vi "WVDIAL_2_OphirPM_v2.0.vi"() -> ()   [LabVIEW 2012]
uses:
  <vilib>/DAQmx/write.llb/DAQmx Write (Digital 1D Bool NChan 1Samp 1Line).vi
  <vilib>/DAQmx/miscellaneous.llb/DAQmx Fill In Error Info.vi
  under_development/AMCS_Data.vi
  <vilib>/Analysis/baseanly.llb/Mean (DBL).vi
  H2O_DIAL/LabVIEW-2012/Scalar_Data.vi
  H2O_DIAL/LabVIEW-2012/Bristol WM V2_31b/CLDevIFace.dll
  <vilib>/Analysis/NI_AALBase.lvlib
panel:
  out "AMCS_Profile":i32=68875
  out "FileHour":i32=2
  out "L_Count":i32=936
  out "sigma_off_total":dbl[](array[numeric])=[5.070497628289756e-25, 5.0334853455633925e-25, 4.99663547931583e-25, 4.959948279288469e-25, 4.923423990568222e-25, 4.887062852998473e-25, 4.850865100877033e-25, 4.814830962521382e-25, 4.778960659817837e-25, 4.743254407920139e-25, 4.707712414842624e-25, 4.672334881115004e-25, 4.637121999436925e-25, 4.602073954366994e-25, 4.56719092201873e-25, 4.532473069731469e-25, 4.497920555823106e-25, 4.463533529335168e-25, 4.429312129736619e-25, 4.395256486716884e-25, 4.361366720005691e-25, 4.327642939082048e-25, 4.2940852430644775e-25, 4.260693720490288e-25, 4.227468449179839e-25, 4.194409496090374e-25, 4.161516917187555e-25, 4.128790757307133e-25, 4.0962310500914247e-25, 4.063837817890729e-25, 4.0316110716857104e-25, 3.999550811045053e-25, 3.9676570240528366e-25, 3.935929687302844e-25, 3.9043687659042657e-25, 3.872974213418959e-25, 3.8417459719034525e-25, 3.8106839719420626e-25, 3.779788132663995e-25, 3.7490583617828527e-25, 3.7184945556449563e-25, 3.6880965993136353e-25, 3.6578643666610067e-25, 3.627797720389404e-25, 3.597896512186718e-25, 3.568160582829921e-25, 3.538589762243083e-25, 3.509183869681634e-25, 3.479942713816823e-25, 3.450866092902416e-25, 3.421953794902879e-25, 3.393205597627788e-25, 3.364621268922782e-25, 3.3362005668111493e-25, 3.3079432396620512e-25, 3.2798490263459325e-25, 3.2519176564454297e-25, 3.2241488504042248e-25, 3.196542319726317e-25, 3.1690977671553114e-25, 3.1418148868557824e-25, 3.1146933646267415e-25, 3.08773287808136e-25, 3.060933096826186e-25, 3.0342936826836184e-25, 3.007814289864978e-25, 2.9814945651963276e-25, 2.955334148264468e-25, 2.9293326716696813e-25, 2.9034897611789183e-25, 2.8778050359516556e-25, 2.8522781086960743e-25, 2.8269085858893675e-25, 2.801696067964473e-25, 2.77664014947359e-25, 2.751740419295918e-25, 2.7269964608086254e-25, 2.7024078520645357e-25, 2.677974165975873e-25, 2.6536949704675698e-25, 2.629569828657932e-25, 2.6055982990165753e-25, 2.5817799355364205e-25, 2.5581142878655634e-25, 2.534600901463837e-25, 2.5112393177860403e-25, 2.488029074350094e-25, 2.464969704946346e-25, 2.4420607397132765e-25, 2.4193017053199705e-25, 2.396692125036495e-25, 2.374231518868433e-25, 2.351919403683499e-25, 2.3297552932977987e-25, 2.3077386985828024e-25, 2.2858691275833926e-25, 2.264146085578557e-25, 2.242569075179679e-25, 2.2211375964275483e-25, 2.1998511468550746e-25, 2.1787092215687626e-25, 2.1577113133082336e-25, 2.136856912540202e-25, 2.116145507460489e-25, 2.095576584136337e-25, 2.0751496264925255e-25, 2.0548641163882025e-25, 2.0347195336705433e-25, 2.0147153562078706e-25, 1.9948510599408518e-25, 1.9751261189266903e-25, 1.9555400053748722e-25, 1.936092189678544e-25, 1.9167821404641924e-25, 1.8976093246186118e-25, 1.8785732073267435e-25, 1.8596732521063013e-25, 1.840908920841047e-25, 1.8222796738212876e-25, 1.8037849697802666e-25, 1.7854242659075025e-25, 1.7671970179325255e-25, 1.7491026801307859e-25, 1.7311407053680074e-25, 1.7133105451612698e-25, 1.6956116497139343e-25, 1.6780434679580535e-25, 1.6606054476291184e-25, 1.6432970353069002e-25, 1.6261176764671616e-25, 1.6090668155595419e-25, 1.5921438960726898e-25, 1.5753483606030133e-25, 1.558679650921211e-25, 1.542137208060544e-25, 1.5257204723895893e-25, 1.5094288837202545e-25, 1.4932618813705948e-25, 1.4772189042726048e-25, 1.4612993910873613e-25, 1.4455027802681816e-25, 1.4298285102037945e-25, 1.4142760193126855e-25, 1.39884474614635e-25, 1.383534129515875e-25, 1.3683436086077352e-25, 1.3532726230945627e-25, 1.3383206132699214e-25, 1.3234870201513542e-25, 1.3087712856189937e-25, 1.294172852522011e-25, 1.279691164815233e-25, 1.2653256676631938e-25, 1.251075807588225e-25, 1.236941032547358e-25, 1.2229207920724155e-25, 1.2090145373762662e-25, 1.1952217214575004e-25, 1.1815417992033117e-25, 1.1679742274812815e-25, 1.1545184652383437e-25, 1.1411739735782334e-25, 1.1279402158460732e-25, 1.1148166576893325e-25, 1.1018027671315384e-25, 1.0888980146189734e-25, 1.0761018730676202e-25, 1.0634138178949676e-25, 1.050833327058706e-25, 1.0383598810662664e-25, 1.0259929629764006e-25, 1.0137320584118708e-25, 1.0015766555315383e-25, 9.895262450187152e-26, 9.775803200441297e-26, 9.657383762269646e-26, 9.539999115734773e-26, 9.423644264312016e-26, 9.308314234034012e-26, 9.194004072774325e-26, 9.08070884940888e-26, 8.968423652704526e-26, 8.857143590515842e-26, 8.746863788487623e-26, 8.637579389020506e-26, 8.529285549996808e-26, 8.421977443551903e-26, 8.315650254725024e-26, 8.210299180224986e-26, 8.105919426962639e-26, 8.002506210665298e-26, 7.900054754557642e-26, 7.798560287932613e-26, 7.698018044712655e-26, 7.598423262105828e-26, 7.499771179237192e-26, 7.402057035772657e-26, 7.305276070650775e-26, 7.209423520744956e-26, 7.114494619701163e-26, 7.020484596631184e-26, 6.927388675157846e-26, 6.83520207218349e-26, 6.74391999695093e-26, 6.653537650085038e-26, 6.564050222691071e-26, 6.47545289560048e-26, 6.387740838606428e-26, 6.300909209843307e-26, 6.21495315514699e-26, 6.129867807642097e-26, 6.045648287278875e-26, 5.962289700535e-26, 5.879787140111133e-26, 5.798135684830717e-26, 5.717330399483455e-26, 5.637366334840297e-26, 5.558238527695597e-26, 5.479942001036147e-26, 5.402471764231797e-26, 5.325822813299969e-26, 5.249990131253825e-26, 5.174968688556138e-26, 5.100753443546731e-26, 5.0273393429923897e-26, 4.954721322724253e-26, 4.8828943082274503e-26, 4.8118532153859127e-26, 4.741592951231876e-26, 4.6721084147336384e-26, 4.6033944976566704e-26, 4.535446085450234e-26, 4.468258058186193e-26, 4.401825291523709e-26, 4.33614265769571e-26, 4.2712050266026124e-26, 4.207007266850279e-26, 4.1435442468571613e-26, 4.080810836010187e-26, 4.018801905846338e-26, 3.957512331230703e-26, 3.896936991600012e-26, 3.837070772243326e-26, 3.777908565561996e-26, 3.719445272431421e-26, 3.661675803546137e-26, 3.604595080840441e-26, 3.548198038889937e-26, 3.4924796264223826e-26, 3.4374348078418457e-26, 3.383058564773786e-26, 3.3293458977389997e-26, 3.2762918278031975e-26, 3.2238913983477067e-26, 3.172139676902159e-26, 3.121031757036547e-26, 3.070562760379313e-26, 3.0207278387203887e-26, 2.971522176188582e-26, 2.922940991630198e-26, 2.8749795410476525e-26, 2.827633120249765e-26, 2.7808970676362635e-26, 2.7347667671897224e-26, 2.689237651659654e-26, 2.644305206012318e-26, 2.599964971092499e-26, 2.556212547611665e-26, 2.5130436004126895e-26, 2.4704538631119164e-26, 2.428439143089101e-26, 2.3869953269207577e-26, 2.3461183862372208e-26, 2.3058043840965564e-26, 2.2660494818532045e-26, 2.2268499466380175e-26, 2.1882021593865282e-26]
  out "sigma_on_total":dbl[](array[numeric])=[3.516166046138097e-23, 3.5157907452847906e-23, 3.51513468971426e-23, 3.514196959161098e-23, 3.512976736015344e-23, 3.511473306185464e-23, 3.5096860601118775e-23, 3.507614493860602e-23, 3.5052582098874735e-23, 3.502616917541285e-23, 3.4996904342273037e-23, 3.4964786854780294e-23, 3.4929817057676835e-23, 3.4891996387279024e-23, 3.485132737348183e-23, 3.480781364691122e-23, 3.476145993029859e-23, 3.4712272049844286e-23, 3.466025692277867e-23, 3.460542256602056e-23, 3.454777808431937e-23, 3.4487333671672725e-23, 3.442410060646205e-23, 3.4358091240077325e-23, 3.428931899736903e-23, 3.421779836333299e-23, 3.414354487615683e-23, 3.4066575119381957e-23, 3.3986906707513384e-23, 3.3904558278202657e-23, 3.38195494740876e-23, 3.373190093797025e-23, 3.3641634290981605e-23, 3.3548772119364244e-23, 3.345333796241224e-23, 3.33553562899499e-23, 3.325485248768654e-23, 3.31518528399112e-23, 3.3046384509497314e-23, 3.2938475515200476e-23, 3.282815471712371e-23, 3.271545178971963e-23, 3.260039720401316e-23, 3.248302220230674e-23, 3.236335877827104e-23, 3.224143965253366e-23, 3.2117298246742885e-23, 3.199096865914817e-23, 3.18624856457891e-23, 3.1731884585195093e-23, 3.1599201461816614e-23, 3.14644728350361e-23, 3.1327735813913904e-23, 3.118902803167363e-23, 3.104838761691913e-23, 3.0905853167689533e-23, 3.0761463727388826e-23, 3.0615258751451924e-23, 3.0467278083049304e-23, 3.031756192772461e-23, 3.0166150822926897e-23, 3.001308561059991e-23, 2.985840741286183e-23, 2.9702157600649176e-23, 2.9544377769578504e-23, 2.938510971087036e-23, 2.922439538548865e-23, 2.9062276897463107e-23, 2.88987964664322e-23, 2.8733996404482916e-23, 2.856791908519729e-23, 2.840060692109546e-23, 2.823210233938355e-23, 2.8062447754046733e-23, 2.7891685544356736e-23, 2.771985802876922e-23, 2.754700743927475e-23, 2.7373175906154254e-23, 2.71984054232944e-23, 2.702273783786046e-23, 2.684621481765235e-23, 2.6668877840748917e-23, 2.649076816398387e-23, 2.6311926811665514e-23, 2.6132394550121815e-23, 2.595221187261574e-23, 2.5771418977050947e-23, 2.5590055752041554e-23, 2.5408161756800332e-23, 2.522577620551517e-23, 2.5042937953267503e-23, 2.4859685474964716e-23, 2.4676056859152064e-23, 2.449208978537404e-23, 2.4307821515438647e-23, 2.4123288880546024e-23, 2.3938528266275293e-23, 2.375357560379023e-23, 2.3568466357933387e-23, 2.338323551597007e-23, 2.3197917579690722e-23, 2.3012546551776264e-23, 2.2827155936328393e-23, 2.2641778719258197e-23, 2.2456447370872583e-23, 2.2271193832897603e-23, 2.2086049516775996e-23, 2.1901045294566413e-23, 2.1716211494842488e-23, 2.153157789996697e-23, 2.1347173738731588e-23, 2.1163027687270315e-23, 2.097916786360134e-23, 2.07956218227752e-23, 2.061241656256252e-23, 2.0429578512033775e-23, 2.0247133540629775e-23, 2.006510694942393e-23, 1.9883523476865673e-23, 1.970240729431415e-23, 1.9521782011719382e-23, 1.934167067561686e-23, 1.9162095771558377e-23, 1.8983079226880006e-23, 1.880464240994691e-23, 1.8626806138283133e-23, 1.8449590676178742e-23, 1.8273015741880447e-23, 1.8097100507455573e-23, 1.7921863607252917e-23, 1.7747323138362434e-23, 1.7573496666605283e-23, 1.740040123053841e-23, 1.722805334930093e-23, 1.7056469022044368e-23, 1.6885663739791132e-23, 1.671565248534023e-23, 1.6546449743297844e-23, 1.6378069503914255e-23, 1.6210525269221011e-23, 1.604383005998786e-23, 1.587799642145069e-23, 1.571303643051848e-23, 1.554896170175491e-23, 1.53857833954368e-23, 1.5223512221160605e-23, 1.506215844867706e-23, 1.490173191356572e-23, 1.4742242021808207e-23, 1.458369776070558e-23, 1.4426107704149258e-23, 1.4269480019244374e-23, 1.4113822474190837e-23, 1.3959142446739708e-23, 1.3805446929672297e-23, 1.3652742538129026e-23, 1.3501035518651393e-23, 1.335033175471664e-23, 1.3200636774045514e-23, 1.3051955758103955e-23, 1.290429354596179e-23, 1.2757654643750209e-23, 1.2612043231262256e-23, 1.2467463168547449e-23, 1.2323918004591888e-23, 1.2181410981178614e-23, 1.2039945043564175e-23, 1.1899522845279472e-23, 1.1760146755511953e-23, 1.1621818864405649e-23, 1.1484540993290901e-23, 1.1348314697827357e-23, 1.1213141275614906e-23, 1.1079021773658707e-23, 1.0945956993350662e-23, 1.0813947499162843e-23, 1.0682993621158443e-23, 1.0553095464443556e-23, 1.0424252914291965e-23, 1.0296465640364806e-23, 1.0169733106187996e-23, 1.0044054570976238e-23, 9.919429098867016e-24, 9.795855561937457e-24, 9.673332646628335e-24, 9.551858860010187e-24, 9.431432533872387e-24, 9.312051830803365e-24, 9.193714748143824e-24, 9.076419125045633e-24, 8.960162645828894e-24, 8.844942844499155e-24, 8.730757111818061e-24, 8.617602697299562e-24, 8.505476715326103e-24, 8.394376148894811e-24, 8.28429785474724e-24, 8.175238567297419e-24, 8.067194902841032e-24, 7.960163362989318e-24, 7.854140339751279e-24, 7.749122119445534e-24, 7.645104885867197e-24, 7.542084723743027e-24, 7.440057623402108e-24, 7.339019484335796e-24, 7.238966117429662e-24, 7.139893249972184e-24, 7.041796528033791e-24, 6.944671519436088e-24, 6.848513717840699e-24, 6.753318545523783e-24, 6.659081355525225e-24, 6.565797436329607e-24, 6.473462012991977e-24, 6.382070250797694e-24, 6.291617257696864e-24, 6.202098086956149e-24, 6.1135077405262306e-24, 6.0258411699439036e-24, 5.939093280105205e-24, 5.853258931100218e-24, 5.7683329402744104e-24, 5.684310085466258e-24, 5.601185105691751e-24, 5.518952704737261e-24, 5.437607551764278e-24, 5.3571442845088725e-24, 5.277557511186432e-24, 5.198841810779709e-24, 5.120991736926645e-24, 5.044001818760121e-24, 4.967866561988263e-24, 4.892580451868829e-24, 4.818137953743617e-24, 4.744533515043554e-24, 4.671761567206439e-24, 4.599816526130568e-24, 4.528692794421368e-24, 4.4583847623727855e-24, 4.388886810069044e-24, 4.320193307151974e-24, 4.252298615419794e-24, 4.185197089827738e-24, 4.118883078938342e-24, 4.053350926789436e-24, 3.988594973802574e-24, 3.9246095576720925e-24, 3.861389014400184e-24, 3.7989276796219265e-24, 3.737219888905301e-24, 3.6762599794970055e-24, 3.6160422905656756e-24, 3.55656116454113e-24, 3.497810947330621e-24, 3.439785989889431e-24, 3.382480648098059e-24, 3.325889284547815e-24, 3.270006268380975e-24, 3.214825976428064e-24, 3.1603427936015446e-24, 3.1065511140889573e-24, 3.053445341163424e-24, 3.001019888590546e-24, 2.9492691804210446e-24, 2.8981876524496178e-24, 2.847769751738098e-24, 2.79800993813206e-24, 2.7489026837790565e-24, 2.7004424745716544e-24, 2.652623809775478e-24, 2.6054412029477065e-24, 2.5588891822439123e-24, 2.5129622908274716e-24, 2.4676550873679846e-24, 2.4229621459967116e-24, 2.3788780572043868e-24]
  out "background start":u32=269
  in  "Tab Control 2":enum32{"WV ND far", "WV ND near"}(tab)
  out "Water Vapor Number Density":dbl[][](graph)=[[1.5992131155180653, 1.6082257408100515, 1.6172404192617005, 1.5682940115340778, 1.4382631922991003, 1.4566513161926358, 1.6624857596079967, 1.604530318531669, 1.3653234601107795, 1.2397847200272387, 1.2182284851114118, 1.2594618273623515, 1.2757220359952972, 1.231794919996768, 1.1984238773092097, 1.0511941569175325, 0.947177179813774, 1.3213587629249737, 1.4068153237738503, 0.9935374495138973, 0.7599198342010364, 0.6628288993150979, 0.6698286610956209, 0.8385968849843203, 0.9265576864824148, 0.7974532453710999, 0.7815643341063747, 0.7189784837938722, 0.5208097189885875, 0.2535027201514644, 0.4186197260233687, 0.8935310957648346, 0.4569807618660739, 0.25298622943586235, -0.3980630535463325, -2.133807038662934, -2.606639636741421, -3.9154695882450983, -8.219471908587723, -10.050453359526605, -3.4968101624851693, -3.2729400219950566, -3.163884070486512, -2.4309470851928605, -0.5833929948890328, 0.06247920983003045, -0.9129852004503765, -0.7315712531026931, -0.30164757420753013, -0.6177145499916912, 0.05774264779438736, 0.6842875121661679, 1.4740113495484077, 0.697544982479824, -1.049981924326516, -0.8196574068354904, 0.510148279490742, 0.21464861075793903, -0.31714560207329967, 0.006887828569203875, -0.30407504105215905, -0.20010859267721784, -1.221138706669891, -0.04661851813208892, 1.5284195002773824, 0.0260232816898901, -0.520857938764628, -0.08492917434350651, 0.604187732093999, 0.73543759309028, 0.6308713001702517, -0.18461931416174024, -0.641552498246701, -0.9215208222409633, -1.0892550092701596, 1.2442835676945807, 2.173314646621063, 0.9369534608442799, -0.792885950953008, -1.1531494944579526, -0.15905319487357858, 0.8176028380172045, 1.1612952959671206, 2.617387230232414, 2.015404900631263, -0.4303147992033666, -0.7796608509634929, -0.10067409378849432, -0.3694516626487272, 0.730107477279339, 0.37322824802492466, -1.6742234572486923, -1.036253896298939, -1.6680330853214775, -0.9716921094813229, 0.06454577965723993, -0.07817305102869904, -0.7332562405584276, 1.8159065003832369, 2.4971988578262545, -0.27693900780234415, 4.098424126129518, 1.9148579130151497, -1.8281665525227517, -2.3804143706043144, 0.3092823814280153, -0.49065459076649065, -0.34898078933322085, 1.2553996836583532, 0.11445370205265852, -1.5928775278553056, -3.6617633065604367, -1.7636166748987094, -0.2880075426855823, 1.7560526808900407, -0.2512189459596313, -0.3287850652593397, 0.8208825793059632, 1.044251631009513, -0.06848876471766958, 0.706626715240254, -1.3322554497053207, 2.1908219922192615, 9.331622435071264, 2.849767805860485, 3.513601642618711, 2.309109033176175, 5.100110065656176, -2.305506196889784, -1.0851253092088786, 2.1439019584318526, 3.111549499967813, -1.002045501523791, -6.733749565128037, 1.243909744708835, 2.064440733646956, -1.2701440070751369, -5.4628386135729325, 3.3917878618854673, 9.521303672264951, -0.5084767308845132, -0.05512797558414156, 12.922056854770483, 2.7383986133981355, -5.799654080917452, -13.877589166980687, -5.53890167405428, 3.110441098528859, -1.7133359853030656, -10.487457505690932, 5.222912870877752, -3.7373060146953523, -21.861987195132567, -5.308588265909625, 0.9116820151696693, 8.993600924878596, 4.185979422457073, 1.0845074378859085, -1.8910834021656124, -1.5746296913749636, 4.306022618247472, 3.997958103320701, 7.93554204893104, -3.684280000966452, -8.424392762667392, -5.77219986630512, -2.3453953126740634, -5.766772069385087, 4.17298472258335, 3.5826829653229293, -9.190201621067096, -1.0829815607679063, -1.682589248661155, 13.874443095893445, 4.3866530582639705, 16.11064454311473, 17.78879632267084, 12.011208447047938, -5.260899169337218, -7.4866580190818866, -14.699964054590536, 2.7256753738889627, -7.159808903092408, -40.059798644383065, 10.941886052200935, -26.89298479919689, -28.06184835098003, -20.43347977213505, -4.406709706394973, -1.8407735993912404, 8.810705572452946, 15.789352328361959, 2.554121964743826, 12.1962206668947, -15.099300151730803, 13.019777626127185, 26.143487506459437, 15.112075103913178, -4.566333162000295, 4.703673483038427, -1.9604286278257814, -22.477442176801777, 11.237707198763124, 25.90063719494314, 16.397524232625667, -1.637893029433272, -11.255055728055169, -28.732727310685455, -20.490465992738148, 9.615150980796496, 12.68857300996426, 18.16933227624077, 14.520051089280647, -5.646874057069329, 0.40197008760169967, 20.2177608324192, -31.760449757613948, 13.215305675945084, 23.298804318146267, -32.646100448424825, -3.1598248666074613, -8.40542451017114, -3.3560341338387953, 29.35382069433968, -25.04630218293011, -13.507505089357831, -13.922338316207165, 6.15334141001665, -10.360985562260492, 28.923205139605535, 8.694480650748346, -16.057475063525434, 36.919584558543015, -13.423711644791421, 39.996568023931324, -16.55455537984995, 6.809952333760757, -7.20484250819715, 23.06954136236042, 39.58479818950455, -17.99911903544103, 5.890677341163354, -60.034189646412095, -21.786588583324534, -51.914763721371045, 40.661987400676836, 26.225049000292202, -34.112626888694464, -39.797026603236304, -67.10976626173382, -5.113708731880433, -49.7213926330504, -18.062560466122466, 85.38084621901817, -23.691191412149227, -7.881934268930171, 63.29577386065949, 24.052597030707947, -20.43551776172326, 132.2828290748101, 39.4757334452027, 55.7151516560583, -23.806902559982316, -75.5252149839331, 70.36337238869856, 94.82852884165652, -82.81021633454347, 12.893729544398322, -26.84837020288986, -60.81708823090221, -39.17993688985304, -13.378858268915783, 37.953224707869225, -16.19763515356616, -29.108263916519956, -124.93982671437738, 0.0, 0.0, 0.0, 0.0]]
  out "Water Vapor Number Density 2":dbl[][](graph)=[[1.5364130113793415, 1.518337489157193, 1.520390998062569, 1.556767034818283, 1.561107486940302, 1.5564802719193571, 1.6381438265816557, 1.501563316682888, 1.2292446720753658, 1.18064949906327, 1.2072274468822595, 1.2275182502054294, 1.2727095492709266, 1.2129762431126005, 1.1245595858175887, 1.02161468124156, 0.9927211557756013, 1.4320153948984997, 1.5061236129201165, 1.040214125246526, 0.7745680406160396, 0.6534685372617243, 0.6999783116040139, 0.7861560859454928, 0.7809087050195085, 0.727799697364269, 0.746909724600615, 0.7971092161296583, 0.40553259283535176, 0.01613853483237202, 0.2058601557879657, 0.12053797086574508, -0.02020158762419371, 0.06527616385373658, -0.6347082947562561, -2.0643629823265455, -2.9845901222078335, -5.145604151721974, -6.748015683547248, -3.7685317770029907, -3.34533331126462, -2.9872900066566688, -2.6758227938189725, -1.7932635435202542, -0.8949735037482576, -0.8200012571692603, -0.13682264648337022, 0.2931977072594, -0.05698793384208824, -0.3224880867074141, -0.11524687828656995, -0.1788695014063217, -0.19025205177511265, 0.012926056004201238, -0.6277162703713939, -0.8922551089115862, -1.1334406535777133, -0.9461302928201699, -0.3168485004641039, 0.268767685858386, 0.28559527092386766, -0.13538304531121997, -0.04237770041577783, -0.023399515410177357, 1.1157410601639124, 1.2482750531968756, 0.7958671042399825, 0.34827129055460804, -0.5014270960529756, -0.7927073011228699, -0.511240289149088, -0.11791264053508158, 0.2420693689689032, 0.2137538761092436, -1.5931871111776896, -1.4220036751918483, 0.0235219114797506, 1.7421075643216557, 1.6432774713882652, 0.6321158852755421, 0.27215593630840884, 0.06807951216103945, -0.5456678171301241, -0.7815692803223797, 0.6275724518932578, 0.27517653867500025, -0.444506510114721, -1.2330716818477265, -0.13086648735003015, 0.3259486674374053, 0.04240287015581609, 1.1654964341416485, 0.7519854734562245, 0.7141108280831628, 0.8488902389421702, 0.8298293562028988, -0.30894789354783786, -1.12530687327123, -0.1478070819209756, 0.9858160437767299, 0.7750186672950592, 0.6108763122901893, -0.14121494435094706, -1.2642069595379943, -0.35713973453174835, -0.4031134561301113, -1.576138495989707, -1.038841182482667, -0.1928514921881704, -2.6034850828806184, -3.7154313945317927, -5.313334178231977, -0.8917503831211164, 2.223977767075163, 0.4871323439767443, -2.3274363575798107, 1.0704190904659991, 3.990521818638429, -0.8398164977279448, 2.7105795336840592, 4.601483331593351, 3.5149673225037716, 0.8990366427771173, 2.2125259583813297, 2.3166980827134824, 5.725774100618085, 2.8364971034247017, -2.5078911292129753, 0.2506085763683534, -1.3073165403302751, -1.4735434630012858, -1.3246230011748195, -3.3265875819766584, -6.081437709602098, -3.1713696664778235, -3.821424059913203, -2.4079480376962152, 2.7122997464347733, -0.4012787716328172, -1.6660387722422796, -2.8883298019759622, 1.583008030545662, 8.683114563228083, 10.230517516040909, -0.4958975601136249, 2.8813077819771102, 3.625276173741331, -2.840541261698016, -0.6053599352493296, 2.1441948493950482, 6.466736863936187, 0.2608467982783902, -3.8177527279633554, -5.6914259723937874, -1.4359348338625717, -3.004659151138894, -4.6914097216194754, 1.0083878383431153, 4.739440029394087, 0.06886551002808773, -2.485849280291415, 4.65498881925389, 7.801295615519863, 2.6547227868290895, 8.996315788153266, 1.929973280459837, -1.4172050913150493, 0.6156159950160424, 1.2936423902948462, 3.2285093129371596, 0.32204146956322977, -4.1108233226260245, -6.506413000854209, -4.911723091198433, -13.141929692253491, -6.3977876365384745, 8.616388465474579, 16.51371740907324, -7.1988931514972, -10.553923078163223, -12.307641308423447, -6.5697288376189835, -5.044623651384795, -13.808438208567816, -2.425144986156166, 5.400445627008468, 2.267531069243815, -17.257334276896696, -8.950527418563968, 5.703973433707766, 14.939577492212859, 21.595849939589044, -9.851732971822114, 17.17547031217899, 9.806979152667655, 20.20186441259229, 1.976249509706074, -4.552324226015481, 7.670997760036694, 22.717836142749398, 15.728369988698287, 13.297780916019025, 22.704048183168776, -11.77196022467062, -14.947622700887818, -9.058359300858323, -0.7082321311117581, 3.2172514486542094, 14.699799656085345, -28.32299461926606, -8.266322339282022, -11.902651622162375, -18.733040377231333, -11.409939624479723, 32.28757119464318, 3.42137124257041, -3.1268353184493938, 11.18700848144839, -3.3359401699727584, 5.0092913080631005, -6.365614099587739, -20.388474455127188, -0.6018044775915197, 19.729541678869182, 3.3391712612817845, -28.65533859839855, -22.47922904710733, -38.673044137935726, -28.471841305595238, -4.335580114906128, -24.63003692117338, -34.16022113076511, -19.05945088654873, 5.782474230064923, -29.66949474051266, -13.271540111384867, -6.570141734253886, 6.6246451035020195, 10.987346568975623, 43.59236203202549, 7.2310434492700235, 50.35355833882173, 3.2493293592923687, -29.827301167932877, -26.579368830155776, 13.378383332241294, 16.44736247852381, 43.942199391517484, 19.15753541202371, -76.54840433881071, 24.075567112876836, -24.501666960145464, 29.583695883450805, 51.633971547504146, 65.0169036784934, 28.137206072052717, 13.077137255123715, -4.3911378030089585, -13.286995683876434, 39.72390515889458, -58.46394305649631, -35.05269948224503, -35.501083671422364, -53.17327104429747, -5.753557970712993, -49.876470893489724, -18.47853213614708, -40.42031030978713, -9.338008653877434, -31.795543307360436, 55.7002918087253, 55.79470085384945, 39.48367009008215, 35.13953970858524, -15.931364372720266, 44.460085088302236, 0.0, 0.0, 0.0, 0.0]] caption="Water Vapor Number Density"
  out "RingBuffer offline near":dbl[][](array[numeric])
  out "RingBuffer aerosol near":dbl[][](array[numeric])=[[2382.6, 2697.6, 2843.6, 3137.6, 4025.6, 3802.6, 2176.6, 1092.6, 1987.6, 4591.6, 6038.6, 6777.6, 6483.6, 4982.6, 3675.6, 3236.6, 3392.6, 3540.6, 3398.6, 3986.6, 4735.6, 3674.6, 2084.6, 721.6, 292.6, 285.6, 230.6, 173.6, 221.6, 330.6, 441.6, 457.6, 447.6, 631.6, 1010.6, 1159.6, 685.6, 426.6, 321.6, 204.6, 70.6, 20.6, 8.6, 1.5999999999999996, -4.4, -2.4000000000000004, 5.6, -2.4000000000000004, 4.6, -7.4, -0.40000000000000036, -5.4, 3.5999999999999996, -5.4, -7.4, -0.40000000000000036, 0.5999999999999996, -1.4000000000000004, 1.5999999999999996, -1.4000000000000004, -4.4, -0.40000000000000036, -3.4000000000000004, -3.4000000000000004, -4.4, -3.4000000000000004, 4.6, 1.5999999999999996, -2.4000000000000004, 1.5999999999999996, 1.5999999999999996, 4.6, 1.5999999999999996, 1.5999999999999996, 2.5999999999999996, -3.4000000000000004, -0.40000000000000036, -0.40000000000000036, -7.4, -3.4000000000000004, -0.40000000000000036, 4.6, -4.4, 0.5999999999999996, -1.4000000000000004, -3.4000000000000004, 0.5999999999999996, -2.4000000000000004, 3.5999999999999996, 0.5999999999999996, 2.5999999999999996, -3.4000000000000004, 3.5999999999999996, -5.4, 2.5999999999999996, 1.5999999999999996, -4.4, -4.4, 2.5999999999999996, 1.5999999999999996, 2.5999999999999996, 1.5999999999999996, 1.5999999999999996, -7.4, 1.5999999999999996, -2.4000000000000004, 0.5999999999999996, -5.4, 0.5999999999999996, 3.5999999999999996, -2.4000000000000004, -7.4, -1.4000000000000004, -1.4000000000000004, -5.4, -1.4000000000000004, 0.5999999999999996, -1.4000000000000004, 0.5999999999999996, -5.4, -4.4, -0.40000000000000036, -5.4, 0.5999999999999996, -3.4000000000000004, -1.4000000000000004, 0.5999999999999996, -1.4000000000000004, -1.4000000000000004, 0.5999999999999996, 2.5999999999999996, -0.40000000000000036, -6.4, -0.40000000000000036, -6.4, -4.4, 2.5999999999999996, -3.4000000000000004, -0.40000000000000036, 0.5999999999999996, -5.4, -4.4, -2.4000000000000004, -3.4000000000000004, -7.4, -2.4000000000000004, 3.5999999999999996, -0.40000000000000036, 1.5999999999999996, -1.4000000000000004, -3.4000000000000004, -1.4000000000000004, -3.4000000000000004, 1.5999999999999996, 5.6, -1.4000000000000004, -1.4000000000000004, 5.6, -1.4000000000000004, -2.4000000000000004, -4.4, 0.5999999999999996, -1.4000000000000004, -2.4000000000000004, -5.4, -5.4, 1.5999999999999996, -5.4, -3.4000000000000004, -5.4, -2.4000000000000004, -5.4, -6.4, -4.4, -3.4000000000000004, -0.40000000000000036, -1.4000000000000004, -2.4000000000000004, -6.4, -1.4000000000000004, 2.5999999999999996, -1.4000000000000004, 2.5999999999999996, 5.6, 4.6, 0.5999999999999996, -4.4, -2.4000000000000004, 0.5999999999999996, -2.4000000000000004, -0.40000000000000036, -1.4000000000000004, -1.4000000000000004, 0.5999999999999996, 0.5999999999999996, 0.5999999999999996, 5.6, 1.5999999999999996, -2.4000000000000004, 2.5999999999999996, -5.4, -0.40000000000000036, 0.5999999999999996, -1.4000000000000004, -4.4, -3.4000000000000004, -1.4000000000000004, -2.4000000000000004, -2.4000000000000004, -0.40000000000000036, -3.4000000000000004, -3.4000000000000004, -2.4000000000000004, 2.5999999999999996, -1.4000000000000004, 5.6, -3.4000000000000004, -2.4000000000000004, 0.5999999999999996, -1.4000000000000004, 0.5999999999999996, -5.4, 0.5999999999999996, -6.4, -0.40000000000000036, -5.4, 0.5999999999999996, 0.5999999999999996, 8.6, 1.5999999999999996, -0.40000000000000036, -3.4000000000000004, -3.4000000000000004, 0.5999999999999996, -2.4000000000000004, -2.4000000000000004, -6.4, -3.4000000000000004, -3.4000000000000004, -1.4000000000000004, 2.5999999999999996, -3.4000000000000004, -1.4000000000000004, -3.4000000000000004, -3.4000000000000004, -2.4000000000000004, -2.4000000000000004, 1.5999999999999996, -7.4, -6.4, -4.4, -0.40000000000000036, -0.40000000000000036, -0.40000000000000036, -4.4, -5.4, -1.4000000000000004, -2.4000000000000004, -4.4, 6.6, -1.4000000000000004, 0.5999999999999996, 2.5999999999999996, -3.4000000000000004, -0.40000000000000036, 3.5999999999999996, -3.4000000000000004, 2.5999999999999996, -5.4, 1.5999999999999996, 0.5999999999999996, -2.4000000000000004, -1.4000000000000004, 1.5999999999999996, 1.5999999999999996, 0.5999999999999996, 0.5999999999999996, -0.40000000000000036, -2.4000000000000004]]
  in  "LOWER DISPLAY TAB":T1(tab)=enum."Raw Counts far"
  out "NRB":dbl[][](graph)=[[-3.739841376821264, -3.148111997969907, -2.8053201900405846, -2.4720283981738125, -2.2220361062039857, -2.1624941227636123, -2.2596934733921055, -2.1357303164235213, -1.6917041934233819, -1.3691989209887527, -1.1576363880704834, -1.0291107137638036, -1.0052600046420344, -1.0397129725062237, -1.0384028135023908, -0.9519858474845082, -0.8454239717927076, -0.7641788963246816, -0.6644779477624746, -0.5354162701784232, -0.4868695967293412, -0.5872496631273286, -0.848695128061842, -1.2608662111155369, -1.4732078684705003, -1.4690139900772856, -1.5446868005495193, -1.5048285927516476, -1.3465772854760274, -1.1700462347927176, -1.0570455424154432, -0.9928439277866905, -0.8831468540601666, -0.677792072205639, -0.5471488995830269, -0.5906765228582762, -0.7934541078663532, -0.9917126986266663, -1.0727561222562487, -1.303794944751113, -1.7988220766703165, -2.4430222256888485, -2.928555581752763, -3.29394444921866, -3.6424079877548867, -3.3600775241079655, -3.1786717810361544, -2.9495348706920352, -2.855238446439066, -2.914077336771172, -3.2704528352752407, -3.016215942676994, -3.1322980629894563, -4.262195139097215, -4.246257279754664, -3.6285450064507736, -3.437083303960591, -4.200126671617277, -3.2310329121095642, -3.2164344346265654, -3.5542613904416402, -3.100809808474606, -4.128301559835989, -2.835862681978818, -2.6387483057572134, -3.485833189379437, -4.074833053341498, -2.915831976778562, -3.0950387539193422, -4.036786578714638, -2.983076490032963, -2.8082025040450525, -3.222187295064662, -3.2103695758436217, -3.198710488522174, -2.819222617629452, -2.8078683518460705, -2.664033424565632, -2.4693208364620416, -2.9665569614099656, -3.910012620985852, -3.899354953975718, -3.8888264739910037, -3.276362488339411, -3.868144807314566, -3.0798361128184384, -3.8479441535059147, -2.7966278431707763, -2.786813174181288, -3.040347996426924, -3.0307502306633864, -2.3844416907520993, -2.233725509365601, -2.458514084558427, -3.771535448165456, -3.1603785943840372, -2.4312263232253346, -2.422317640372835, -2.694322798276014, -2.9488330153055737, -2.514224749342304, -3.7097823152193166, -3.0992466110528296, -2.4888008183100285, -2.2696387473033335, -2.0635999268959293, -2.2532497900727906, -2.6187456764972143, -3.050068064581927, -2.6028078171546634, -2.0800454489001563, -3.628546613402788, -2.6665800484270132, -2.571783484798168, -2.283374111050601, -2.106714628042256, -2.1756456219508866, -2.2610057771455736, -2.160923422658148, -2.0123289143782213, -2.5200224468382135, -2.3501478355580927, -2.2249595688790285, -2.5858935650693824, -3.5331626327270387, -2.4848520972359878, -2.1971623498459105, -2.471173248175377, -3.5058032381446536, -2.176883087144151, -1.8796690661139412, -2.531589072982153, -1.835812237540614, -1.8293059227451702, -2.086095845222006, -2.681755198565139, -2.8514799261503607, -2.243109324105116, -2.118740191249634, -2.230611425551113, -2.01357912013245, -2.6442563265394607, -2.37492111254099, -1.9189056223055938, -2.082033787287875, -3.3982769471742773, -3.392347989246799, -1.971493914653295, -1.9656448086186618, -1.9598348273318473, -1.8127375118871323, -1.871943430606548, -2.1534846352723918, -2.3105517457981875, -1.9313539491026268, -1.9257681487342866, -2.131068192089122, -2.2882790135622684, -2.5460387666646707, -2.277353222159264, -2.711269308399475, -2.3537069063085907, -2.261217978663198, -2.2559054913757177, -2.513865126877761, -1.9645536156777144, -1.8665844031480432, -1.7850120430443674, -2.067094087680242, -2.224695344714566, -1.7696383857117857, -1.840960451628112, -1.9286775855002336, -2.0417690003423896, -2.0367913995350007, -3.235957323114852, -2.084903269467421, -1.9473826253288045, -2.2670308734340665, -2.012322486700977, -1.7202734567577243, -1.7918745694730602, -2.6000188810023155, -2.0512141561719615, -2.4144895584995463, -1.9838416084717567, -2.1419099743981156, -1.8564540932304647, -1.8518461834113362, -3.1694754568374934, -2.5628543259677192, -3.1603802013360522, -2.553806442447627, -2.1099897276106616, -1.7319481227181737, -1.9383553541946372, -2.096660735147928, -1.7186869649201475, -1.7143111926237964, -2.083533196143151, -2.342440900464596, -3.116279919849904, -2.0706011116446876, -1.6927570105914123, -1.6885096233317012, -2.0578587467328067, -2.053652496557278, -1.8867408269820662, -1.8825749246854813, -1.760331202289986, -2.3002681047101885, -2.296161293448071, -2.0288339805936384, -3.06615511204477, -2.4600441406319633, -2.016685685169252, -2.0126737197740545, -3.050069671533942, -1.631129115762973, -1.5507852448516808, -1.9968086401008922, -1.7120638428565473, -1.367629563265811, -1.4701953698051455, -1.466326370250746, -1.6965529134630226, -1.9735414730848682, -1.6889000977569169, -3.0073116940633757, -1.8573941301558488, -2.3976971006788856, -2.0417609656120534, -2.9922708166911134, -1.6663380769375389, -1.943457462927641, -1.6589457858176113, -1.4861339144758856, -2.9738287446301275, -2.970186856846876, -1.7624450134843772, -2.184798930155837, -1.5443866134823474, -1.6335572445611999, -1.6299901390803655, -1.6264376230287596, -2.9451124445363934, -2.94158875222382, -2.3360176988107417, -2.3325223662717014, -2.931102641399076, -2.325573617501098, -2.146031933742486, -1.5985287494061886, -1.7711823689511583, -2.311840699595264, -1.2977317268017707, -1.4921510987806208, -1.862353775544653, -1.6962679687450855, -1.8556464915294777, -1.5714887770812624, -1.3990280238566024, -1.8456816904915978, -1.8423853337314515, -1.8391014395974978, -1.7310865289289006, -1.727827279461884, -2.2686514724055966, -1.8260886274662975, -1.449289817125235, -2.258982478714363, -1.9035991273254553, -1.5324444976763123, -2.8514815331023757, -1.8940715477333274, -1.6990316380605992, -1.3796154809140275, -inf, -inf, -inf]] caption="Water Vapor Number Density"
  out "NRB 2":dbl[][](graph)=[[-3.3138728309802596, -2.67333414094971, -2.2872446356915392, -1.957101572046068, -1.7236275596231185, -1.6853331752552108, -1.8180720457627246, -1.72825806141245, -1.290633504502973, -0.9840259369938127, -0.8163504750141714, -0.7251984318702619, -0.72186042712421, -0.7841700095118289, -0.8249439632711958, -0.7875081616148522, -0.7148765714866753, -0.664843831506477, -0.5900925435426341, -0.4710613963323042, -0.4450203164247589, -0.5734326258620402, -0.8518878294675268, -1.2598163106137872, -1.46910702385855, -1.4844002693597458, -1.558021420514424, -1.5362267439536783, -1.3602146003476414, -1.1847802803606045, -1.0899681774337695, -1.059493687028336, -0.9561277218271328, -0.7469643291310749, -0.5998578324715791, -0.6463714213061379, -0.8436179520482209, -0.9932063671074317, -1.1238688065214002, -1.383784411413848, -1.842286162898628, -2.316066939444091, -2.7524418242450515, -3.2939364143099423, -2.889072286306479, -3.1973245148547935, -3.1786444623465067, -3.3230866079937815, -3.20044960722529, -2.737973222170736, -2.849436273828795, -3.34071899925205, -3.32417394732007, -2.4560183789995143, -2.6551878518542855, -4.230588927931571, -3.613156886282499, -4.2001089948180965, -4.185260958659683, -2.7082741252573808, -2.7761021052087407, -2.863434430004854, -2.596816214950003, -2.523553282874999, -2.5100865175570624, -3.3097242534591675, -2.5834440405143186, -3.459888772215009, -3.447208416152971, -2.8326440981894283, -2.533076948477821, -2.5209286530534345, -2.79619445797703, -2.666275819642734, -3.3747840708440817, -2.6865906244397793, -3.3519251472825182, -2.3517240254618126, -2.199334716339299, -2.642037835017475, -2.587769221347387, -3.8993372771765378, -2.6100616242492145, -3.2763480255037183, -2.4879239238016893, -2.711844864795182, -2.893687181284411, -3.0598467802425677, -2.5059592458148607, -2.614355159339292, -3.2068238129852946, -3.799389327252861, -2.835759789413778, -2.6345860600829196, -2.4492920485269907, -2.6162993012031803, -2.1099832998145005, -2.7902735351366585, -2.4134688699095865, -2.4047392591046863, -2.396096511539401, -2.5056398346941067, -2.2389021766143236, -2.2305099474271075, -3.0825279994876054, -2.7221139559921075, -2.2879942198598555, -2.2799142642563752, -2.329886263223439, -2.866026754226455, -1.9461390141893085, -1.985090723006627, -2.4746848803154777, -2.081687611184221, -2.074101633149943, -2.9959906191736447, -2.9885348741351585, -2.981142583015231, -2.195667852445213, -1.8784224796673736, -2.1811910345973744, -2.0918569646751717, -2.166951552351479, -2.393998396957847, -2.152941749214162, -2.924165507392356, -2.917299155715568, -2.3664218279865805, -2.903727177028984, -2.2949534736042683, -2.4510264914334274, -1.9543494514454665, -1.9477940319229945, -1.9412877171275509, -1.7339213619301692, -2.505647869781213, -2.851465463314668, -2.168459636198889, -3.4409353814357813, -2.0545057038737986, -1.7383467464518634, -1.8909206250910533, -1.9539045510945445, -1.677863914729682, -1.7140489672926733, -2.620106412974031, -2.1882055087215893, -2.60828869375299, -3.380592445119423, -1.9945792571189123, -1.9888078806439358, -1.9830745993407295, -2.4033428248864506, -1.7956097902569303, -2.0240758627641036, -2.194592570573394, -2.0129399542862187, -2.007425085195841, -2.045423560360459, -1.7872573485453167, -2.0345660569376625, -2.70587656854222, -2.023842600193446, -1.7062255347473776, -1.559621010492369, -2.008001632921252, -2.0027848667061954, -1.6329082048952646, -1.6277533591196431, -1.6750153880862255, -1.6699210100584658, -1.4850753602319753, -1.5184966926625907, -1.654814734277574, -1.9621417116287732, -2.2817003508933484, -1.9522712762777488, -1.5826867637292024, -1.6302071688829871, -2.438267114336293, -2.433454974804536, -2.4286693485727553, -1.5892660894575017, -1.4897430893851515, -1.7776401420205528, -1.9091919205655294, -1.6518141007841682, -2.2244099879942882, -2.2198020781751597, -2.023334565376659, -2.210658952026193, -2.014239309875218, -2.553791979611934, -2.373208664682453, -2.368742901817869, -1.6510815032030195, -1.5817187796066705, -2.5315762171044196, -3.129258829124558, -1.9787817759543547, -1.6581845111836904, -3.116262243050724, -2.509914521801056, -1.6453162911728705, -1.512405508731265, -1.719027334491968, -1.8162771180875266, -1.7106351053047515, -1.9405491950602092, -1.8037792195335236, -1.546932403261781, -1.6119049041671651, -3.070205775066496, -2.2879845778445236, -1.7398623392734758, -2.016661580443094, -1.5916571583276091, -2.095812699312438, -2.444018367947245, -2.440061235983069, -1.6579772278600535, -1.6540558263289973, -1.5679668999283467, -1.4950012771888406, -1.560211589801943, -1.6385448969354728, -2.2367604101566596, -1.3483229928906202, -1.2997077707244487, -2.2253564525077194, -1.7209938492170735, -1.464521344075367, -1.846129925230279, -2.0342939717013624, -1.604626050686802, -1.3377027624067772, -1.2872882797424154, -1.4423433997441422, -1.5899659733339992, -2.188389641119693, -2.360872512477745, -1.5791310432694121, -1.5755492280336503, -1.4207176611797074, -1.486244457295603, -1.5648915610235166, -2.3395126911081503, -1.4756732643722354, -1.095739694634786, -1.1987088815761062, -1.5474143322681984, -2.3221055160643935, -2.318665555275846, -1.5370943419903984, -1.223704610894713, -1.3790173832334671, -1.628351562338773, -1.3722579019307057, -1.858969554582452, -1.4820369028849445, -2.29162558295092, -1.686237595578451, -2.284995100647966, -1.6050099552616999, -1.6763484303443261, -2.877201708681837, -2.2718840748983316, -1.7245721792247393, -1.588713248996546, -1.8228415544269811, -1.9067871047728366, -1.5790800009329646, -2.854639687862459, -1.6473390525771658, -1.8069036950844306, -2.0669939604124696, -2.8420054438150744, -inf, -inf, -inf]] caption="Water Vapor Number Density"
  out "raw counts":dbl[][](graph)=[[938.9, 988.9, 893.9, 948.9, 1280.9, 1253.9, 768.9, 422.9, 790.9, 1860.9, 2621.9, 3373.9, 3379.9, 2714.9, 2161.9, 2108.9, 2465.9, 2701.9, 2847.9, 3401.9, 4152.9, 3506.9, 2075.9, 750.9, 260.9, 311.9, 222.9, 193.9, 230.9, 338.9, 459.9, 509.9, 544.9, 730.9, 1192.9, 1254.9, 840.9, 406.9, 343.9, 247.9, 82.9, 17.9, 3.9000000000000004, 2.9000000000000004, -0.09999999999999964, -1.0999999999999996, -1.0999999999999996, -2.0999999999999996, -3.0999999999999996, -3.0999999999999996, -2.0999999999999996, -0.09999999999999964, 3.9000000000000004, -1.0999999999999996, 0.9000000000000004, -1.0999999999999996, 1.9000000000000004, -3.0999999999999996, 2.9000000000000004, -1.0999999999999996, 2.9000000000000004, -2.0999999999999996, -0.09999999999999964, -0.09999999999999964, 3.9000000000000004, 1.9000000000000004, -1.0999999999999996, 0.9000000000000004, 1.9000000000000004, -0.09999999999999964, -0.09999999999999964, -2.0999999999999996, -1.0999999999999996, -0.09999999999999964, -1.0999999999999996, -0.09999999999999964, 2.9000000000000004, -0.09999999999999964, 3.9000000000000004, 1.9000000000000004, -0.09999999999999964, -0.09999999999999964, -0.09999999999999964, -0.09999999999999964, 0.9000000000000004, -1.0999999999999996, -0.09999999999999964, -0.09999999999999964, -2.0999999999999996, -0.09999999999999964, -1.0999999999999996, -0.09999999999999964, -5.1, -2.0999999999999996, -2.0999999999999996, 1.9000000000000004, -1.0999999999999996, -3.0999999999999996, -1.0999999999999996, -1.0999999999999996, -0.09999999999999964, -3.0999999999999996, 2.9000000000000004, -2.0999999999999996, -1.0999999999999996, -4.1, -4.1, -1.0999999999999996, -1.0999999999999996, 1.9000000000000004, -4.1, -3.0999999999999996, 2.9000000000000004, -1.0999999999999996, -1.0999999999999996, -3.0999999999999996, -3.0999999999999996, -2.0999999999999996, -2.0999999999999996, -3.0999999999999996, -4.1, 1.9000000000000004, -5.1, 0.9000000000000004, 0.9000000000000004, -1.0999999999999996, -1.0999999999999996, -3.0999999999999996, 0.9000000000000004, -1.0999999999999996, -3.0999999999999996, -5.1, 6.9, 1.9000000000000004, 6.9, -2.0999999999999996, 0.9000000000000004, -0.09999999999999964, -3.0999999999999996, -1.0999999999999996, -2.0999999999999996, -3.0999999999999996, 1.9000000000000004, -4.1, -2.0999999999999996, -2.0999999999999996, 1.9000000000000004, -2.0999999999999996, -3.0999999999999996, -2.0999999999999996, -3.0999999999999996, -4.1, -2.0999999999999996, -1.0999999999999996, -1.0999999999999996, -4.1, -1.0999999999999996, -2.0999999999999996, -0.09999999999999964, -1.0999999999999996, -1.0999999999999996, 1.9000000000000004, -0.09999999999999964, -2.0999999999999996, -0.09999999999999964, -1.0999999999999996, -3.0999999999999996, -2.0999999999999996, -4.1, 0.9000000000000004, -3.0999999999999996, -3.0999999999999996, -2.0999999999999996, -2.0999999999999996, -1.0999999999999996, -2.0999999999999996, 1.9000000000000004, 0.9000000000000004, 2.9000000000000004, -1.0999999999999996, -2.0999999999999996, -4.1, -1.0999999999999996, 1.9000000000000004, 0.9000000000000004, -2.0999999999999996, -1.0999999999999996, -1.0999999999999996, -3.0999999999999996, -1.0999999999999996, 0.9000000000000004, -0.09999999999999964, -0.09999999999999964, 0.9000000000000004, -3.0999999999999996, -2.0999999999999996, -1.0999999999999996, -1.0999999999999996, -4.1, -1.0999999999999996, -1.0999999999999996, -0.09999999999999964, -0.09999999999999964, -2.0999999999999996, -3.0999999999999996, -2.0999999999999996, -0.09999999999999964, -2.0999999999999996, -1.0999999999999996, -2.0999999999999996, -2.0999999999999996, 0.9000000000000004, -2.0999999999999996, -0.09999999999999964, -0.09999999999999964, 0.9000000000000004, -3.0999999999999996, 0.9000000000000004, -1.0999999999999996, -4.1, -2.0999999999999996, -0.09999999999999964, -4.1, -5.1, -2.0999999999999996, -5.1, 0.9000000000000004, -3.0999999999999996, -1.0999999999999996, 0.9000000000000004, 1.9000000000000004, -1.0999999999999996, 2.9000000000000004, -3.0999999999999996, -1.0999999999999996, -1.0999999999999996, -3.0999999999999996, -3.0999999999999996, 2.9000000000000004, -3.0999999999999996, -0.09999999999999964, -1.0999999999999996, -4.1, -0.09999999999999964, -4.1, -0.09999999999999964, -0.09999999999999964, -0.09999999999999964, 0.9000000000000004, -0.09999999999999964, -0.09999999999999964, 0.9000000000000004, -2.0999999999999996, -2.0999999999999996, 4.9, -4.1, -4.1, -1.0999999999999996, -1.0999999999999996, -2.0999999999999996, -0.09999999999999964, -4.1, -2.0999999999999996, -0.09999999999999964, -2.0999999999999996, -0.09999999999999964, 2.9000000000000004, -0.09999999999999964, 0.9000000000000004, -3.0999999999999996, -2.0999999999999996, 2.9000000000000004, -1.0999999999999996, -3.0999999999999996, 2.9000000000000004, -1.0999999999999996, 3.9000000000000004, 1.9000000000000004, -1.0999999999999996, 0.0]] caption="Water Vapor Number Density"
  out "raw counts near":dbl[][](graph)=[[2382.6, 2697.6, 2843.6, 3137.6, 4025.6, 3802.6, 2176.6, 1092.6, 1987.6, 4591.6, 6038.6, 6777.6, 6483.6, 4982.6, 3675.6, 3236.6, 3392.6, 3540.6, 3398.6, 3986.6, 4735.6, 3674.6, 2084.6, 721.6, 292.6, 285.6, 230.6, 173.6, 221.6, 330.6, 441.6, 457.6, 447.6, 631.6, 1010.6, 1159.6, 685.6, 426.6, 321.6, 204.6, 70.6, 20.6, 8.6, 1.5999999999999996, -4.4, -2.4000000000000004, 5.6, -2.4000000000000004, 4.6, -7.4, -0.40000000000000036, -5.4, 3.5999999999999996, -5.4, -7.4, -0.40000000000000036, 0.5999999999999996, -1.4000000000000004, 1.5999999999999996, -1.4000000000000004, -4.4, -0.40000000000000036, -3.4000000000000004, -3.4000000000000004, -4.4, -3.4000000000000004, 4.6, 1.5999999999999996, -2.4000000000000004, 1.5999999999999996, 1.5999999999999996, 4.6, 1.5999999999999996, 1.5999999999999996, 2.5999999999999996, -3.4000000000000004, -0.40000000000000036, -0.40000000000000036, -7.4, -3.4000000000000004, -0.40000000000000036, 4.6, -4.4, 0.5999999999999996, -1.4000000000000004, -3.4000000000000004, 0.5999999999999996, -2.4000000000000004, 3.5999999999999996, 0.5999999999999996, 2.5999999999999996, -3.4000000000000004, 3.5999999999999996, -5.4, 2.5999999999999996, 1.5999999999999996, -4.4, -4.4, 2.5999999999999996, 1.5999999999999996, 2.5999999999999996, 1.5999999999999996, 1.5999999999999996, -7.4, 1.5999999999999996, -2.4000000000000004, 0.5999999999999996, -5.4, 0.5999999999999996, 3.5999999999999996, -2.4000000000000004, -7.4, -1.4000000000000004, -1.4000000000000004, -5.4, -1.4000000000000004, 0.5999999999999996, -1.4000000000000004, 0.5999999999999996, -5.4, -4.4, -0.40000000000000036, -5.4, 0.5999999999999996, -3.4000000000000004, -1.4000000000000004, 0.5999999999999996, -1.4000000000000004, -1.4000000000000004, 0.5999999999999996, 2.5999999999999996, -0.40000000000000036, -6.4, -0.40000000000000036, -6.4, -4.4, 2.5999999999999996, -3.4000000000000004, -0.40000000000000036, 0.5999999999999996, -5.4, -4.4, -2.4000000000000004, -3.4000000000000004, -7.4, -2.4000000000000004, 3.5999999999999996, -0.40000000000000036, 1.5999999999999996, -1.4000000000000004, -3.4000000000000004, -1.4000000000000004, -3.4000000000000004, 1.5999999999999996, 5.6, -1.4000000000000004, -1.4000000000000004, 5.6, -1.4000000000000004, -2.4000000000000004, -4.4, 0.5999999999999996, -1.4000000000000004, -2.4000000000000004, -5.4, -5.4, 1.5999999999999996, -5.4, -3.4000000000000004, -5.4, -2.4000000000000004, -5.4, -6.4, -4.4, -3.4000000000000004, -0.40000000000000036, -1.4000000000000004, -2.4000000000000004, -6.4, -1.4000000000000004, 2.5999999999999996, -1.4000000000000004, 2.5999999999999996, 5.6, 4.6, 0.5999999999999996, -4.4, -2.4000000000000004, 0.5999999999999996, -2.4000000000000004, -0.40000000000000036, -1.4000000000000004, -1.4000000000000004, 0.5999999999999996, 0.5999999999999996, 0.5999999999999996, 5.6, 1.5999999999999996, -2.4000000000000004, 2.5999999999999996, -5.4, -0.40000000000000036, 0.5999999999999996, -1.4000000000000004, -4.4, -3.4000000000000004, -1.4000000000000004, -2.4000000000000004, -2.4000000000000004, -0.40000000000000036, -3.4000000000000004, -3.4000000000000004, -2.4000000000000004, 2.5999999999999996, -1.4000000000000004, 5.6, -3.4000000000000004, -2.4000000000000004, 0.5999999999999996, -1.4000000000000004, 0.5999999999999996, -5.4, 0.5999999999999996, -6.4, -0.40000000000000036, -5.4, 0.5999999999999996, 0.5999999999999996, 8.6, 1.5999999999999996, -0.40000000000000036, -3.4000000000000004, -3.4000000000000004, 0.5999999999999996, -2.4000000000000004, -2.4000000000000004, -6.4, -3.4000000000000004, -3.4000000000000004, -1.4000000000000004, 2.5999999999999996, -3.4000000000000004, -1.4000000000000004, -3.4000000000000004, -3.4000000000000004, -2.4000000000000004, -2.4000000000000004, 1.5999999999999996, -7.4, -6.4, -4.4, -0.40000000000000036, -0.40000000000000036, -0.40000000000000036, -4.4, -5.4, -1.4000000000000004, -2.4000000000000004, -4.4, 6.6, -1.4000000000000004, 0.5999999999999996, 2.5999999999999996, -3.4000000000000004, -0.40000000000000036, 3.5999999999999996, -3.4000000000000004, 2.5999999999999996, -5.4, 1.5999999999999996, 0.5999999999999996, -2.4000000000000004, -1.4000000000000004, 1.5999999999999996, 1.5999999999999996, 0.5999999999999996, 0.5999999999999996, -0.40000000000000036, -2.4000000000000004, 0.0]] caption="Water Vapor Number Density"
  out "Aerosol Smoothed 2":dbl[](array[numeric])=[2540.1, 2770.6, 2990.6, 3581.6, 3914.1, 2989.6, 1634.6, 1540.1, 3289.6000000000004, 5315.1, 6408.1, 6630.6, 5733.1, 4329.1, 3456.1, 3314.6, 3466.6, 3469.6, 3692.6, 4361.1, 4205.1, 2879.6, 1403.1, 507.1, 289.1, 258.1, 202.1, 197.6, 276.1, 386.1, 449.6, 452.6, 539.6, 821.1, 1085.1, 922.5999999999999, 556.1, 374.1, 263.1, 137.6, 45.599999999999994, 14.600000000000001, 5.1, -1.4000000000000004, -3.4000000000000004, 1.5999999999999996, 1.5999999999999996, 1.0999999999999996, -1.4000000000000004, -3.9000000000000004, -2.9000000000000004, -0.9000000000000004, -0.9000000000000004, -6.4, -3.9000000000000004, 0.09999999999999964, -0.40000000000000036, 0.09999999999999964, 0.09999999999999964, -2.9000000000000004, -2.4000000000000004, -1.9000000000000004, -3.4000000000000004, -3.9000000000000004, -3.9000000000000004, 0.5999999999999996, 3.0999999999999996, -0.40000000000000036, -0.40000000000000036, 1.5999999999999996, 3.0999999999999996, 3.0999999999999996, 1.5999999999999996, 2.0999999999999996, -0.40000000000000036, -1.9000000000000004, -0.40000000000000036, -3.9000000000000004, -5.4, -1.9000000000000004, 2.0999999999999996, 0.09999999999999964, -1.9000000000000004, -0.40000000000000036, -2.4000000000000004, -1.4000000000000004, -0.9000000000000004, 0.5999999999999996, 2.0999999999999996, 1.5999999999999996, -0.40000000000000036, 0.09999999999999964, -0.9000000000000004, -1.4000000000000004, 2.0999999999999996, -1.4000000000000004, -4.4, -0.9000000000000004, 2.0999999999999996, 2.0999999999999996, 2.0999999999999996, 1.5999999999999996, -2.9000000000000004, -2.9000000000000004, -0.40000000000000036, -0.9000000000000004, -2.4000000000000004, -2.4000000000000004, 2.0999999999999996, 0.5999999999999996, -4.9, -4.4, -1.4000000000000004, -3.4000000000000004, -3.4000000000000004, -0.40000000000000036, -0.40000000000000036, -0.40000000000000036, -2.4000000000000004, -4.9, -2.4000000000000004, -2.9000000000000004, -2.4000000000000004, -1.4000000000000004, -2.4000000000000004, -0.40000000000000036, -0.40000000000000036, -1.4000000000000004, -0.40000000000000036, 1.5999999999999996, 1.0999999999999996, -3.4000000000000004, -3.4000000000000004, -3.4000000000000004, -5.4, -0.9000000000000004, -0.40000000000000036, -1.9000000000000004, 0.09999999999999964, -2.4000000000000004, -4.9, -3.4000000000000004, -2.9000000000000004, -5.4, -4.9, 0.5999999999999996, 1.5999999999999996, 0.5999999999999996, 0.09999999999999964, -2.4000000000000004, -2.4000000000000004, -2.4000000000000004, -0.9000000000000004, 3.5999999999999996, 2.0999999999999996, -1.4000000000000004, 2.0999999999999996, 2.0999999999999996, -1.9000000000000004, -3.4000000000000004, -1.9000000000000004, -0.40000000000000036, -1.9000000000000004, -3.9000000000000004, -5.4, -1.9000000000000004, -1.9000000000000004, -4.4, -4.4, -3.9000000000000004, -3.9000000000000004, -5.9, -5.4, -3.9000000000000004, -1.9000000000000004, -0.9000000000000004, -1.9000000000000004, -4.4, -3.9000000000000004, 0.5999999999999996, 0.5999999999999996, 0.5999999999999996, 4.1, 5.1, 2.5999999999999996, -1.9000000000000004, -3.4000000000000004, -0.9000000000000004, -0.9000000000000004, -1.4000000000000004, -0.9000000000000004, -1.4000000000000004, -0.40000000000000036, 0.5999999999999996, 0.5999999999999996, 3.0999999999999996, 3.5999999999999996, -0.40000000000000036, 0.09999999999999964, -1.4000000000000004, -2.9000000000000004, 0.09999999999999964, -0.40000000000000036, -2.9000000000000004, -3.9000000000000004, -2.4000000000000004, -1.9000000000000004, -2.4000000000000004, -1.4000000000000004, -1.9000000000000004, -3.4000000000000004, -2.9000000000000004, 0.09999999999999964, 0.5999999999999996, 2.0999999999999996, 1.0999999999999996, -2.9000000000000004, -0.9000000000000004, -0.40000000000000036, -0.40000000000000036, -2.4000000000000004, -2.4000000000000004, -2.9000000000000004, -3.4000000000000004, -2.9000000000000004, -2.4000000000000004, 0.5999999999999996, 4.6, 5.1, 0.5999999999999996, -1.9000000000000004, -3.4000000000000004, -1.4000000000000004, -0.9000000000000004, -2.4000000000000004, -4.4, -4.9, -3.4000000000000004, -2.4000000000000004, 0.5999999999999996, -0.40000000000000036, -2.4000000000000004, -2.4000000000000004, -3.4000000000000004, -2.9000000000000004, -2.4000000000000004, -0.40000000000000036, -2.9000000000000004, -6.9, -5.4, -2.4000000000000004, -0.40000000000000036, -0.40000000000000036, -2.4000000000000004, -4.9, -3.4000000000000004, -1.9000000000000004, -3.4000000000000004, 1.0999999999999996, 2.5999999999999996, -0.40000000000000036, 1.5999999999999996, -0.40000000000000036, -1.9000000000000004, 1.5999999999999996, 0.09999999999999964, -0.40000000000000036, -1.4000000000000004, -1.9000000000000004, 1.0999999999999996, -0.9000000000000004, -1.9000000000000004, 0.09999999999999964, 1.5999999999999996, 1.0999999999999996, 0.5999999999999996, 0.09999999999999964]
  out "Off-Line Smoothed 2":dbl[](array[numeric])=[6642.953333333331, 7228.019999999998, 7339.608888888886, 7089.514444444441, 6398.381111111108, 5253.139444444443, 3894.411666666667, 2911.494999999999, 2933.2811111111105, 3901.0616666666656, 5074.786666666665, 5809.342222222221, 5938.936666666665, 5586.6144444444435, 5004.508888888889, 4612.261666666666, 4977.111666666666, 4922.853333333333, 3451.5227777777773, 2216.1477777777773, 2130.80611111111, 2460.892222222222, 2628.7727777777773, 2529.475555555555, 2239.281111111111, 1805.0311111111118, 1273.0061111111113, 816.5283333333334, 520.2616666666665, 328.20333333333326, 199.7283333333333, 129.0005555555555, 101.57277777777777, 94.63944444444444, 87.93666666666667, 68.51166666666668, 43.57833333333335, 25.708888888888886, 15.475555555555554, 9.395, 5.867222222222222, 3.897777777777778, 2.772777777777778, 2.4061111111111115, 2.603333333333334, 2.5227777777777787, 2.2394444444444455, 2.347777777777778, 2.3505555555555557, 2.161666666666667, 2.203333333333334, 2.195000000000001, 2.170000000000001, 2.183888888888889, 1.9450000000000003, 1.8172222222222225, 1.9088888888888893, 1.831111111111111, 1.6561111111111104, 1.703333333333333, 1.567222222222222, 1.478333333333333, 1.5894444444444438, 1.5561111111111103, 1.5422222222222213, 1.7199999999999998, 1.758888888888889, 1.5838888888888882, 1.5172222222222216, 1.7116666666666667, 1.8950000000000002, 1.7227777777777775, 1.5199999999999996, 1.300555555555555, 1.1366666666666663, 1.0255555555555558, 1.0283333333333335, 1.0866666666666667, 1.3644444444444441, 1.2505555555555552, 0.9700000000000002, 0.972777777777778, 1.02, 1.2477777777777777, 1.133888888888889, 1.1033333333333333, 1.2477777777777774, 1.2644444444444443, 1.1227777777777779, 1.045, 1.1672222222222222, 1.1561111111111109, 0.8033333333333331, 0.7172222222222222, 1.031111111111111, 0.8783333333333333, 0.8477777777777776, 0.9116666666666666, 0.8338888888888889, 1.0144444444444443, 0.9422222222222223, 0.856111111111111, 0.7144444444444444, 0.6727777777777778, 0.9866666666666666, 0.9838888888888888, 0.9088888888888889, 0.8366666666666667, 0.645, 0.5755555555555555, 0.7616666666666667, 0.9422222222222221, 0.5255555555555554, 0.3505555555555556, 0.5838888888888889, 0.6255555555555554, 0.4616666666666666, 0.3005555555555556, 0.5783333333333334, 0.7699999999999998, 0.6533333333333331, 0.38111111111111107, 0.35333333333333333, 0.5977777777777777, 0.3977777777777778, 0.5533333333333336, 0.8588888888888888, 0.7283333333333333, 0.7477777777777779, 1.0116666666666665, 0.9866666666666666, 0.7144444444444444, 0.6422222222222222, 0.6144444444444445, 0.6088888888888887, 0.72, 0.7255555555555557, 0.3977777777777779, 0.31166666666666687, 0.34500000000000014, 0.41999999999999993, 0.6199999999999998, 0.642222222222222, 0.4255555555555555, 0.345, 0.48111111111111093, 0.21444444444444433, 0.34222222222222254, 0.7866666666666668, 0.5116666666666667, 0.31166666666666676, 0.33944444444444444, 0.48111111111111116, 0.6033333333333334, 0.5727777777777778, 0.6088888888888888, 0.3005555555555555, 0.26166666666666655, 0.39222222222222203, 0.2977777777777778, 0.39222222222222225, 0.40888888888888897, 0.21166666666666673, 0.2672222222222222, 0.4838888888888887, 0.4644444444444442, 0.5949999999999999, 0.642222222222222, 0.6588888888888886, 0.8144444444444445, 0.5200000000000001, 0.4505555555555554, 0.43111111111111095, 0.21444444444444438, 0.5477777777777777, 0.7116666666666664, 0.4227777777777776, 0.41999999999999993, 0.6727777777777775, 0.5338888888888886, 0.195, 0.18388888888888896, 0.4755555555555556, 0.5311111111111112, 0.3283333333333334, 0.22000000000000008, 0.07000000000000005, 0.15333333333333335, 0.21999999999999997, 0.07277777777777776, 0.19777777777777764, 0.3505555555555553, 0.3088888888888889, 0.18666666666666676, 0.10888888888888894, 0.29500000000000004, 0.3894444444444446, 0.07833333333333345, 0.050555555555555645, 0.14222222222222244, 0.197777777777778, 0.3394444444444445, 0.04777777777777778, -0.22722222222222216, 0.195, 0.43388888888888877, 0.2144444444444444, 0.28666666666666657, 0.19222222222222216, -0.0716666666666666, -0.07722222222222218, 0.05611111111111114, 0.31166666666666665, 0.5422222222222219, 0.35611111111111093, 0.22555555555555556, 0.3227777777777777, 0.26999999999999996, 0.12000000000000008, -0.09666666666666655, -0.14388888888888884, 0.27555555555555544, 0.38666666666666655, 0.04499999999999997, 0.12000000000000009, 0.08388888888888901, -0.24388888888888877, -0.1744444444444442, 0.2672222222222224, 0.2450000000000001, -0.10499999999999994, -0.11055555555555555, -0.06333333333333344, -0.0327777777777779, 0.036666666666666695, 0.07277777777777786, 0.0894444444444445, -0.03555555555555554, -0.060555555555555536, 0.06999999999999997, 0.12833333333333347, 0.09500000000000022, 0.06722222222222235, 0.10611111111111127, 0.23111111111111116, 0.3727777777777777, -0.08000000000000018, -0.2550000000000001, -0.05500000000000001, -0.0772222222222223, -0.016111111111111128, -0.22444444444444442, 0.056111111111110945, 0.4144444444444443, 0.14222222222222233, -0.02722222222222218, 0.18666666666666676, 0.1283333333333334, 0.13111111111111115, 0.14500000000000007, 0.1255555555555555, 0.23388888888888887, 0.25888888888888906, 0.2505555555555557, 0.21166666666666678, 0.14500000000000007, -0.018888888888888903, -0.02999999999999998, 0.056111111111111174, 0.031111111111111173, -0.10222222222222213, 0.0644444444444445, 0.15333333333333332, -0.06611111111111104, -0.11888888888888881, -0.035555555555555465, 0.07555555555555565]
  out "Off-Line Bin Readings 2":dbl[](array[numeric])=[2393.0, 2708.0, 2854.0, 3148.0, 4036.0, 3813.0, 2187.0, 1103.0, 1998.0, 4602.0, 6049.0, 6788.0, 6494.0, 4993.0, 3686.0, 3247.0, 3403.0, 3551.0, 3409.0, 3997.0, 4746.0, 3685.0, 2095.0, 732.0, 303.0, 296.0, 241.0, 184.0, 232.0, 341.0, 452.0, 468.0, 458.0, 642.0, 1021.0, 1170.0, 696.0, 437.0, 332.0, 215.0, 81.0, 31.0, 19.0, 12.0, 6.0, 8.0, 16.0, 8.0, 15.0, 3.0, 10.0, 5.0, 14.0, 5.0, 3.0, 10.0, 11.0, 9.0, 12.0, 9.0, 6.0, 10.0, 7.0, 7.0, 6.0, 7.0, 15.0, 12.0, 8.0, 12.0, 12.0, 15.0, 12.0, 12.0, 13.0, 7.0, 10.0, 10.0, 3.0, 7.0, 10.0, 15.0, 6.0, 11.0, 9.0, 7.0, 11.0, 8.0, 14.0, 11.0, 13.0, 7.0, 14.0, 5.0, 13.0, 12.0, 6.0, 6.0, 13.0, 12.0, 13.0, 12.0, 12.0, 3.0, 12.0, 8.0, 11.0, 5.0, 11.0, 14.0, 8.0, 3.0, 9.0, 9.0, 5.0, 9.0, 11.0, 9.0, 11.0, 5.0, 6.0, 10.0, 5.0, 11.0, 7.0, 9.0, 11.0, 9.0, 9.0, 11.0, 13.0, 10.0, 4.0, 10.0, 4.0, 6.0, 13.0, 7.0, 10.0, 11.0, 5.0, 6.0, 8.0, 7.0, 3.0, 8.0, 14.0, 10.0, 12.0, 9.0, 7.0, 9.0, 7.0, 12.0, 16.0, 9.0, 9.0, 16.0, 9.0, 8.0, 6.0, 11.0, 9.0, 8.0, 5.0, 5.0, 12.0, 5.0, 7.0, 5.0, 8.0, 5.0, 4.0, 6.0, 7.0, 10.0, 9.0, 8.0, 4.0, 9.0, 13.0, 9.0, 13.0, 16.0, 15.0, 11.0, 6.0, 8.0, 11.0, 8.0, 10.0, 9.0, 9.0, 11.0, 11.0, 11.0, 16.0, 12.0, 8.0, 13.0, 5.0, 10.0, 11.0, 9.0, 6.0, 7.0, 9.0, 8.0, 8.0, 10.0, 7.0, 7.0, 8.0, 13.0, 9.0, 16.0, 7.0, 8.0, 11.0, 9.0, 11.0, 5.0, 11.0, 4.0, 10.0, 5.0, 11.0, 11.0, 19.0, 12.0, 10.0, 7.0, 7.0, 11.0, 8.0, 8.0, 4.0, 7.0, 7.0, 9.0, 13.0, 7.0, 9.0, 7.0, 7.0, 8.0, 8.0, 12.0, 3.0, 4.0, 6.0, 10.0, 10.0, 10.0, 6.0, 5.0, 9.0, 8.0, 6.0, 17.0, 9.0, 11.0, 13.0, 7.0, 10.0, 14.0, 7.0, 13.0, 5.0, 12.0, 11.0, 8.0, 9.0, 12.0, 12.0, 11.0, 11.0, 10.0, 8.0]
  out "On-Line Smoothed 2":dbl[](array[numeric])=[5750.5722222222175, 5773.50833333333, 5415.672222222218, 4835.991666666663, 4031.011111111109, 3048.069444444444, 2086.1555555555556, 1437.2027777777785, 1325.5777777777787, 1647.866666666667, 2018.8916666666664, 2171.386111111111, 2085.072222222222, 1839.127777777778, 1540.4638888888896, 1339.6444444444455, 1364.2777777777787, 1287.0361111111122, 854.2583333333339, 500.14722222222224, 451.875, 499.2500000000001, 515.0250000000001, 480.05, 408.5194444444444, 316.24166666666656, 214.54166666666666, 132.8888888888889, 81.30555555555557, 49.2888888888889, 29.96388888888888, 19.341666666666654, 14.927777777777766, 14.019444444444437, 12.949999999999994, 10.083333333333332, 6.833333333333335, 4.638888888888891, 3.2555555555555564, 2.808333333333333, 2.388888888888889, 1.683333333333333, 1.6777777777777771, 1.85, 1.8472222222222223, 1.8611111111111112, 1.7944444444444443, 1.8166666666666664, 1.8194444444444444, 1.5472222222222218, 1.3916666666666662, 1.4166666666666659, 1.4083333333333323, 1.4611111111111104, 1.4166666666666659, 1.552777777777777, 1.6055555555555547, 1.533333333333333, 1.3944444444444442, 1.2138888888888881, 1.3222222222222215, 1.4333333333333327, 1.7249999999999996, 1.5999999999999992, 1.3027777777777771, 1.3083333333333327, 1.3083333333333325, 1.4083333333333328, 1.3027777777777771, 1.2444444444444436, 0.9944444444444439, 0.9749999999999995, 1.1583333333333323, 1.1361111111111102, 1.174999999999999, 1.0833333333333326, 0.9472222222222215, 1.0083333333333326, 1.0583333333333327, 0.8388888888888886, 0.9888888888888884, 0.994444444444444, 0.7777777777777777, 0.5499999999999999, 0.608333333333333, 0.8944444444444437, 1.0222222222222213, 1.1277777777777767, 1.0694444444444438, 0.9499999999999993, 0.9249999999999994, 1.0472222222222212, 0.7222222222222215, 0.5166666666666665, 0.5972222222222221, 0.6333333333333331, 0.6833333333333329, 0.5333333333333332, 0.5999999999999998, 0.708333333333333, 0.5527777777777777, 0.5722222222222222, 0.6999999999999997, 0.708333333333333, 0.6111111111111109, 0.5111111111111111, 0.561111111111111, 0.40555555555555556, 0.48333333333333295, 0.6027777777777773, 0.5083333333333333, 0.7194444444444443, 0.8249999999999995, 0.49722222222222195, 0.39166666666666666, 0.7472222222222218, 0.9055555555555548, 0.7638888888888886, 0.5861111111111108, 0.42222222222222194, 0.3944444444444445, 0.5888888888888887, 0.39722222222222203, 0.26666666666666666, 0.35000000000000003, 0.3055555555555556, 0.4416666666666666, 0.6388888888888885, 0.5777777777777773, 0.3138888888888888, 0.32500000000000007, 0.22499999999999998, 0.3222222222222222, 0.5305555555555557, 0.4805555555555555, 0.5527777777777776, 0.5444444444444444, 0.4666666666666667, 0.5333333333333331, 0.5055555555555553, 0.32222222222222224, 0.5333333333333332, 0.6027777777777776, 0.19722222222222222, 0.30277777777777776, 0.55, 0.31666666666666665, 0.2777777777777778, 0.18611111111111114, 0.07500000000000004, 0.26111111111111107, 0.15277777777777773, 0.2, 0.5166666666666665, 0.547222222222222, 0.4194444444444445, 0.10833333333333343, 0.1916666666666666, 0.2138888888888888, 0.15277777777777762, 0.4194444444444443, 0.33888888888888874, 0.22499999999999995, 0.18611111111111106, 0.1861111111111111, 0.31388888888888883, 0.3583333333333333, 0.2027777777777779, 0.09166666666666665, 0.26388888888888873, 0.10833333333333327, 0.2499999999999999, 0.5249999999999999, 0.12777777777777774, 0.17222222222222214, 0.2694444444444444, 0.23055555555555557, 0.26111111111111107, 0.2944444444444444, 0.3861111111111112, 0.33611111111111125, 0.27222222222222237, 0.15000000000000002, 0.02777777777777772, 0.308333333333333, 0.39444444444444415, 0.22222222222222227, 0.2444444444444444, 0.20833333333333326, 0.3555555555555555, 0.4472222222222222, 0.24444444444444433, 0.08333333333333322, 0.1305555555555555, 0.3333333333333333, 0.25, 0.17222222222222228, 0.00833333333333336, -0.15555555555555559, 0.07222222222222215, 0.12222222222222212, 0.022222222222222154, 0.01111111111111104, 0.2555555555555554, 0.20277777777777767, 0.027777777777777762, -0.016666666666666663, 0.008333333333333331, 0.03888888888888886, -0.11111111111111108, -0.19722222222222224, -0.011111111111111072, -0.08055555555555545, -0.37500000000000006, 0.0749999999999999, 0.2638888888888889, 0.0666666666666667, 0.033333333333333326, 0.15000000000000002, 0.363888888888889, 0.016666666666666774, -0.04444444444444423, 0.13888888888888903, 0.011111111111111132, -0.036111111111111205, 0.055555555555555566, 0.09166666666666667, 0.13055555555555556, 0.3055555555555556, 0.1472222222222221, 0.011111111111111058, 0.17777777777777792, 0.127777777777778, 0.1583333333333334, 0.10000000000000012, 0.06944444444444449, 0.2194444444444444, 0.3055555555555555, 0.2666666666666666, -0.0333333333333334, 0.14444444444444435, 0.37777777777777777, 0.21111111111111114, 0.30555555555555547, 0.3111111111111111, 0.027777777777777804, -0.11944444444444446, -0.08611111111111111, 0.16388888888888897, 0.23055555555555557, -0.08333333333333336, -0.36944444444444446, -0.063888888888889, 0.09999999999999988, -0.06666666666666676, 0.15833333333333324, -0.08055555555555563, -0.18055555555555564, 0.0805555555555555, 0.03055555555555551, -0.022222222222222303, 0.08888888888888881, 0.14444444444444443, -0.08333333333333327, -0.1833333333333334, -0.10277777777777797, 0.10277777777777763, 0.1638888888888888, 0.15555555555555556, 0.0722222222222222, -0.030555555555555645, -0.20833333333333337, -0.20277777777777778, 0.13055555555555554, 0.16388888888888892, 0.0944444444444445, 0.047222222222222214]
  out "On-Line Bin Readings 2":dbl[](array[numeric])=[2197.0, 2381.0, 2188.0, 2206.0, 2771.0, 2358.0, 1249.0, 550.0, 874.0, 2028.0, 2484.0, 2652.0, 2322.0, 1734.0, 1156.0, 1007.0, 938.0, 927.0, 870.0, 893.0, 1014.0, 799.0, 418.0, 157.0, 52.0, 55.0, 48.0, 39.0, 57.0, 64.0, 73.0, 64.0, 72.0, 87.0, 126.0, 137.0, 89.0, 49.0, 40.0, 40.0, 13.0, 10.0, 7.0, 8.0, 11.0, 11.0, 7.0, 14.0, 9.0, 11.0, 13.0, 11.0, 9.0, 10.0, 13.0, 12.0, 10.0, 5.0, 20.0, 7.0, 6.0, 8.0, 7.0, 10.0, 13.0, 7.0, 13.0, 7.0, 8.0, 11.0, 16.0, 9.0, 5.0, 7.0, 8.0, 4.0, 12.0, 4.0, 12.0, 14.0, 9.0, 6.0, 10.0, 9.0, 9.0, 10.0, 6.0, 9.0, 8.0, 6.0, 9.0, 12.0, 9.0, 3.0, 9.0, 10.0, 5.0, 8.0, 10.0, 3.0, 10.0, 8.0, 12.0, 13.0, 7.0, 9.0, 10.0, 11.0, 9.0, 4.0, 7.0, 7.0, 7.0, 4.0, 8.0, 7.0, 4.0, 4.0, 10.0, 5.0, 7.0, 12.0, 12.0, 6.0, 11.0, 8.0, 10.0, 12.0, 9.0, 12.0, 7.0, 9.0, 9.0, 4.0, 8.0, 7.0, 7.0, 14.0, 7.0, 10.0, 7.0, 7.0, 15.0, 9.0, 8.0, 12.0, 7.0, 6.0, 12.0, 3.0, 6.0, 4.0, 11.0, 5.0, 9.0, 6.0, 10.0, 6.0, 14.0, 4.0, 7.0, 6.0, 4.0, 11.0, 17.0, 7.0, 12.0, 9.0, 7.0, 9.0, 4.0, 11.0, 10.0, 10.0, 9.0, 4.0, 10.0, 7.0, 7.0, 10.0, 9.0, 11.0, 8.0, 9.0, 7.0, 10.0, 12.0, 6.0, 10.0, 8.0, 4.0, 10.0, 8.0, 13.0, 6.0, 5.0, 5.0, 9.0, 11.0, 11.0, 7.0, 15.0, 9.0, 9.0, 4.0, 10.0, 12.0, 9.0, 6.0, 6.0, 7.0, 5.0, 11.0, 9.0, 4.0, 7.0, 9.0, 9.0, 7.0, 8.0, 11.0, 6.0, 8.0, 7.0, 9.0, 5.0, 12.0, 5.0, 11.0, 7.0, 8.0, 6.0, 7.0, 12.0, 8.0, 10.0, 10.0, 13.0, 9.0, 8.0, 9.0, 9.0, 5.0, 9.0, 8.0, 8.0, 4.0, 8.0, 4.0, 7.0, 11.0, 9.0, 6.0, 6.0, 9.0, 5.0, 8.0, 11.0, 9.0, 9.0, 12.0, 10.0, 7.0, 10.0, 5.0, 5.0, 11.0, 12.0, 6.0, 12.0, 11.0, 6.0, 10.0, 7.0, 10.0, 15.0, 11.0, 8.0, 14.0]
  in  "stop":bool
  in  "Reset Average":bool=TRUE
  in  "Save Data?":bool=TRUE
  in  "Collect Data?":bool=TRUE
  in  "Tab Control":T2(tab)=enum."g/m^3"
  out "Water Vapor Number Density  2":cluster{"Y":dbl[], "Y":dbl[]}[](graph)
  out "Absolute Humidity":cluster{"Y":dbl[], "Y":dbl[]}[](graph)
  out "NRB plot":cluster{"Y":dbl[], "Y":dbl[]}[](graph)
  in  "background length":i32=10
  out "Correction":cluster{"Y":dbl[], "Y":dbl[]}[](graph)
  in  "dead time":dbl=3.7e-08
  out "Optical Depth":cluster{"Y":dbl[], "Y":dbl[]}[](graph) caption="XY Graph"
  out "RingBuffer offline far":dbl[][](array[numeric])
  out "RingBuffer aerosol far":dbl[][](array[numeric])=[[938.9, 988.9, 893.9, 948.9, 1280.9, 1253.9, 768.9, 422.9, 790.9, 1860.9, 2621.9, 3373.9, 3379.9, 2714.9, 2161.9, 2108.9, 2465.9, 2701.9, 2847.9, 3401.9, 4152.9, 3506.9, 2075.9, 750.9, 260.9, 311.9, 222.9, 193.9, 230.9, 338.9, 459.9, 509.9, 544.9, 730.9, 1192.9, 1254.9, 840.9, 406.9, 343.9, 247.9, 82.9, 17.9, 3.9000000000000004, 2.9000000000000004, -0.09999999999999964, -1.0999999999999996, -1.0999999999999996, -2.0999999999999996, -3.0999999999999996, -3.0999999999999996, -2.0999999999999996, -0.09999999999999964, 3.9000000000000004, -1.0999999999999996, 0.9000000000000004, -1.0999999999999996, 1.9000000000000004, -3.0999999999999996, 2.9000000000000004, -1.0999999999999996, 2.9000000000000004, -2.0999999999999996, -0.09999999999999964, -0.09999999999999964, 3.9000000000000004, 1.9000000000000004, -1.0999999999999996, 0.9000000000000004, 1.9000000000000004, -0.09999999999999964, -0.09999999999999964, -2.0999999999999996, -1.0999999999999996, -0.09999999999999964, -1.0999999999999996, -0.09999999999999964, 2.9000000000000004, -0.09999999999999964, 3.9000000000000004, 1.9000000000000004, -0.09999999999999964, -0.09999999999999964, -0.09999999999999964, -0.09999999999999964, 0.9000000000000004, -1.0999999999999996, -0.09999999999999964, -0.09999999999999964, -2.0999999999999996, -0.09999999999999964, -1.0999999999999996, -0.09999999999999964, -5.1, -2.0999999999999996, -2.0999999999999996, 1.9000000000000004, -1.0999999999999996, -3.0999999999999996, -1.0999999999999996, -1.0999999999999996, -0.09999999999999964, -3.0999999999999996, 2.9000000000000004, -2.0999999999999996, -1.0999999999999996, -4.1, -4.1, -1.0999999999999996, -1.0999999999999996, 1.9000000000000004, -4.1, -3.0999999999999996, 2.9000000000000004, -1.0999999999999996, -1.0999999999999996, -3.0999999999999996, -3.0999999999999996, -2.0999999999999996, -2.0999999999999996, -3.0999999999999996, -4.1, 1.9000000000000004, -5.1, 0.9000000000000004, 0.9000000000000004, -1.0999999999999996, -1.0999999999999996, -3.0999999999999996, 0.9000000000000004, -1.0999999999999996, -3.0999999999999996, -5.1, 6.9, 1.9000000000000004, 6.9, -2.0999999999999996, 0.9000000000000004, -0.09999999999999964, -3.0999999999999996, -1.0999999999999996, -2.0999999999999996, -3.0999999999999996, 1.9000000000000004, -4.1, -2.0999999999999996, -2.0999999999999996, 1.9000000000000004, -2.0999999999999996, -3.0999999999999996, -2.0999999999999996, -3.0999999999999996, -4.1, -2.0999999999999996, -1.0999999999999996, -1.0999999999999996, -4.1, -1.0999999999999996, -2.0999999999999996, -0.09999999999999964, -1.0999999999999996, -1.0999999999999996, 1.9000000000000004, -0.09999999999999964, -2.0999999999999996, -0.09999999999999964, -1.0999999999999996, -3.0999999999999996, -2.0999999999999996, -4.1, 0.9000000000000004, -3.0999999999999996, -3.0999999999999996, -2.0999999999999996, -2.0999999999999996, -1.0999999999999996, -2.0999999999999996, 1.9000000000000004, 0.9000000000000004, 2.9000000000000004, -1.0999999999999996, -2.0999999999999996, -4.1, -1.0999999999999996, 1.9000000000000004, 0.9000000000000004, -2.0999999999999996, -1.0999999999999996, -1.0999999999999996, -3.0999999999999996, -1.0999999999999996, 0.9000000000000004, -0.09999999999999964, -0.09999999999999964, 0.9000000000000004, -3.0999999999999996, -2.0999999999999996, -1.0999999999999996, -1.0999999999999996, -4.1, -1.0999999999999996, -1.0999999999999996, -0.09999999999999964, -0.09999999999999964, -2.0999999999999996, -3.0999999999999996, -2.0999999999999996, -0.09999999999999964, -2.0999999999999996, -1.0999999999999996, -2.0999999999999996, -2.0999999999999996, 0.9000000000000004, -2.0999999999999996, -0.09999999999999964, -0.09999999999999964, 0.9000000000000004, -3.0999999999999996, 0.9000000000000004, -1.0999999999999996, -4.1, -2.0999999999999996, -0.09999999999999964, -4.1, -5.1, -2.0999999999999996, -5.1, 0.9000000000000004, -3.0999999999999996, -1.0999999999999996, 0.9000000000000004, 1.9000000000000004, -1.0999999999999996, 2.9000000000000004, -3.0999999999999996, -1.0999999999999996, -1.0999999999999996, -3.0999999999999996, -3.0999999999999996, 2.9000000000000004, -3.0999999999999996, -0.09999999999999964, -1.0999999999999996, -4.1, -0.09999999999999964, -4.1, -0.09999999999999964, -0.09999999999999964, -0.09999999999999964, 0.9000000000000004, -0.09999999999999964, -0.09999999999999964, 0.9000000000000004, -2.0999999999999996, -2.0999999999999996, 4.9, -4.1, -4.1, -1.0999999999999996, -1.0999999999999996, -2.0999999999999996, -0.09999999999999964, -4.1, -2.0999999999999996, -0.09999999999999964, -2.0999999999999996, -0.09999999999999964, 2.9000000000000004, -0.09999999999999964, 0.9000000000000004, -3.0999999999999996, -2.0999999999999996, 2.9000000000000004, -1.0999999999999996, -3.0999999999999996, 2.9000000000000004, -1.0999999999999996, 3.9000000000000004, 1.9000000000000004, -1.0999999999999996]]
  in  "Weather":T3(tab)
  out "Temperature (C)":dbl(graph)=6.141636141636141
  out "Pressure (mb)":dbl(graph)=825.6043956043957
  out "Relative Humdity (%)":dbl(graph)=80.59065934065934
  out "Pulse Energy (Micro Joule)":cluster{dbl}(graph)={4.114285714285715}
  in  "PRF (kHz)":dbl=7.0
  out "?":cluster{"mean":dbl, "mean":dbl}(graph)={"mean"=1019.9999999999999, "mean"=2080.0}
  out "Index":i32=816
  out "Aerosol Smoothed":dbl[](array[numeric])=[963.9, 941.4, 921.4, 1114.9, 1267.4, 1011.4000000000001, 595.9, 606.9, 1325.9, 2241.4, 2997.9, 3376.9, 3047.4, 2438.4, 2135.4, 2287.4, 2583.9, 2774.9, 3124.9, 3777.3999999999996, 3829.8999999999996, 2791.4, 1413.4, 505.9, 286.4, 267.4, 208.4, 212.4, 284.9, 399.4, 484.9, 527.4, 637.9, 961.9000000000001, 1223.9, 1047.9, 623.9, 375.4, 295.9, 165.4, 50.400000000000006, 10.899999999999999, 3.4000000000000004, 1.4000000000000004, -0.5999999999999996, -1.0999999999999996, -1.5999999999999996, -2.5999999999999996, -3.0999999999999996, -2.5999999999999996, -1.0999999999999996, 1.9000000000000004, 1.4000000000000004, -0.09999999999999964, -0.09999999999999964, 0.40000000000000036, -0.5999999999999996, -0.09999999999999964, 0.9000000000000004, 0.9000000000000004, 0.40000000000000036, -1.0999999999999996, -0.09999999999999964, 1.9000000000000004, 2.9000000000000004, 0.40000000000000036, -0.09999999999999964, 1.4000000000000004, 0.9000000000000004, -0.09999999999999964, -1.0999999999999996, -1.5999999999999996, -0.5999999999999996, -0.5999999999999996, -0.5999999999999996, 1.4000000000000004, 1.4000000000000004, 1.9000000000000004, 2.9000000000000004, 0.9000000000000004, -0.09999999999999964, -0.09999999999999964, -0.09999999999999964, 0.40000000000000036, -0.09999999999999964, -0.5999999999999996, -0.09999999999999964, -1.0999999999999996, -1.0999999999999996, -0.5999999999999996, -0.5999999999999996, -2.5999999999999996, -3.5999999999999996, -2.0999999999999996, -0.09999999999999964, 0.40000000000000036, -2.0999999999999996, -2.0999999999999996, -1.0999999999999996, -0.5999999999999996, -1.5999999999999996, -0.09999999999999964, 0.40000000000000036, -1.5999999999999996, -2.5999999999999996, -4.1, -2.5999999999999996, -1.0999999999999996, 0.40000000000000036, -1.0999999999999996, -3.5999999999999996, -0.09999999999999964, 0.9000000000000004, -1.0999999999999996, -2.0999999999999996, -3.0999999999999996, -2.5999999999999996, -2.0999999999999996, -2.5999999999999996, -3.5999999999999996, -1.0999999999999996, -1.5999999999999996, -2.0999999999999996, 0.9000000000000004, -0.09999999999999964, -1.0999999999999996, -2.0999999999999996, -1.0999999999999996, -0.09999999999999964, -2.0999999999999996, -4.1, 0.9000000000000004, 4.4, 4.4, 2.4000000000000004, -0.5999999999999996, 0.40000000000000036, -1.5999999999999996, -2.0999999999999996, -1.5999999999999996, -2.5999999999999996, -0.5999999999999996, -1.0999999999999996, -3.0999999999999996, -2.0999999999999996, -0.09999999999999964, -0.09999999999999964, -2.5999999999999996, -2.5999999999999996, -2.5999999999999996, -3.5999999999999996, -3.0999999999999996, -1.5999999999999996, -1.0999999999999996, -2.5999999999999996, -2.5999999999999996, -1.5999999999999996, -1.0999999999999996, -0.5999999999999996, -1.0999999999999996, 0.40000000000000036, 0.9000000000000004, -1.0999999999999996, -1.0999999999999996, -0.5999999999999996, -2.0999999999999996, -2.5999999999999996, -3.0999999999999996, -1.5999999999999996, -1.0999999999999996, -3.0999999999999996, -2.5999999999999996, -2.0999999999999996, -1.5999999999999996, -1.5999999999999996, -0.09999999999999964, 1.4000000000000004, 1.9000000000000004, 0.9000000000000004, -1.5999999999999996, -3.0999999999999996, -2.5999999999999996, 0.40000000000000036, 1.4000000000000004, -0.5999999999999996, -1.5999999999999996, -1.0999999999999996, -2.0999999999999996, -2.0999999999999996, -0.09999999999999964, 0.40000000000000036, -0.09999999999999964, 0.40000000000000036, -1.0999999999999996, -2.5999999999999996, -1.5999999999999996, -1.0999999999999996, -2.5999999999999996, -2.5999999999999996, -1.0999999999999996, -0.5999999999999996, -0.09999999999999964, -1.0999999999999996, -2.5999999999999996, -2.5999999999999996, -1.0999999999999996, -1.0999999999999996, -1.5999999999999996, -1.5999999999999996, -2.0999999999999996, -0.5999999999999996, -0.5999999999999996, -1.0999999999999996, -0.09999999999999964, 0.40000000000000036, -1.0999999999999996, -1.0999999999999996, -0.09999999999999964, -2.5999999999999996, -3.0999999999999996, -1.0999999999999996, -2.0999999999999996, -4.6, -3.5999999999999996, -3.5999999999999996, -2.0999999999999996, -1.0999999999999996, -2.0999999999999996, -0.09999999999999964, 1.4000000000000004, 0.40000000000000036, 0.9000000000000004, -0.09999999999999964, -2.0999999999999996, -1.0999999999999996, -2.0999999999999996, -3.0999999999999996, -0.09999999999999964, -0.09999999999999964, -1.5999999999999996, -0.5999999999999996, -2.5999999999999996, -2.0999999999999996, -2.0999999999999996, -2.0999999999999996, -0.09999999999999964, -0.09999999999999964, 0.40000000000000036, 0.40000000000000036, -0.09999999999999964, 0.40000000000000036, -0.5999999999999996, -2.0999999999999996, 1.4000000000000004, 0.40000000000000036, -4.1, -2.5999999999999996, -1.0999999999999996, -1.5999999999999996, -1.0999999999999996, -2.0999999999999996, -3.0999999999999996, -1.0999999999999996, -1.0999999999999996, -1.0999999999999996, 1.4000000000000004, 1.4000000000000004, 0.40000000000000036, -1.0999999999999996, -2.5999999999999996, 0.40000000000000036, 0.9000000000000004, -2.0999999999999996, -0.09999999999999964, 0.9000000000000004, 1.4000000000000004, 2.9000000000000004]
  out "Off-Line  Bin Readings":dbl[](array[numeric])=[944.0, 994.0, 899.0, 954.0, 1286.0, 1259.0, 774.0, 428.0, 796.0, 1866.0, 2627.0, 3379.0, 3385.0, 2720.0, 2167.0, 2114.0, 2471.0, 2707.0, 2853.0, 3407.0, 4158.0, 3512.0, 2081.0, 756.0, 266.0, 317.0, 228.0, 199.0, 236.0, 344.0, 465.0, 515.0, 550.0, 736.0, 1198.0, 1260.0, 846.0, 412.0, 349.0, 253.0, 88.0, 23.0, 9.0, 8.0, 5.0, 4.0, 4.0, 3.0, 2.0, 2.0, 3.0, 5.0, 9.0, 4.0, 6.0, 4.0, 7.0, 2.0, 8.0, 4.0, 8.0, 3.0, 5.0, 5.0, 9.0, 7.0, 4.0, 6.0, 7.0, 5.0, 5.0, 3.0, 4.0, 5.0, 4.0, 5.0, 8.0, 5.0, 9.0, 7.0, 5.0, 5.0, 5.0, 5.0, 6.0, 4.0, 5.0, 5.0, 3.0, 5.0, 4.0, 5.0, 0.0, 3.0, 3.0, 7.0, 4.0, 2.0, 4.0, 4.0, 5.0, 2.0, 8.0, 3.0, 4.0, 1.0, 1.0, 4.0, 4.0, 7.0, 1.0, 2.0, 8.0, 4.0, 4.0, 2.0, 2.0, 3.0, 3.0, 2.0, 1.0, 7.0, 0.0, 6.0, 6.0, 4.0, 4.0, 2.0, 6.0, 4.0, 2.0, 0.0, 12.0, 7.0, 12.0, 3.0, 6.0, 5.0, 2.0, 4.0, 3.0, 2.0, 7.0, 1.0, 3.0, 3.0, 7.0, 3.0, 2.0, 3.0, 2.0, 1.0, 3.0, 4.0, 4.0, 1.0, 4.0, 3.0, 5.0, 4.0, 4.0, 7.0, 5.0, 3.0, 5.0, 4.0, 2.0, 3.0, 1.0, 6.0, 2.0, 2.0, 3.0, 3.0, 4.0, 3.0, 7.0, 6.0, 8.0, 4.0, 3.0, 1.0, 4.0, 7.0, 6.0, 3.0, 4.0, 4.0, 2.0, 4.0, 6.0, 5.0, 5.0, 6.0, 2.0, 3.0, 4.0, 4.0, 1.0, 4.0, 4.0, 5.0, 5.0, 3.0, 2.0, 3.0, 5.0, 3.0, 4.0, 3.0, 3.0, 6.0, 3.0, 5.0, 5.0, 6.0, 2.0, 6.0, 4.0, 1.0, 3.0, 5.0, 1.0, 0.0, 3.0, 0.0, 6.0, 2.0, 4.0, 6.0, 7.0, 4.0, 8.0, 2.0, 4.0, 4.0, 2.0, 2.0, 8.0, 2.0, 5.0, 4.0, 1.0, 5.0, 1.0, 5.0, 5.0, 5.0, 6.0, 5.0, 5.0, 6.0, 3.0, 3.0, 10.0, 1.0, 1.0, 4.0, 4.0, 3.0, 5.0, 1.0, 3.0, 5.0, 3.0, 5.0, 8.0, 5.0, 6.0, 2.0, 3.0, 8.0, 4.0, 2.0, 8.0, 4.0, 9.0, 7.0, 4.0]
  out "Off-Line Smoothed":dbl[](array[numeric])=[2599.413333333333, 2455.499444444444, 2302.8327777777777, 2215.3272222222217, 2070.8327777777768, 1783.19111111111, 1390.9938888888883, 1098.8744444444442, 1196.8577777777775, 1725.4216666666664, 2411.6494444444443, 2965.077222222222, 3260.5161111111106, 3309.138333333333, 3212.9966666666664, 3222.266111111111, 3793.013333333334, 3965.8327777777786, 2884.452222222222, 1949.710555555555, 1979.8022222222212, 2370.4077777777766, 2618.579999999999, 2588.4633333333322, 2319.64111111111, 1883.6355555555547, 1335.3661111111105, 853.3772222222224, 539.4633333333335, 336.63833333333343, 202.9994444444444, 132.46888888888887, 106.35499999999996, 101.47999999999996, 94.64111111111109, 73.32444444444444, 45.754999999999995, 25.67444444444445, 14.855, 8.491111111111108, 4.413333333333332, 2.4188888888888895, 1.9661111111111116, 1.8855555555555563, 1.5744444444444452, 1.3216666666666668, 1.2800000000000002, 1.2800000000000002, 1.293888888888889, 1.3522222222222224, 1.435555555555556, 1.3466666666666671, 1.1161111111111113, 1.1300000000000003, 1.2161111111111114, 1.0744444444444445, 1.218888888888889, 1.2994444444444446, 1.2022222222222227, 1.299444444444445, 1.1383333333333336, 0.9355555555555556, 1.0022222222222221, 0.9855555555555557, 0.8411111111111111, 0.8716666666666667, 0.8938888888888892, 0.860555555555556, 0.8022222222222224, 0.9327777777777779, 0.9855555555555557, 0.7272222222222222, 0.8050000000000002, 0.9133333333333336, 0.9188888888888889, 0.8050000000000002, 0.8050000000000002, 0.8661111111111113, 0.73, 0.8438888888888888, 0.7411111111111109, 0.7772222222222223, 0.9022222222222223, 0.5855555555555554, 0.416111111111111, 0.48833333333333334, 0.6522222222222221, 0.7244444444444442, 0.6938888888888888, 0.6938888888888889, 0.705, 0.5744444444444444, 0.5966666666666667, 0.5966666666666666, 0.38555555555555543, 0.39111111111111097, 0.40222222222222215, 0.33277777777777773, 0.30222222222222217, 0.4244444444444443, 0.5855555555555554, 0.441111111111111, 0.4494444444444444, 0.6244444444444445, 0.5022222222222222, 0.4355555555555555, 0.5105555555555554, 0.42444444444444435, 0.44944444444444437, 0.4244444444444443, 0.2716666666666665, 0.4633333333333333, 0.5299999999999999, 0.4716666666666665, 0.5716666666666665, 0.44944444444444426, 0.3188888888888887, 0.5411111111111111, 0.4661111111111111, 0.30222222222222206, 0.35222222222222216, 0.41888888888888887, 0.42999999999999994, 0.4077777777777778, 0.45499999999999985, 0.45499999999999985, 0.3244444444444445, 0.25499999999999995, 0.441111111111111, 0.3799999999999999, 0.3633333333333332, 0.4522222222222221, 0.3105555555555555, 0.2272222222222223, 0.38000000000000006, 0.41055555555555556, 0.3772222222222221, 0.3411111111111109, 0.355, 0.5188888888888888, 0.5022222222222221, 0.3688888888888888, 0.25499999999999995, 0.16055555555555553, 0.14111111111111105, 0.23555555555555546, 0.26888888888888884, 0.305, 0.44666666666666655, 0.40222222222222215, 0.21333333333333332, 0.14388888888888884, 0.21333333333333335, 0.3161111111111112, 0.4133333333333332, 0.33555555555555544, 0.2411111111111111, 0.13277777777777772, 0.09111111111111113, 0.16333333333333333, 0.17444444444444443, 0.28833333333333333, 0.2911111111111111, 0.29111111111111115, 0.2522222222222223, 0.2466666666666667, 0.33, 0.3244444444444444, 0.20777777777777773, 0.07166666666666666, 0.08000000000000007, 0.07722222222222225, 0.15499999999999997, 0.1716666666666667, 0.14111111111111121, 0.2161111111111111, 0.23555555555555557, 0.09666666666666669, 0.17722222222222223, 0.19111111111111112, 0.03277777777777772, 0.15222222222222212, 0.3938888888888888, 0.35777777777777775, 0.18555555555555553, 0.08833333333333333, 0.024444444444444473, 0.13000000000000003, 0.021666666666666695, 0.0022222222222222088, 0.19388888888888892, -0.017222222222222194, -0.09777777777777777, 0.12999999999999998, 0.057777777777777733, 0.0827777777777778, 0.10500000000000004, 0.11611111111111101, 0.08833333333333324, 0.0383333333333333, 0.1383333333333333, 0.19111111111111115, 0.23555555555555555, 0.09388888888888886, -0.03944444444444449, 0.09388888888888883, 0.17444444444444446, 0.18277777777777782, 0.13277777777777777, 0.13833333333333334, 0.16333333333333333, 0.07999999999999999, 0.12444444444444448, -0.0227777777777778, -0.0005555555555556285, 0.23555555555555552, 0.22166666666666665, 0.21611111111111111, 0.1577777777777778, 0.13000000000000006, 0.16055555555555556, 0.1661111111111111, -0.01166666666666659, -0.12555555555555548, -0.05611111111111109, -0.028333333333333335, 0.13833333333333336, 0.26055555555555565, 0.17444444444444449, 0.14944444444444444, 0.052222222222222225, -0.017222222222222153, 0.004999999999999984, -0.0894444444444445, 0.055000000000000056, 0.18277777777777784, 0.09111111111111113, 0.05500000000000002, 0.08555555555555558, 0.13555555555555557, 0.16611111111111115, 0.09388888888888894, -0.02000000000000005, -0.07277777777777783, -0.12833333333333335, -0.14500000000000002, -0.05888888888888891, 0.15777777777777774, 0.20499999999999996, -0.01999999999999997, 0.007777777777777849, 0.20222222222222214, 0.11888888888888877, -0.025555555555555557, 0.03833333333333335, -0.06722222222222227, -0.0894444444444445, 0.010555555555555563, -0.05055555555555553, -0.10333333333333329, -0.00611111111111106, 0.06333333333333335, 0.09666666666666661, 0.07722222222222215, -0.017222222222222312, 0.16055555555555548, 0.2494444444444445, 0.16055555555555565, -0.008888888888888835, -0.11722222222222217, 0.08833333333333332, 0.13555555555555554, 0.016111111111111128, -0.10055555555555555, -0.006111111111111095, 0.09944444444444449, -0.019999999999999983]
  out "On-Line  Smoothed":dbl[](array[numeric])=[2262.0072222222234, 1965.7016666666673, 1696.973888888889, 1500.3961111111112, 1289.8822222222223, 1026.0822222222223, 746.1627777777777, 543.5405555555553, 540.257222222222, 722.5655555555555, 944.9044444444446, 1092.0100000000002, 1126.1155555555556, 1069.851666666667, 972.6322222222225, 917.3600000000002, 1014.7294444444447, 1013.1794444444447, 700.0294444444445, 434.8933333333332, 415.907222222222, 477.57111111111084, 508.9711111111109, 487.3849999999999, 421.1238888888889, 325.6822222222222, 220.6711111111111, 136.09888888888892, 82.37666666666667, 49.93222222222222, 29.415555555555557, 19.154444444444444, 14.77944444444444, 13.421111111111106, 12.565555555555552, 9.45722222222222, 6.318333333333333, 4.087777777777779, 2.6516666666666673, 1.9849999999999999, 1.7599999999999996, 1.5072222222222218, 1.2072222222222222, 1.179444444444444, 1.1711111111111108, 0.9877777777777775, 0.9738888888888888, 1.0044444444444443, 1.0766666666666664, 1.0322222222222222, 0.7683333333333335, 0.8183333333333334, 1.0544444444444443, 0.9988888888888892, 1.0405555555555557, 1.0683333333333331, 0.9044444444444444, 0.7461111111111112, 0.5100000000000001, 0.7211111111111111, 0.9877777777777776, 0.8266666666666667, 0.7461111111111112, 0.7849999999999999, 0.8211111111111111, 0.8516666666666666, 0.7572222222222222, 0.5461111111111112, 0.5933333333333336, 0.537777777777778, 0.4433333333333334, 0.6294444444444445, 0.7461111111111112, 0.7516666666666667, 0.687777777777778, 0.5711111111111112, 0.5211111111111111, 0.5961111111111111, 0.6988888888888889, 0.7155555555555555, 0.5322222222222224, 0.4072222222222223, 0.34888888888888897, 0.3294444444444445, 0.4211111111111111, 0.5405555555555557, 0.4516666666666668, 0.36555555555555574, 0.4183333333333334, 0.21555555555555556, 0.23500000000000007, 0.3544444444444445, 0.3155555555555556, 0.3488888888888891, 0.4294444444444446, 0.3183333333333333, 0.2405555555555556, 0.3072222222222223, 0.2627777777777778, 0.248888888888889, 0.2877777777777778, 0.26833333333333337, 0.24888888888888894, 0.473888888888889, 0.2933333333333335, 0.15166666666666676, 0.3350000000000001, 0.09888888888888893, 0.20166666666666672, 0.4433333333333334, 0.2877777777777778, 0.2544444444444445, 0.34333333333333343, 0.39055555555555566, 0.22666666666666668, 0.1572222222222223, 0.3350000000000001, 0.4100000000000002, 0.36555555555555574, 0.3322222222222223, 0.21555555555555558, 0.2516666666666667, 0.3072222222222223, 0.262777777777778, 0.14055555555555574, 0.17111111111111124, 0.2683333333333334, 0.27388888888888885, 0.1877777777777778, 0.03222222222222228, 0.10166666666666671, 0.10444444444444445, -0.11499999999999994, -0.03722222222222209, 0.2127777777777779, 0.20166666666666672, 0.16833333333333333, 0.15166666666666662, 0.18777777777777777, 0.25722222222222235, 0.10722222222222234, 0.05444444444444449, 0.12666666666666665, 0.1016666666666666, 0.03499999999999998, 0.01277777777777777, 0.12944444444444442, 0.13222222222222224, 0.012777777777777825, -0.10111111111111112, 0.16000000000000011, 0.43777777777777793, 0.32944444444444454, 0.09888888888888901, 0.1516666666666667, 0.19055555555555553, -0.03999999999999997, 0.12111111111111117, 0.2655555555555556, 0.12944444444444445, 0.11, 0.135, 0.18500000000000003, 0.07944444444444448, 0.13777777777777786, 0.18777777777777782, -0.028888888888888898, -0.1372222222222222, -0.12333333333333331, 0.1016666666666667, 0.21000000000000005, 0.09888888888888896, 0.14611111111111116, 0.135, -0.03999999999999996, 0.09055555555555564, 0.11277777777777787, 0.051666666666666694, 0.14055555555555554, 0.029444444444444495, -0.037222222222222115, 0.015555555555555618, 0.02388888888888885, 0.043333333333333286, 0.11277777777777778, 0.10444444444444446, 0.09055555555555558, 0.04611111111111114, -0.04277777777777775, -0.09277777777777774, -0.048333333333333305, 0.07944444444444447, 0.33222222222222236, 0.30166666666666675, 0.07111111111111112, 0.13222222222222227, 0.12111111111111116, 0.007222222222222234, 0.12388888888888892, 0.24611111111111117, 0.2516666666666667, 0.16833333333333333, 0.03500000000000001, 0.03500000000000001, 0.07666666666666667, 0.0822222222222223, 0.23777777777777792, 0.17666666666666675, 0.05444444444444446, 0.04611111111111112, -0.048333333333333325, -0.07888888888888887, 0.06833333333333337, 0.15722222222222224, 0.007222222222222248, -0.08444444444444442, -0.08722222222222223, 0.03777777777777783, 0.018333333333333403, -0.07888888888888887, -0.05111111111111107, -0.02611111111111107, 0.10166666666666668, 0.20722222222222225, 0.06833333333333337, 0.1627777777777778, 0.07666666666666674, -0.1094444444444444, -0.03444444444444441, -0.00944444444444444, 0.1266666666666667, -0.009444444444444394, -0.09000000000000005, -0.08722222222222226, -0.13722222222222222, -0.10388888888888889, -0.02888888888888891, 0.07666666666666666, 0.0016666666666666878, 0.029444444444444492, 0.023888888888888918, -0.15111111111111108, -0.14277777777777773, -0.10388888888888893, -0.06222222222222225, 0.007222222222222251, 0.057222222222222285, -0.1316666666666666, -0.2094444444444444, -0.017777777777777736, 0.02666666666666671, -0.03166666666666666, -0.1455555555555555, -0.20388888888888876, -0.16499999999999992, -0.17333333333333326, -0.12055555555555544, -0.1177777777777777, -0.13999999999999996, 0.0016666666666666757, -0.0566666666666666, -0.02055555555555541, -0.006666666666666585, -0.15388888888888883, -0.14833333333333326, -0.0011111111111110766, 0.05444444444444449, 0.10444444444444448, 0.048888888888888885, -0.07055555555555558, -0.03166666666666664, -0.0011111111111110818, 0.03500000000000003, 0.09611111111111109, 0.08777777777777775, 0.012777777777777773, 0.0211111111111111]
  out "On-Line Bin Readings":dbl[](array[numeric])=[880.0, 850.0, 729.0, 697.0, 802.0, 740.0, 464.0, 217.0, 341.0, 830.0, 1153.0, 1293.0, 1211.0, 904.0, 700.0, 605.0, 666.0, 660.0, 643.0, 790.0, 944.0, 717.0, 396.0, 160.0, 54.0, 53.0, 50.0, 43.0, 43.0, 56.0, 75.0, 69.0, 79.0, 65.0, 158.0, 163.0, 115.0, 50.0, 31.0, 30.0, 14.0, 6.0, 9.0, 8.0, 5.0, 5.0, 8.0, 6.0, 4.0, 5.0, 4.0, 3.0, 4.0, 4.0, 2.0, 6.0, 8.0, 3.0, 5.0, 4.0, 10.0, 11.0, 2.0, 4.0, 7.0, 5.0, 4.0, 9.0, 3.0, 2.0, 4.0, 3.0, 6.0, 7.0, 3.0, 4.0, 7.0, 5.0, 2.0, 7.0, 3.0, 1.0, 0.0, 4.0, 3.0, 2.0, 5.0, 3.0, 5.0, 4.0, 3.0, 1.0, 6.0, 2.0, 3.0, 8.0, 2.0, 6.0, 2.0, 4.0, 3.0, 4.0, 4.0, 5.0, 6.0, 1.0, 3.0, 6.0, 3.0, 6.0, 4.0, 4.0, 4.0, 3.0, 5.0, 5.0, 5.0, 7.0, 5.0, 11.0, 3.0, 5.0, 3.0, 4.0, 6.0, 3.0, 3.0, 3.0, 6.0, 4.0, 5.0, 6.0, 4.0, 1.0, 6.0, 4.0, 5.0, 1.0, 4.0, 4.0, 6.0, 3.0, 2.0, 2.0, 4.0, 1.0, 2.0, 4.0, 4.0, 1.0, 2.0, 5.0, 8.0, 6.0, 6.0, 5.0, 2.0, 4.0, 3.0, 8.0, 5.0, 7.0, 8.0, 4.0, 3.0, 7.0, 4.0, 7.0, 4.0, 0.0, 5.0, 4.0, 2.0, 6.0, 7.0, 5.0, 6.0, 3.0, 2.0, 6.0, 4.0, 4.0, 6.0, 1.0, 6.0, 5.0, 2.0, 4.0, 4.0, 5.0, 5.0, 3.0, 2.0, 2.0, 5.0, 6.0, 3.0, 4.0, 3.0, 4.0, 3.0, 3.0, 9.0, 3.0, 2.0, 2.0, 8.0, 4.0, 5.0, 5.0, 4.0, 4.0, 4.0, 8.0, 6.0, 4.0, 5.0, 4.0, 3.0, 5.0, 6.0, 2.0, 3.0, 3.0, 6.0, 7.0, 3.0, 0.0, 6.0, 5.0, 2.0, 1.0, 5.0, 3.0, 5.0, 6.0, 3.0, 2.0, 3.0, 6.0, 2.0, 6.0, 2.0, 5.0, 2.0, 2.0, 4.0, 3.0, 1.0, 3.0, 6.0, 1.0, 8.0, 4.0, 3.0, 0.0, 5.0, 6.0, 4.0, 5.0, 8.0, 2.0, 4.0, 3.0, 2.0, 7.0, 3.0, 4.0, 3.0, 3.0, 6.0, 3.0, 2.0, 6.0, 5.0, 4.0, 3.0, 4.0, 4.0]
  out "Range Corrected Altitude Array":dbl[](array[numeric])=[5625.0, 22500.0, 50625.0, 90000.0, 140625.0, 202500.0, 275625.0, 360000.0, 455625.0, 562500.0, 680625.0, 810000.0, 950625.0, 1102500.0, 1265625.0, 1440000.0, 1625625.0, 1822500.0, 2030625.0, 2250000.0, 2480625.0, 2722500.0, 2975625.0, 3240000.0, 3515625.0, 3802500.0, 4100625.0, 4410000.0, 4730625.0, 5062500.0, 5405625.0, 5760000.0, 6125625.0, 6502500.0, 6890625.0, 7290000.0, 7700625.0, 8122500.0, 8555625.0, 9000000.0, 9455625.0, 9922500.0, 10400625.0, 10890000.0, 11390625.0, 11902500.0, 12425625.0, 12960000.0, 13505625.0, 14062500.0, 14630625.0, 15210000.0, 15800625.0, 16402500.0, 17015625.0, 17640000.0, 18275625.0, 18922500.0, 19580625.0, 20250000.0, 20930625.0, 21622500.0, 22325625.0, 23040000.0, 23765625.0, 24502500.0, 25250625.0, 26010000.0, 26780625.0, 27562500.0, 28355625.0, 29160000.0, 29975625.0, 30802500.0, 31640625.0, 32490000.0, 33350625.0, 34222500.0, 35105625.0, 36000000.0, 36905625.0, 37822500.0, 38750625.0, 39690000.0, 40640625.0, 41602500.0, 42575625.0, 43560000.0, 44555625.0, 45562500.0, 46580625.0, 47610000.0, 48650625.0, 49702500.0, 50765625.0, 51840000.0, 52925625.0, 54022500.0, 55130625.0, 56250000.0, 57380625.0, 58522500.0, 59675625.0, 60840000.0, 62015625.0, 63202500.0, 64400625.0, 65610000.0, 66830625.0, 68062500.0, 69305625.0, 70560000.0, 71825625.0, 73102500.0, 74390625.0, 75690000.0, 77000625.0, 78322500.0, 79655625.0, 81000000.0, 82355625.0, 83722500.0, 85100625.0, 86490000.0, 87890625.0, 89302500.0, 90725625.0, 92160000.0, 93605625.0, 95062500.0, 96530625.0, 98010000.0, 99500625.0, 101002500.0, 102515625.0, 104040000.0, 105575625.0, 107122500.0, 108680625.0, 110250000.0, 111830625.0, 113422500.0, 115025625.0, 116640000.0, 118265625.0, 119902500.0, 121550625.0, 123210000.0, 124880625.0, 126562500.0, 128255625.0, 129960000.0, 131675625.0, 133402500.0, 135140625.0, 136890000.0, 138650625.0, 140422500.0, 142205625.0, 144000000.0, 145805625.0, 147622500.0, 149450625.0, 151290000.0, 153140625.0, 155002500.0, 156875625.0, 158760000.0, 160655625.0, 162562500.0, 164480625.0, 166410000.0, 168350625.0, 170302500.0, 172265625.0, 174240000.0, 176225625.0, 178222500.0, 180230625.0, 182250000.0, 184280625.0, 186322500.0, 188375625.0, 190440000.0, 192515625.0, 194602500.0, 196700625.0, 198810000.0, 200930625.0, 203062500.0, 205205625.0, 207360000.0, 209525625.0, 211702500.0, 213890625.0, 216090000.0, 218300625.0, 220522500.0, 222755625.0, 225000000.0, 227255625.0, 229522500.0, 231800625.0, 234090000.0, 236390625.0, 238702500.0, 241025625.0, 243360000.0, 245705625.0, 248062500.0, 250430625.0, 252810000.0, 255200625.0, 257602500.0, 260015625.0, 262440000.0, 264875625.0, 267322500.0, 269780625.0, 272250000.0, 274730625.0, 277222500.0, 279725625.0, 282240000.0, 284765625.0, 287302500.0, 289850625.0, 292410000.0, 294980625.0, 297562500.0, 300155625.0, 302760000.0, 305375625.0, 308002500.0, 310640625.0, 313290000.0, 315950625.0, 318622500.0, 321305625.0, 324000000.0, 326705625.0, 329422500.0, 332150625.0, 334890000.0, 337640625.0, 340402500.0, 343175625.0, 345960000.0, 348755625.0, 351562500.0, 354380625.0, 357210000.0, 360050625.0, 362902500.0, 365765625.0, 368640000.0, 371525625.0, 374422500.0, 377330625.0, 380250000.0, 383180625.0, 386122500.0, 389075625.0, 392040000.0, 395015625.0, 398002500.0, 401000625.0, 404010000.0, 407030625.0, 410062500.0, 413105625.0, 416160000.0, 419225625.0, 422302500.0, 425390625.0, 428490000.0, 431600625.0, 434722500.0, 437855625.0, 441000000.0]
  out "Altitude Array (km)":dbl[](array[numeric])=[0.075, 0.15, 0.22499999999999998, 0.3, 0.375, 0.45, 0.5249999999999999, 0.6, 0.6749999999999999, 0.7499999999999999, 0.825, 0.8999999999999999, 0.9749999999999999, 1.05, 1.125, 1.2, 1.275, 1.3499999999999999, 1.4249999999999998, 1.5, 1.575, 1.65, 1.7249999999999999, 1.7999999999999998, 1.8749999999999998, 1.95, 2.025, 2.1, 2.1750000000000003, 2.25, 2.325, 2.4, 2.475, 2.5500000000000003, 2.625, 2.7, 2.775, 2.85, 2.9250000000000003, 3.0, 3.075, 3.15, 3.225, 3.3000000000000003, 3.375, 3.45, 3.525, 3.6, 3.675, 3.75, 3.825, 3.9, 3.975, 4.05, 4.125, 4.2, 4.275, 4.35, 4.425, 4.5, 4.575, 4.65, 4.725, 4.8, 4.875, 4.95, 5.025, 5.1, 5.175, 5.25, 5.325, 5.4, 5.475, 5.55, 5.625, 5.7, 5.775, 5.85, 5.925, 6.0, 6.075, 6.15, 6.225, 6.3, 6.375, 6.45, 6.525, 6.6, 6.675, 6.75, 6.825, 6.9, 6.975, 7.05, 7.125, 7.2, 7.2749999999999995, 7.35, 7.425, 7.5, 7.575, 7.6499999999999995, 7.725, 7.8, 7.875, 7.95, 8.024999999999999, 8.1, 8.174999999999999, 8.249999999999998, 8.325, 8.399999999999999, 8.475, 8.549999999999999, 8.624999999999998, 8.7, 8.774999999999999, 8.85, 8.924999999999999, 8.999999999999998, 9.075, 9.149999999999999, 9.225, 9.299999999999999, 9.374999999999998, 9.45, 9.524999999999999, 9.6, 9.674999999999999, 9.749999999999998, 9.825, 9.899999999999999, 9.975, 10.049999999999999, 10.124999999999998, 10.2, 10.274999999999999, 10.35, 10.424999999999999, 10.499999999999998, 10.575, 10.649999999999999, 10.725, 10.799999999999999, 10.874999999999998, 10.95, 11.024999999999999, 11.1, 11.174999999999999, 11.249999999999998, 11.325, 11.399999999999999, 11.475, 11.549999999999999, 11.624999999999998, 11.7, 11.774999999999999, 11.85, 11.924999999999999, 11.999999999999998, 12.075, 12.149999999999999, 12.225, 12.299999999999999, 12.374999999999998, 12.45, 12.524999999999999, 12.6, 12.674999999999999, 12.749999999999998, 12.825, 12.899999999999999, 12.975, 13.049999999999999, 13.124999999999998, 13.2, 13.274999999999999, 13.35, 13.424999999999999, 13.499999999999998, 13.575, 13.649999999999999, 13.725, 13.799999999999999, 13.874999999999998, 13.95, 14.024999999999999, 14.1, 14.174999999999999, 14.249999999999998, 14.325, 14.399999999999999, 14.474999999999998, 14.549999999999999, 14.624999999999998, 14.7, 14.774999999999999, 14.849999999999998, 14.924999999999999, 14.999999999999998, 15.075, 15.149999999999999, 15.224999999999998, 15.299999999999999, 15.374999999999998, 15.45, 15.524999999999999, 15.599999999999998, 15.674999999999999, 15.749999999999998, 15.825, 15.899999999999999, 15.974999999999998, 16.05, 16.125, 16.2, 16.275, 16.349999999999998, 16.424999999999997, 16.5, 16.575, 16.65, 16.724999999999998, 16.799999999999997, 16.875, 16.95, 17.025, 17.099999999999998, 17.174999999999997, 17.25, 17.325, 17.4, 17.474999999999998, 17.549999999999997, 17.625, 17.7, 17.775, 17.849999999999998, 17.924999999999997, 18.0, 18.075, 18.15, 18.224999999999998, 18.299999999999997, 18.375, 18.45, 18.525, 18.599999999999998, 18.674999999999997, 18.75, 18.825, 18.9, 18.974999999999998, 19.049999999999997, 19.125, 19.2, 19.275, 19.349999999999998, 19.424999999999997, 19.5, 19.575, 19.65, 19.724999999999998, 19.799999999999997, 19.875, 19.95, 20.025, 20.099999999999998, 20.174999999999997, 20.25, 20.325, 20.4, 20.474999999999998, 20.549999999999997, 20.625, 20.7, 20.775, 20.849999999999998, 20.924999999999997, 21.0]
  in  "Instrument Control":T4(tab)=enum."WS"
  out "Readings":T5={"OnLineTEC"=19.5230961, "OnLineLD"=0.148240238, "OffLineTEC"=17.1877079, "OffLineLD"=0.153494149, "EtalonTEC"=26.0435486, "TSOA-TEC"=18.0100346, "Pro8000"=TRUE, "OnLine TEC"=TRUE, "OnLine LD"=TRUE, "OffLine TEC"=TRUE, "OffLine LD"=TRUE, "Etalon TEC"=TRUE, "TSOA TEC"=TRUE} {"OffLineLD" format="%.4g"; "OnLineLD" format="%.4g"; "TSOA-TEC" format="%.3g"; "EtalonTEC" format="%.3g"; "OffLineTEC" format="%.3g"; "OnLineTEC" format="%.3g"}
  in  "Settings":T6={"Module"=enum."On Line LD", "OnLineTEC"=19.52, "OnLineLD"=0.14802799999999902, "OffLineTEC"=17.19, "OffLineLD"=0.15375799999999876, "EtalonTEC"=26.0, "TSOA-TEC"=18.0} {"OffLineLD" min=0.0 max=0.175 step=0.001 format="%.3p"; "OnLineLD" min=0.0 max=0.175 step=0.001 format="%.3p"; "TSOA-TEC" format="%.2g"; "EtalonTEC" format="%.2g"; "OffLineTEC" min=0.0 max=30.0 step=0.1 format="%.2g"; "OnLineTEC" min=0.0 max=30.0 step=0.1 format="%.2g"}
  in  "Pulse B Polarity":enum32{"Low", "High"}(ring)=enum."High"
  in  "Pulse A Delay(ns)":u32=1040 min=80 max=327600
  in  "Pulse B Delay(ns)":u32=170000 min=80 max=327600 step=1
  in  "Accumulation Delay(ns)":u32=10 min=10 max=1270 step=1
  in  "Sync Pulse Polarity":enum32{"Low", "High"}(ring)=enum."High"
  in  "Pulse A Polarity":enum32{"Low", "High"}(ring)=enum."High"
  in  "Number of Bins":u32=280 min=2 max=4095 step=1
  in  "Number of Accumulates":u32=10000 min=1 max=32767 step=1
  in  "Time Resolution Per Bin(ns)":u32=500 min=5 max=1063 step=1
  out "WM Switch":bool
  in  "Cancel online":bool
  in  "Cancel Offline":bool
  in  "Lambda On Set (nm)":dbl=828.193 format="%.5f"
  out "Lambda On Read (nm)":dbl=828.193023532932 format="%.5f"
  out "Lambda Off Read (nm)":dbl=828.2924608551322 format="%.5f"
  in  "Lambda Off Set (nm)":dbl=828.29245 format="%#.5f"
  in  "Bristol In":i32=5
  out "Bristol Out":i32=30
  in  "AB_DIF":dbl=5e-05 format="%#_15g"
  in  "NONAB_DIF":dbl=5e-05 format="%#_15g"
  out "Wavelength Lock Online":bool=TRUE
  out "Wavelength Lock Offline":bool=TRUE
  out "WL Difference":dbl=2.3532932004854956e-05 format="%_7g"
  out "WL Difference off":dbl=1.0855132131837308e-05 format="%_7g"
  in  "calculate absorption cross sections":bool
  in  "Smoothing Range":dbl=150.0
  in  "Total DIAL Integration Time (Minutes)":i32=3
  in  "Data Reads (number of loops)":i32=1
  in  "Total Aerosol Integration Time (Minutes)":dbl=0.02
  in  "Scalar Wait Time":u32=1300
  out "Smoothed Bins":dbl=2.0
  in  "Ophir PM On/Off":bool=TRUE
  out "OphirPM":T7={"Ophir-Ref"=refnum, "Ophir-Device"=1000, "Ophir-Channel"=0}
  out "Average Diode Power":dbl(knob)=0.00144 scale=0.0..0.002 scale format="%.1p"
  out "Ophir Samples":i32=21
  in  "Switch Comm Port":refnum<visa-resource-name>="COM3"
  out "FF_On_Ref":refnum<file>
  out "FF_On_Ptr":i64=109824 format="%.2p"
  out "FF_Off_Ref":refnum<file>
  out "FF_Off_Ptr":i64=109824 format="%.2p"
  out "NF_On_Ref":refnum<file>
  out "NF_On_Ptr":i64=109824 format="%.2p"
  out "NF_Off_Ref":refnum<file>
  out "NF_Off_Ptr":i64=109824 format="%.2p"
  out "DataOpen":bool=TRUE
  out "File Path_Far Field (out)":string="D:\\Micropulse_DIAL_data\\160330FF\\02"
  out "File Path_Near Field (out)":string="D:\\Micropulse_DIAL_data\\160330NF\\02"
  in  "Data File DIR (in)":string="D:\\Micropulse_DIAL_data\\"
  in  "WS_On/Off":bool=TRUE
  in  "WS visa":refnum<visa-resource-name>="Weather"
  out "TRHP":T8={"Temp C"=6.141636141636141, "RelH %"=80.59065934065934, "Press hPa"=825.6043956043957, "AbH g/m^3"=5.723443223443223}
  in  "ADAM6018 IP":string="192.168.0.165"
  out "T_bench":sgl=21.708372
  in  "bins":u32=280 min=2 max=4095 step=1
  out "y offset":u32=10
  in  "ns scale":u32=500
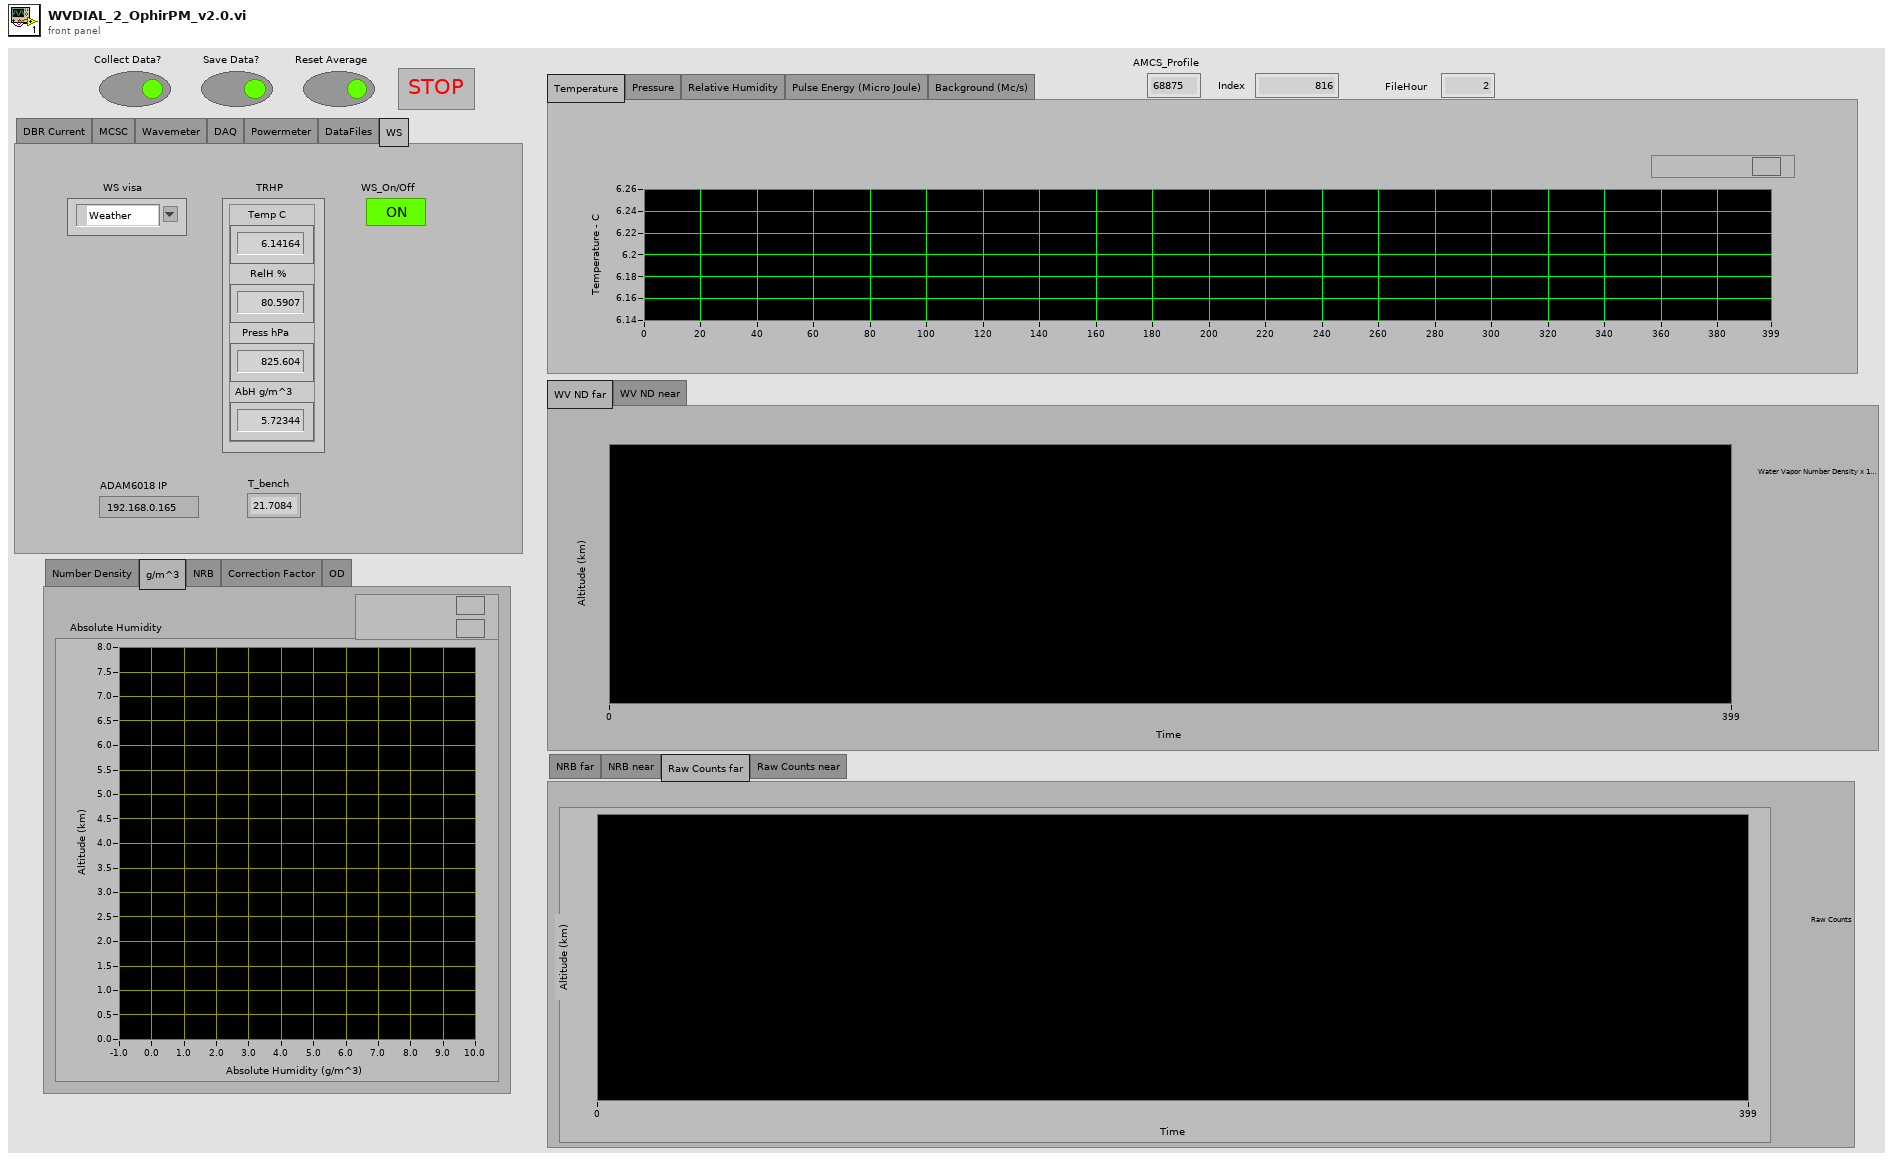
[diagram p1: front panel]
types:
  T1 = enum32{"NRB far", "NRB near", "Raw Counts far", "Raw Counts near"}
  T2 = enum32{"Number Density", "g/m^3", "NRB", "Correction Factor", "OD"}
  T3 = enum32{"Temperature", "Pressure", "Relative Humidity", "Pulse Energy (Micro Joule)", "Background (Mc/s)"}
  T4 = enum32{"DBR Current", "MCSC", "Wavemeter", "DAQ", "Powermeter", "DataFiles", "WS"}
  T5 = cluster{"OnLineTEC":dbl, "OnLineLD":dbl, "OffLineTEC":dbl, "OffLineLD":dbl, "EtalonTEC":dbl, "TSOA-TEC":dbl, "Pro8000":bool, "OnLine TEC":bool, "OnLine LD":bool, "OffLine TEC":bool, "OffLine LD":bool, "Etalon TEC":bool, "TSOA TEC":bool}
  T6 = cluster{"Module":enum16{"On Line TEC", "On Line LD", "Off Line TEC", "Off Line LD", "Etalon TEC", "TSOA TEC"}, "OnLineTEC":dbl, "OnLineLD":dbl, "OffLineTEC":dbl, "OffLineLD":dbl, "EtalonTEC":dbl, "TSOA-TEC":dbl}
  T7 = cluster{"Ophir-Ref":refnum<k7>, "Ophir-Device":i32, "Ophir-Channel":i32}
  T8 = cluster{"Temp C":dbl, "RelH %":dbl, "Press hPa":dbl, "AbH g/m^3":dbl}
  T9 = enum16{"Open_TL", "Close_TL", "Verify_ID", "TEC_Sensor", "SET", "READ", "ON", "OFF", "Set_Limits", "Read_Limits", "Enable_Status", "Read_Status"}
  T10 = enum16{"open", "replace", "create", "open or create", "replace or create", "replace or create with confirmation"}
  T11 = enum16{"On Line TEC", "On Line LD", "Off Line TEC", "Off Line LD", "Etalon TEC", "TSOA TEC"}
  T12 = cluster{"Temp":dbl, "RelH":dbl, "Press":dbl, "AbH":dbl}
  T13 = typedef "LVDateTimeRec.ctl" = cluster{"fractional second":dbl, "second":i32, "minute":i32, "hour":i32, "day of month":i32, "month":i32, "year":i32, "day of week":i32, "day of year":i32, "DST":i32}
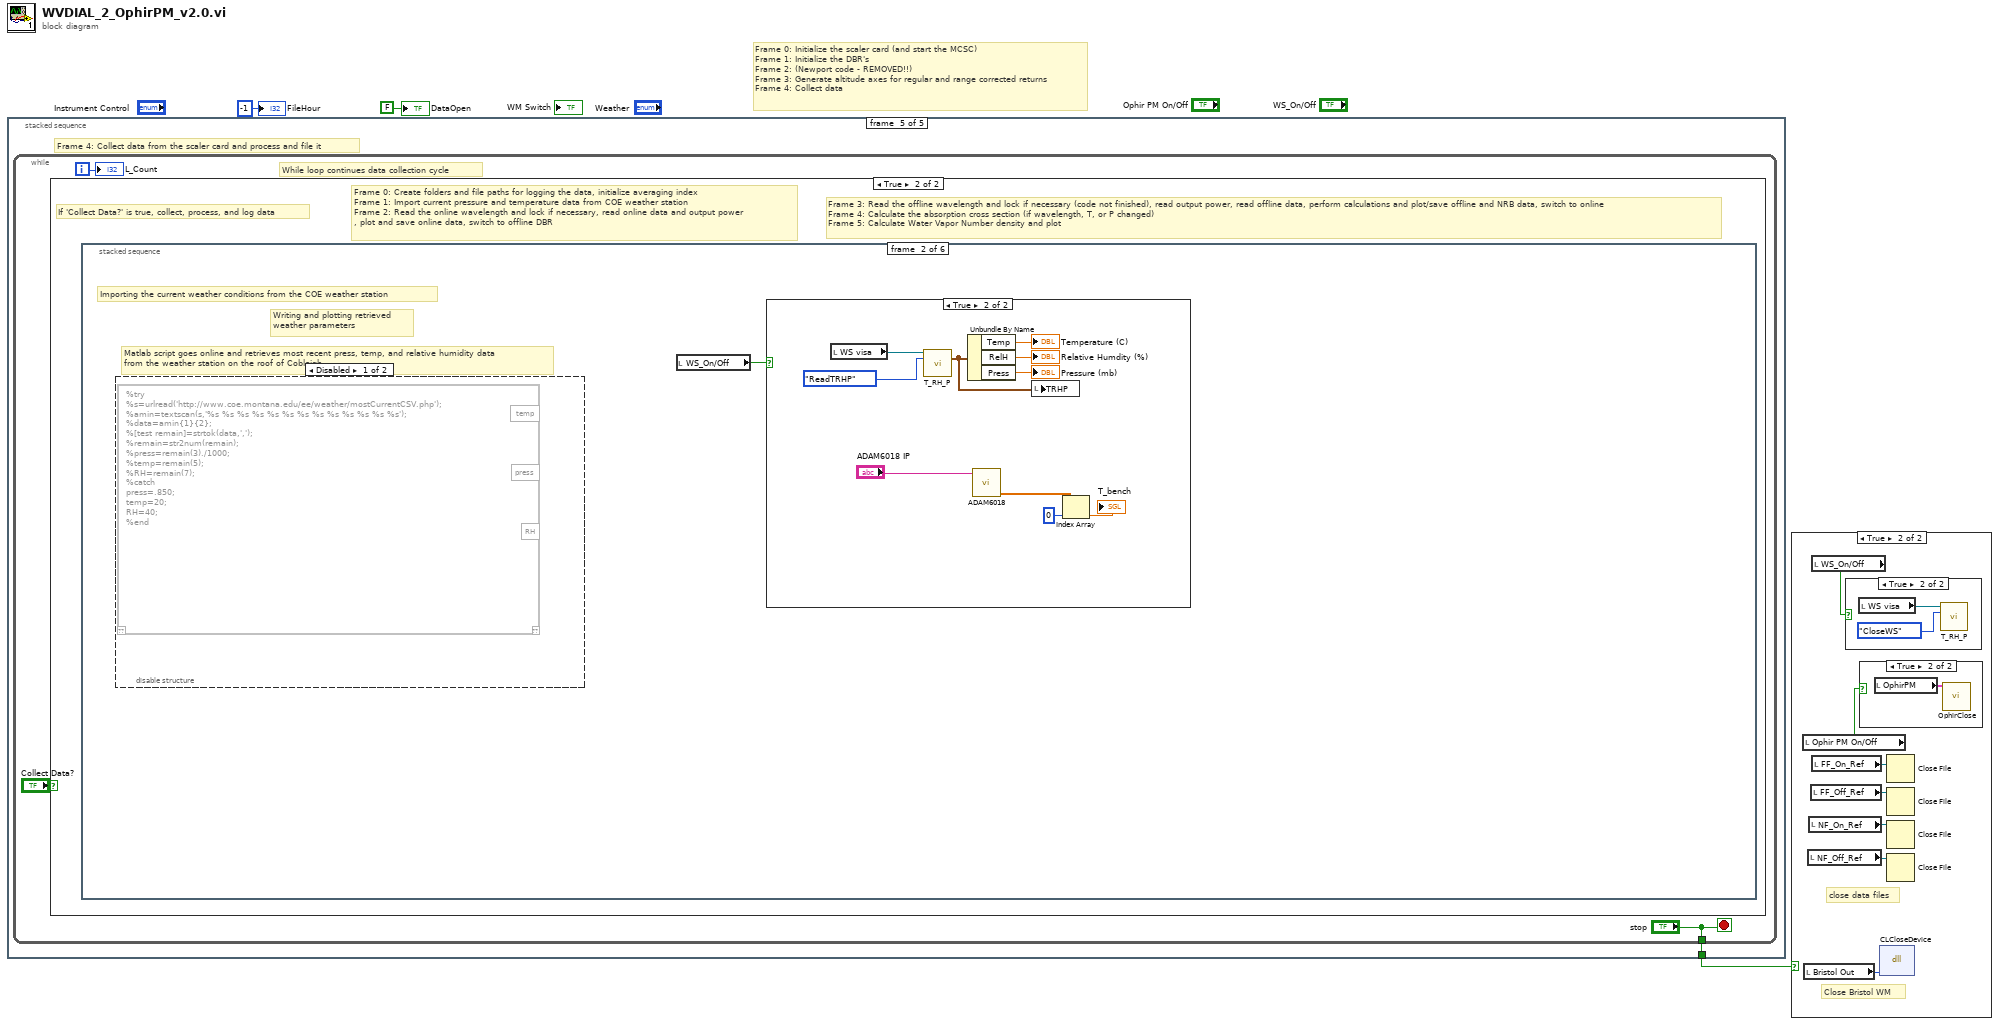
[diagram p0: block diagram]
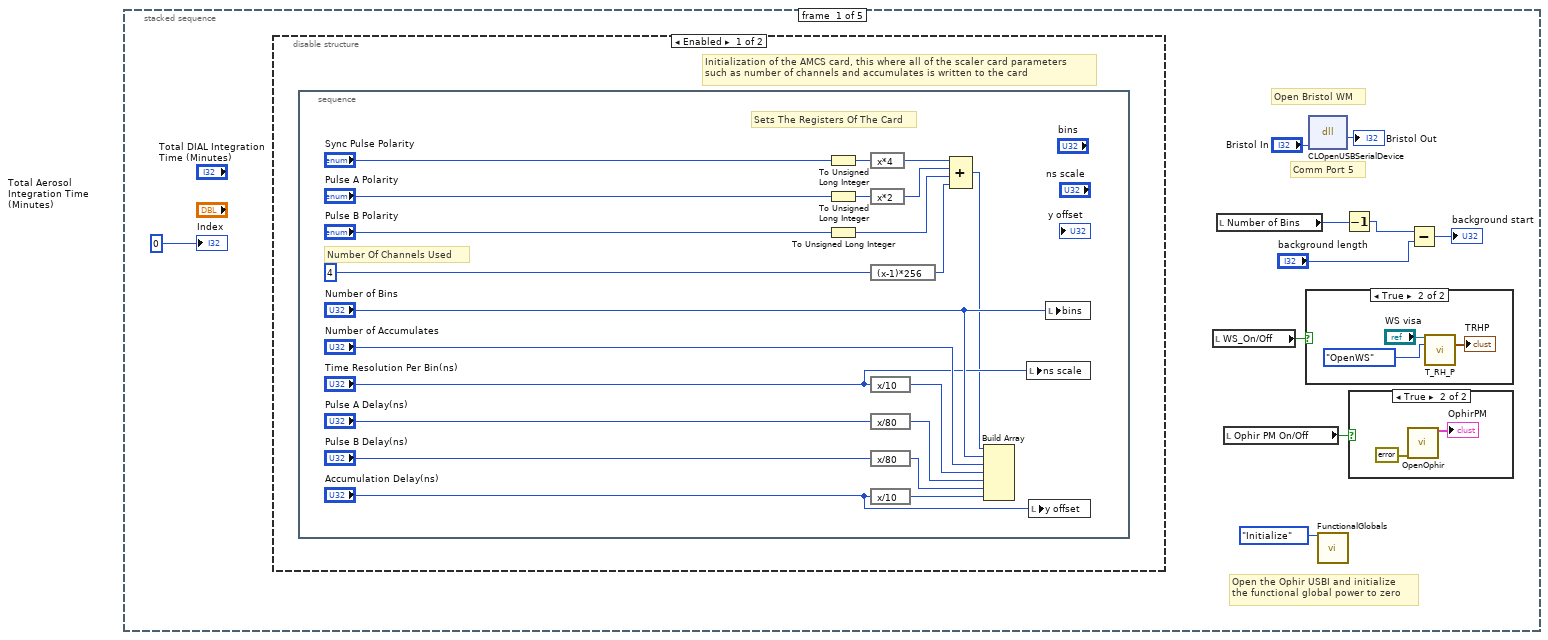
[diagram p5: hidden frame]
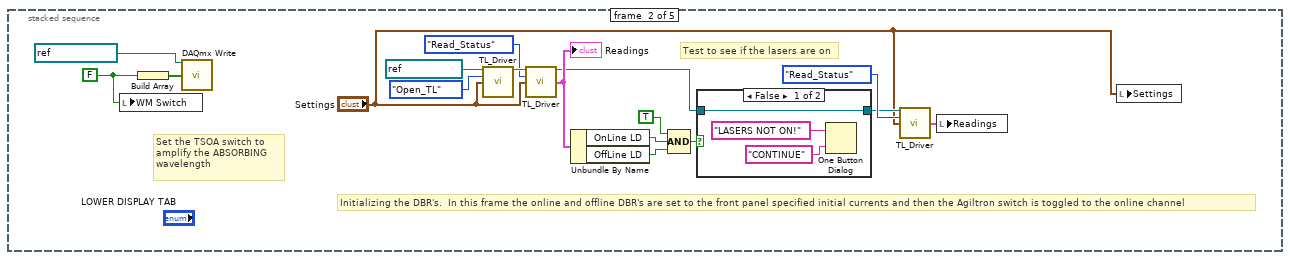
[diagram p9: hidden frame]
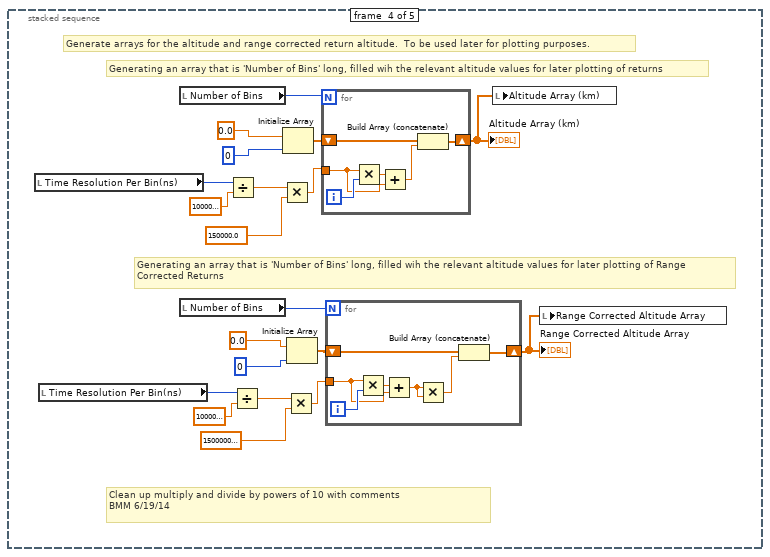
[diagram p12: hidden frame]
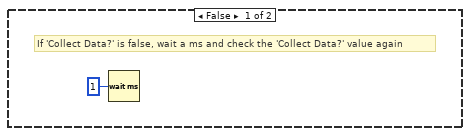
[diagram p13: hidden frame]
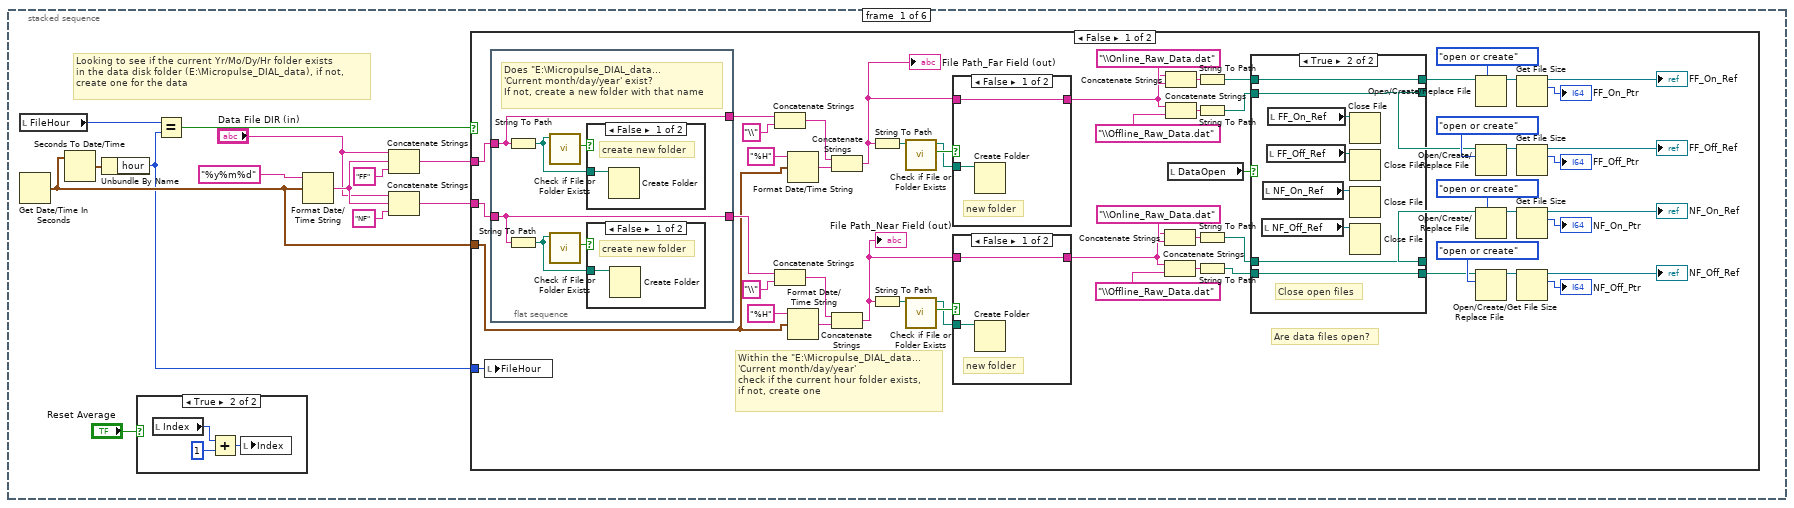
[diagram p14: hidden frame]
diagram:
  # "Frame 0: Initialize the scaler card (and start the MCSC)\nFrame 1: Initialize the DBR's\nFrame 2: (Newport code - REMOVED!!)\nFrame 3: Generate altitude axes for regular and range corrected returns\nFrame 4: Collect data"
  n1 = stacked-sequence {
    tunnel: [_ _ _ _ w94] -> w3
    frame #0 {
      # "Open the Ophir USBI and initialize\nthe functional global power to zero"
      # "Comm Port 5"
      # "Open Bristol WM"
      n2 = disable-structure shown="Enabled" {
        frame Enabled {
          # "Initialization of the AMCS card, this where all of the scaler card parameters\nsuch as number of channels and accumulates is written to the card"
          n3 = stacked-sequence {
            frame #0 {
              # "Sets The Registers Of The Card"
              # "Number Of Channels Used"
              n4 = To Unsigned Long Integer(number="Sync Pulse Polarity") -> (unsigned 32bit integer=w19:u32)
              n5 = To Unsigned Long Integer(number="Pulse A Polarity") -> (unsigned 32bit integer=w23:u32)
              n6 = To Unsigned Long Integer(number="Pulse B Polarity") -> (unsigned 32bit integer=w21:u32)
              n7 = expression code="x*4"(w19) -> (w28:u32)
              n8 = expression code="x*2"(w23) -> (w27:u32)
              n9 = expression code="(x-1)*256"(u32 4 ("Number of Channels Used")) -> (w26:u32)
              n10 = expression code="x/10"("Time Resolution Per Bin(ns)") -> (w30:u32)
              n11 = expression code="x/80"("Pulse A Delay(ns)") -> (w37:u32)
              n12 = expression code="x/80"("Pulse B Delay(ns)") -> (w39:u32)
              n13 = expression code="x/10"("Accumulation Delay(ns)") -> (w38:u32)
              n14 = Compound Arithmetic op=ADD(w28, w27, w21, w26) -> (w25:u32)
              n15 = Build Array(w25, "Number of Bins", "Number of Accumulates", w30, w37, w39, w38) -> ()  [unwired: 1 out]
              n16 = local write "ns scale"("Time Resolution Per Bin(ns)") -> ()
              n17 = local write "y offset"("Accumulation Delay(ns)") -> ()
              n18 = local write "bins"("Number of Bins") -> ()
            }
          }
        }
        frame Disabled {
        }
      }
      n19 = local read "WS_On/Off"() -> (w5:bool)
      n20 = local read "Number of Bins"() -> (w10:u32)
      n21 = local read "Ophir PM On/Off"() -> (w4:bool)
      n22 = case shown="True" w5 {
        frame False {
        }
        frame True {
          n23 = call "T_RH_P.vi"("VISA in"="WS visa", "WS_Commands"=enum16{"OpenWS", "ReadTRHP", "CloseWS"}."OpenWS") -> ("TRHP"=→"TRHP":T12)  [unwired: 11 in, 2 out]
        }
      }
      n24 = dll-call lib="C:/H2O_DIAL/LabVIEW-2012/Bristol WM V2_31b/CLDevIface.dll" fn="CLOpenUSBSerialDevice"("commPort"="Bristol In") -> ("return type"=→"Bristol Out":i32)  [unwired: 4 in, 2 out]
      n25 = call "FunctionalGlobals.vi"("FG_Control"=enum16{"Initialize", "PowerRead", "PowerWrite"}."Initialize") -> ()  [unwired: 14 in, 1 out]
      n26 = Decrement(x=w10) -> (x-1=w9:u32)
      n27 = case shown="True" w4 {
        frame False {
        }
        frame True {
          n28 = call "OpenOphir.vi"("error in (no error)"=errorcluster {"status"=FALSE, "code"=0, "source"=""}) -> ("OphirPM"=→"OphirPM":T7)  [unwired: 13 in, 1 out]
        }
      }
      n29 = Subtract(x=w9, y="background length") -> (x-y=→"background start":u32)
      "Index" <- 0 ("Index")
    }
    frame #1 {
      w40 = FALSE ("Boolean")
      # "Test to see if the lasers are on"
      # "Set the TSOA switch to\namplify the ABSORBING\nwavelength"
      # "Initializing the DBR's.  In this frame the online and offline DBR's are set to the front panel specified initial currents and then the Agiltron switch is toggled to the online channel"
      n30 = local write "WM Switch"(w40) -> ()
      n31 = Build Array(w40) -> (w42:bool[])
      n32 = call-poly <vilib>:"DAQmx Write.vi"("task/channels in"=refnum<k21> "BristolWM", "data"=w42) -> ()  [unwired: 11 in, 3 out]
      n33 = call "TL_Driver.vi"("Device In"=refnum<visa-resource-name> "ThorLabs", "Commands"=T9."Open_TL", "Settings"="Settings") -> ("Device Out"=w54:refnum<visa-resource-name>)  [unwired: 9 in, 3 out]
      n34 = call "TL_Driver.vi"("Device In"=w54, "Commands"=T9."Read_Status", "Settings"="Settings") -> ("Device Out"=w51:refnum<visa-resource-name>, "Readings"=w52:T5)  [unwired: 9 in, 2 out]
      "Readings" <- w52
      n35 = Unbundle By Name(w52) -> ("OnLine LD"=w46:bool, "OffLine LD"=w47:bool)
      n36 = Compound Arithmetic op=AND(TRUE, w46, w47) -> (w45:bool)
      n37 = case shown="False" w45 {
        tunnel: w51 -> [w57 w60]
        tunnel: [w57 w60] -> w49
        frame False {
          n38 = One Button Dialog(message="LASERS NOT ON!", button name ("OK")="CONTINUE") -> ()  [unwired: 1 out]
        }
        frame True {
        }
      }
      n39 = call "TL_Driver.vi"("Device In"=w49, "Commands"=T9."Read_Status", "Settings"="Settings") -> ("Readings"=w41:T5)  [unwired: 9 in, 3 out]
      n40 = local write "Readings"(w41) -> ()
      n41 = local write "Settings"("Settings") -> ()
    }
    frame #2 {
      # "NEWPORT CODE REMOVED!!!!"
    }
    frame #3 {
      # "Clean up multiply and divide by powers of 10 with comments\nBMM 6/19/14"
      # "Generating an array that is 'Number of Bins' long, filled wih the relevant altitude values for later plotting of Range \nCorrected Returns"
      # "Generating an array that is 'Number of Bins' long, filled wih the relevant altitude values for later plotting of returns"
      # "Generate arrays for the altitude and range corrected return altitude.  To be used later for plotting purposes."
      n42 = local read "Time Resolution Per Bin(ns)"() -> (w73:u32)
      n43 = local read "Time Resolution Per Bin(ns)"() -> (w63:u32)
      n44 = local read "Number of Bins"() -> (w76:u32)
      n45 = local read "Number of Bins"() -> (w66:u32)
      n46 = Divide(x=w73, y=1000000000.0) -> (x/y=w71:dbl)
      n47 = Divide(x=w63, y=1000000000.0) -> (x/y=w61:dbl)
      n48 = Multiply(x=w71, y=150000.0) -> (x*y=w74:dbl)
      n49 = Initialize Array(0.0, 0) -> (w79:dbl[])
      n50 = Multiply(x=w61, y=150000000.0) -> (x*y=w64:dbl)
      n51 = Initialize Array(0.0, 0) -> (w69:dbl[])
      n52 = for {
        N: w76 -> [_]
        shift-right: [w92] -> w77
        shift-left: w79 -> [w93]
        tunnel: w74 -> [w89]
        i -> [w91]
        n53 = Multiply(x=w89, y=w91) -> (x*y=w90:dbl)
        n54 = Add(x=w90, y=w89) -> (x+y=w88:dbl)
        n55 = Build Array (concatenate)(w93, w88) -> (w92:dbl[])
      }
      "Altitude Array (km)" <- w77
      n56 = for {
        N: w66 -> [_]
        shift-right: [w86] -> w67
        shift-left: w69 -> [w87]
        tunnel: w64 -> [w82]
        i -> [w85]
        n57 = Multiply(x=w82, y=w85) -> (x*y=w83:dbl)
        n58 = Add(x=w83, y=w82) -> (x+y=w81:dbl)
        n59 = Multiply(x=w81, y=w81) -> (x*y=w84:dbl)
        n60 = Build Array (concatenate)(w87, w84) -> (w86:dbl[])
      }
      "Range Corrected Altitude Array" <- w67
      n61 = local write "Altitude Array (km)"(w77) -> ()
      n62 = local write "Range Corrected Altitude Array"(w67) -> ()
    }
    frame #4 {
      # "Frame 4: Collect data from the scaler card and process and file it"
      n63 = while {
        tunnel: ["stop"] -> w94
        i -> [w95]
        stop <- "stop" stop-if-true
        # "While loop continues data collection cycle"
        n64 = case shown="True" "Collect Data?" {
          frame False {
            # "If 'Collect Data?' is false, wait a ms and check the 'Collect Data?' value again"
            n65 = Wait (ms)(milliseconds to wait=u32 1) -> ()  [unwired: 1 out]
          }
          frame True {
            # "Frame 3: Read the offline wavelength and lock if necessary (code not finished), read output power, read offline data, perform calculations and plot/save offline and NRB data, switch to online\nFrame 4: Calculate the absorption cross section (if wavelength, T, or P changed)\nFrame 5: Calculate Water Vapor Number density and plot"
            # "Frame 0: Create folders and file paths for logging the data, initialize averaging index\nFrame 1: Import current pressure and temperature data from COE weather station\nFrame 2: Read the online wavelength and lock if necessary, read online data and output power\n, plot and save online data, switch to offline DBR"
            # "If 'Collect Data?' is true, collect, process, and log data"
            n66 = stacked-sequence {
              frame #0 {
                # "Looking to see if the current Yr/Mo/Dy/Hr folder exists\nin the data disk folder (E:\\Micropulse_DIAL_data), if not,\ncreate one for the data"
                n67 = local read "FileHour"() -> (w108:i32)
                n68 = Get Date/Time In Seconds() -> (seconds since 1Jan1904=w100:timestamp)
                n69 = Seconds To Date/Time(time stamp (now)=w100) -> (date time rec=w110:T13)  [unwired: 1 in]
                n70 = Unbundle By Name(w110) -> ("hour"=w99:i32)
                n71 = case shown="True" "Reset Average" {
                  frame False {
                    n72 = local write "Index"(0 ("Index")) -> ()
                  }
                  frame True {
                    n73 = local read "Index"() -> (w198:i32)
                    n74 = Add(x=w198, y=1) -> (x+y=w197:i32)
                    n75 = local write "Index"(w197) -> ()
                  }
                }
                n76 = Equal?(x=w108, y=w99) -> (x = y?=w109:bool)
                n77 = Format Date/Time String(time format string (%c)="%y%m%d", seconds (now)=w100) -> (date/time string=w104:string)  [unwired: 1 in]
                n78 = Concatenate Strings("Data File DIR (in)", w104, "FF" ("string")) -> (w106:string)
                n79 = Concatenate Strings("Data File DIR (in)", w104, "NF" ("string")) -> (w101:string)
                n80 = case shown="False" w109 {
                  tunnel: w106 -> [w168 _]
                  tunnel: w101 -> [w167 _]
                  tunnel: w100 -> [w154 _]
                  tunnel: w99 -> [w130 _]
                  frame False {
                    # "Are data files open?"
                    # "Within the \"E:\\Micropulse_DIAL_data...\n'Current month/day/year' \ncheck if the current hour folder exists,\nif not, create one"
                    n81 = local write "FileHour"(w130) -> ()
                    n82 = flat-sequence {
                      tunnel: [w188] -> w155
                      tunnel: w168 -> [w187]
                      tunnel: w167 -> [w188]
                      tunnel: [w187] -> w156
                      frame #0 {
                        # "Does \"E:\\Micropulse_DIAL_data...\n'Current month/day/year' exist?\nIf not, create a new folder with that name"
                        n83 = String To Path(string=w187) -> (path=w192:path)
                        n84 = String To Path(string=w188) -> (path=w190:path)
                        n85 = call <vilib>:"Check if File or Folder Exists.vi"("path"=w192) -> ("file or folder exists?"=w191:bool)  [unwired: 8 in, 2 out]
                        n86 = call <vilib>:"Check if File or Folder Exists.vi"("path"=w190) -> ("file or folder exists?"=w189:bool)  [unwired: 8 in, 2 out]
                        n87 = case shown="False" w191 {
                          tunnel: w192 -> [w194 _]
                          frame False {
                            # "create new folder"
                            n88 = Create Folder(path (use dialog)=w194) -> ()  [unwired: 2 in, 3 out]
                          }
                          frame True {
                            # "Folder exists\ndo nothing"
                          }
                        }
                        n89 = case shown="False" w189 {
                          tunnel: w190 -> [w193 _]
                          frame False {
                            # "create new folder"
                            n90 = Create Folder(path (use dialog)=w193) -> ()  [unwired: 2 in, 3 out]
                          }
                          frame True {
                            # "Folder exists\ndo nothing"
                          }
                        }
                      }
                    }
                    n91 = Concatenate Strings(w156, "\\" ("string")) -> (w163:string)
                    n92 = Concatenate Strings(w155, "\\" ("string")) -> (w158:string)
                    n93 = Format Date/Time String(time format string (%c)="%H", seconds (now)=w154) -> (date/time string=w166:string)  [unwired: 1 in]
                    n94 = Format Date/Time String(time format string (%c)="%H", seconds (now)=w154) -> (date/time string=w161:string)  [unwired: 1 in]
                    n95 = Concatenate Strings(w163, w166) -> (w126:string)
                    "File Path_Far Field (out)" <- w126
                    n96 = Concatenate Strings(w158, w161) -> (w127:string)
                    "File Path_Near Field (out)" <- w127
                    n97 = String To Path(string=w126) -> (path=w164:path)
                    n98 = String To Path(string=w127) -> (path=w159:path)
                    n99 = call <vilib>:"Check if File or Folder Exists.vi"("path"=w164) -> ("file or folder exists?"=w153:bool, "dup path"=w151:path)  [unwired: 8 in, 1 out]
                    n100 = call <vilib>:"Check if File or Folder Exists.vi"("path"=w159) -> ("file or folder exists?"=w152:bool, "dup path"=w150:path)  [unwired: 8 in, 1 out]
                    n101 = case shown="False" w153 {
                      tunnel: w151 -> [w185 _]
                      tunnel: w126 -> [w184 w186]
                      tunnel: [w184 w186] -> w124
                      frame False {
                        # "new folder"
                        n102 = Create Folder(path (use dialog)=w185) -> ()  [unwired: 2 in, 3 out]
                      }
                      frame True {
                        # "Folder exists\ndo nothing"
                      }
                    }
                    n103 = case shown="False" w152 {
                      tunnel: w150 -> [w182 _]
                      tunnel: w127 -> [w181 w183]
                      tunnel: [w181 w183] -> w125
                      frame False {
                        # "new folder"
                        n104 = Create Folder(path (use dialog)=w182) -> ()  [unwired: 2 in, 3 out]
                      }
                      frame True {
                        # "Folder exists\ndo nothing"
                      }
                    }
                    n105 = Concatenate Strings(w125, "\\Online_Raw_Data.dat" ("string")) -> (w144:string)
                    n106 = Concatenate Strings(w125, "\\Offline_Raw_Data.dat" ("string")) -> (w143:string)
                    n107 = Concatenate Strings(w124, "\\Online_Raw_Data.dat" ("string")) -> (w149:string)
                    n108 = Concatenate Strings(w124, "\\Offline_Raw_Data.dat" ("string")) -> (w148:string)
                    n109 = local read "DataOpen"() -> (w141:bool)
                    n110 = String To Path(string=w149) -> (path=w140:path)
                    n111 = String To Path(string=w148) -> (path=w139:path)
                    n112 = String To Path(string=w144) -> (path=w138:path)
                    n113 = String To Path(string=w143) -> (path=w137:path)
                    n114 = case shown="True" w141 {
                      tunnel: w140 -> [w172 w176]
                      tunnel: [w172 w176] -> w134
                      tunnel: w139 -> [w171 w175]
                      tunnel: [w171 w175] -> w133
                      tunnel: w138 -> [w170 w174]
                      tunnel: [w170 w174] -> w132
                      tunnel: [w169 w173] -> w131
                      tunnel: w137 -> [w169 w173]
                      frame False {
                        # "No files open\ndo nothing"
                      }
                      frame True {
                        # "Close open files"
                        n115 = local read "NF_Off_Ref"() -> (w178:refnum<file>)
                        n116 = local read "NF_On_Ref"() -> (w177:refnum<file>)
                        n117 = local read "FF_Off_Ref"() -> (w180:refnum<file>)
                        n118 = local read "FF_On_Ref"() -> (w179:refnum<file>)
                        n119 = Close File(refnum=w179) -> ()  [unwired: 1 in, 2 out]
                        n120 = Close File(refnum=w180) -> ()  [unwired: 1 in, 2 out]
                        n121 = Close File(refnum=w177) -> ()  [unwired: 1 in, 2 out]
                        n122 = Close File(refnum=w178) -> ()  [unwired: 1 in, 2 out]
                      }
                    }
                    n123 = Open/Create/Replace File(file path (use dialog)=w134, operation (0:open)=T10."open or create") -> (refnum out=w120:refnum<file>)  [unwired: 4 in, 2 out]
                    n124 = Open/Create/Replace File(file path (use dialog)=w133, operation (0:open)=T10."open or create") -> (refnum out=w121:refnum<file>)  [unwired: 4 in, 2 out]
                    n125 = Open/Create/Replace File(file path (use dialog)=w132, operation (0:open)=T10."open or create") -> (refnum out=w122:refnum<file>)  [unwired: 4 in, 2 out]
                    n126 = Open/Create/Replace File(file path (use dialog)=w131, operation (0:open)=T10."open or create") -> (refnum out=w123:refnum<file>)  [unwired: 4 in, 2 out]
                    n127 = Get File Size(file=w120) -> (refnum out=→"FF_On_Ref":refnum<file>, size (in bytes)=→"FF_On_Ptr":i64)  [unwired: 1 in, 1 out]
                    n128 = Get File Size(file=w121) -> (refnum out=→"FF_Off_Ref":refnum<file>, size (in bytes)=→"FF_Off_Ptr":i64)  [unwired: 1 in, 1 out]
                    n129 = Get File Size(file=w122) -> (refnum out=→"NF_On_Ref":refnum<file>, size (in bytes)=→"NF_On_Ptr":i64)  [unwired: 1 in, 1 out]
                    n130 = Get File Size(file=w123) -> (refnum out=→"NF_Off_Ref":refnum<file>, size (in bytes)=→"NF_Off_Ptr":i64)  [unwired: 1 in, 1 out]
                  }
                  frame True {
                    # "Don't need to do anything!"
                  }
                }
              }
              frame #1 {
                # "Writing and plotting retrieved\nweather parameters"
                # "Matlab script goes online and retrieves most recent press, temp, and relative humidity data \nfrom the weather station on the roof of Cobleigh"
                # "Importing the current weather conditions from the COE weather station"
                n131 = disable-structure shown="Disabled" {
                  frame Disabled {
                    n132 = script code="%try\n%s=urlread('http://www.coe.montana.edu/ee/weather/mostCurrentCSV.php');\n%amin=textscan(s,'%s %s %s %s %s %s %s %s %s %s %s %s %s');\n%data=amin{1}{2};\n%[test remain]=strtok(data,',');\n%remain=str2num(remain);\n%press=remain(3)./1000;\n%temp=remain(5);\n%RH=remain(7);\n%catch\npress=.850;\ntemp=20;\nRH=40;\n%end"() -> ()  [unwired: 1 in, 4 out]
                  }
                  frame Enabled {
                  }
                }
                n133 = local read "WS_On/Off"() -> (w199:bool)
                n134 = case shown="True" w199 {
                  frame False {
                  }
                  frame True {
                    n135 = local read "WS visa"() -> (w209:refnum<visa-resource-name>)
                    n136 = call "T_RH_P.vi"("VISA in"=w209, "WS_Commands"=enum16{"OpenWS", "ReadTRHP", "CloseWS"}."ReadTRHP") -> ("TRHP"=w204:T12)  [unwired: 11 in, 2 out]
                    n137 = Unbundle By Name(w204) -> ("Temp"=→"Temperature (C)":dbl, "RelH"=→"Relative Humdity (%)":dbl, "Press"=→"Pressure (mb)":dbl)
                    n138 = call "ADAM6018.vi"("Remote IP Address 2"="ADAM6018 IP") -> ("Array"=w202:sgl[])  [unwired: 10 in]
                    n139 = local write "TRHP"(w204) -> ()
                    n140 = Index Array(array=w202, index=0) -> (element=→"T_bench":sgl)
                  }
                }
              }
              frame #2 {
                # "Frame 3: Read, process, and plot online data\nFrame 4: Switch to the offline DBR seed\nFrame 5: Write the data to the folders from Frame 0 of outter sequence"
                # "Frame 0: Read the online wavelength and adjust to locking tolerance if out of range\nFrame 1: Read the output power from the Newport meter, calculate and plot the output pulse energy\nFrame 2: Wait 'Scalar Wait Time' for buffer to clear other wavelength data"
                # "Online"
                n141 = stacked-sequence {
                  frame #0 {
                    # "Read the online wavelength and continue adjusting the online DBR if outside the wavelength tolerance\nuntil it is within tolerance"
                    n142 = while {
                      i -> [w213]
                      stop <- w211 stop-if-true
                      # "Frame 2: Decrement DBR current if above tolerance\nFrame 3: Increment DBR current if below tolerance"
                      # "Frame 0: Read the current wavelength from the wavemeter\nFrame 1: Calculate the difference between desired and actual wavelength"
                      # "Continue reading and adjusting online DBR current until within locking tolerance"
                      n143 = stacked-sequence {
                        tunnel: w213 -> [w215 _ _ _ _]
                        tunnel: [_ _ w222 _ _] -> w212
                        frame #0 {
                          n144 = Equal To 0?(x=w215) -> (x = 0?=w214:bool)
                          n145 = case shown="True" w214 {
                            frame False {
                            }
                            frame True {
                              w216 = FALSE ("Boolean")
                              # "SWITCH to ABSORBING"
                              n146 = Build Array(w216) -> (w217:bool[])
                              n147 = local write "WM Switch"(w216) -> ()
                              n148 = call-poly <vilib>:"DAQmx Write.vi"("task/channels in"=refnum<k21> "BristolWM", "data"=w217) -> ()  [unwired: 11 in, 3 out]
                            }
                          }
                        }
                        frame #1 {
                          # "Read Bristol WM"
                          n149 = local read "Bristol Out"() -> (w219:i32)
                          n150 = dll-call lib="C:/H2O_DIAL/LabVIEW-2012/Bristol WM V2_31b/CLDevIface.dll" fn="CLGetLambdaReading"("devHandle"=w219) -> ("return type"=→"Lambda On Read (nm)":dbl)  [unwired: 4 in, 2 out]
                        }
                        frame #2 {
                          # "If WL difference is within tolerance, stop looping, and illuminate 'Wavelength Lock Online' indicator"
                          # "Calculating the difference between the actual and desired online wavelength"
                          n151 = local read "Lambda On Read (nm)"() -> (w229:dbl)
                          n152 = local read "AB_DIF"() -> (w226:dbl)
                          n153 = Subtract(x=w229, y="Lambda On Set (nm)") -> (x-y=w221:dbl)
                          "WL Difference" <- w221
                          n154 = Multiply(x=-1.0, y=w226) -> (x*y=w227:dbl)
                          n155 = Greater?(x=w221, y=w227) -> (0:w223:bool)
                          n156 = Less?(x=w221, y=w226) -> (x < y?=w224:bool)
                          n157 = And(x=w223, y=w224) -> (x .and. y?=w222:bool)
                          "Wavelength Lock Online" <- w222
                        }
                        frame #3 {
                          # "If the wavelength difference is greater that 0.0002 nm, decrement the \nDBR current by 0.01 mA"
                          n158 = local read "WL Difference"() -> (w232:dbl)
                          n159 = Greater Or Equal?(x=w232, y="AB_DIF") -> (x >= y?=w230:bool)
                          n160 = case shown="True" w230 {
                            frame False {
                              # "Wavelength difference is not greater than 0.0002 nm, do nothing"
                            }
                            frame True {
                              # "Generating a command string\nto decrement the current"
                              # "WL difference is greater than 0.0002 nm,\ndecrement the DBR current by 0.01 mA"
                              n161 = local read "Settings"() -> (w237:T6)
                              n162 = Unbundle By Name(w237) -> ("OnLineLD"=w239:dbl)
                              n163 = Subtract(x=w239, y=3e-06) -> (x-y=w240:dbl)
                              n164 = Bundle By Name(cluster=w237, "OnLineLD"=w240, "Module"=T11."On Line LD") -> (w235:T6)
                              n165 = call "TL_Driver.vi"("Device In"=refnum<visa-resource-name> "ThorLabs", "Commands"=T9."SET", "Settings"=w235) -> ("Readings"=w233:T5)  [unwired: 9 in, 3 out]
                              n166 = local write "Settings"(w235) -> ()
                              n167 = local write "Readings"(w233) -> ()
                            }
                          }
                        }
                        frame #4 {
                          # "If the wavelength difference is less that 0.0002 nm, increment the \nDBR current by 0.01 mA"
                          n168 = local read "WL Difference"() -> (w246:dbl)
                          n169 = local read "AB_DIF"() -> (w244:dbl)
                          n170 = Multiply(x=-1.0, y=w244) -> (x*y=w242:dbl)
                          n171 = Less Or Equal?(x=w246, y=w242) -> (x <= y?=w245:bool)
                          n172 = case shown="True" w245 {
                            frame False {
                              # "WL difference is no <= to -0.0002 nm, do nothing"
                            }
                            frame True {
                              # "WL difference is < -0.0002,\nincrement the DBR current by 0.01 mA"
                              # "Generating a command string\nto decrement the current"
                              n173 = local read "Settings"() -> (w251:T6)
                              n174 = Unbundle By Name(w251) -> ("OnLineLD"=w253:dbl)
                              n175 = Add(x=w253, y=3e-06) -> (x+y=w254:dbl)
                              n176 = Bundle By Name(cluster=w251, "OnLineLD"=w254, "Module"=T11."On Line LD") -> (w248:T6)
                              n177 = call "TL_Driver.vi"("Device In"=refnum<visa-resource-name> "ThorLabs", "Commands"=T9."SET", "Settings"=w248) -> ("Readings"=w247:T5)  [unwired: 9 in, 3 out]
                              n178 = local write "Settings"(w248) -> ()
                              n179 = local write "Readings"(w247) -> ()
                            }
                          }
                        }
                      }
                      n180 = Or(x=w212, y="Cancel online") -> (x .or. y?=w211:bool)
                    }
                  }
                  frame #1 {
                    # "Reading the output power of the laser transmitter from the Ophir power meter, once read, convert to corresponding pulse energy and plot"
                    n181 = local read "Ophir PM On/Off"() -> (w256:bool)
                    n182 = case shown="True" w256 {
                      frame False {
                      }
                      frame True {
                        # "Plotting the online and offling pulse energies"
                        # "Converting to pulse energy, assumes 5 percent pickoff"
                        n183 = local read "OphirPM"() -> (w261:T7)
                        n184 = call "OphirRead.vi"("OphirPM"=w261) -> ("Power (W)"=w257:dbl, "Ophir Samples"=→"Ophir Samples":i32)  [unwired: 12 in, 1 out]
                        "Average Diode Power" <- w257
                        n185 = Multiply(x=w257, y=1000.0) -> (x*y=w265:dbl)
                        n186 = Divide(x=w265, y=0.05) -> (x/y=w263:dbl)
                        n187 = Divide(x=w263, y="PRF (kHz)") -> (x/y=w258:dbl)
                        n188 = Bundle(w258) -> (→"Pulse Energy (Micro Joule)":cluster{dbl})  [unwired: 1 in]
                      }
                    }
                  }
                  frame #2 {
                    # "Wait 'Scalar Wait Time' for the next available batch of scalar card data"
                    n189 = local read "AMCS_Profile"() -> (w267:i32)
                    n190 = disable-structure shown="Disabled" {
                      frame Disabled {
                        # "Waiting 'Scalar Wait Time'"
                        n191 = Wait (ms)(milliseconds to wait="Scalar Wait Time") -> ()  [unwired: 1 out]
                      }
                      frame Enabled {
                      }
                    }
                    n192 = while {
                      tunnel: [w274] -> w268
                      tunnel: [w270] -> _
                      tunnel: w267 -> [w270]
                      stop <- w272 stop-if-true
                      n193 = global read "AMCS_Data.vi" "AMCS_Profile"() -> (w274:i32)
                      n194 = Wait (ms)(milliseconds to wait=u32 10) -> ()  [unwired: 1 out]
                      n195 = Equal?(x=w274, y=w270) -> (x = y?=w273:bool)
                      n196 = case shown="False" w273 {
                        tunnel: [TRUE FALSE] -> w272
                        frame False {
                        }
                        frame True {
                        }
                      }
                    }
                    "AMCS_Profile" <- w268
                  }
                  frame #3 {
                    # "convert time per range bin to meters\nand calculate smoothed bins using\nsmoothing range"
                    # "Plotting online cross section and smoothed online data"
                    # "Calculate the bin by bin mean of the data"
                    # "Collect 'Integration Period (Seconds)' number\nof scalar data"
                    # "Reading, processing, and plotting the online data"
                    n197 = local read "Data Reads (number of loops)"() -> (w302:i32)
                    n198 = for {
                      N: w302 -> [_]
                      tunnel: [w322] -> w314 mode=indexing
                      tunnel: [w323] -> w294 mode=indexing
                      # "Scalar Data is retrieved from Global \nVariable that scaler.vi is writing to,"
                      n199 = disable-structure shown="Disabled" {
                        frame Disabled {
                          n200 = global read "Scalar_Data.vi" "Scalar Data  3"() -> ()  [unwired: 1 out]
                          n201 = global read "Scalar_Data.vi" "Scalar Data"() -> ()  [unwired: 1 out]
                        }
                        frame Enabled {
                        }
                      }
                      n202 = global read "AMCS_Data.vi" "AMCS_Data"() -> (w326:u16[][])
                      n203 = Index Array(array=w326, index (row) #1=0 ("index (row)"), index (row) #2=2 ("index (row)")) -> (element #1=w322:u16[], element #2=w323:u16[])  [unwired: 2 in]
                    }
                    n204 = Transpose 2D Array(2D array=w314) -> (transposed array=w318:u16[][])
                    n205 = Transpose 2D Array(2D array=w294) -> (transposed array=w300:u16[][])
                    n206 = for {
                      tunnel: w318 -> [w328] mode=indexing
                      tunnel: [w327] -> w319 mode=indexing
                      n207 = call-poly <vilib>:"Mean.vi"("X"=w328) -> ("mean"=w327:dbl)  [unwired: 1 out]
                    }
                    n208 = for {
                      tunnel: w300 -> [w321] mode=indexing
                      tunnel: [w320] -> w301 mode=indexing
                      n209 = call-poly <vilib>:"Mean.vi"("X"=w321) -> ("mean"=w320:dbl)  [unwired: 1 out]
                    }
                    n210 = local read "bins"() -> (w293:u32)
                    n211 = Array Subset(array=w319, index=1 ("dimension size"), length=w293) -> (w306:dbl[])
                    n212 = Array Subset(array=w301, index=1 ("dimension size"), length=w293) -> (w298:dbl[])
                    n213 = local read "background length"() -> (w283:i32)
                    n214 = local read "background start"() -> (w284:u32)
                    n215 = Array Size(array=w306) -> (size(s)=w303:i32)
                    n216 = Array Size(array=w298) -> (size(s)=w295:i32)
                    n217 = Initialize Array(1.0 ("element"), w303) -> (w305:dbl[])
                    n218 = Initialize Array(1.0 ("element"), w295) -> (w297:dbl[])
                    n219 = Multiply(x=w306, y=w305) -> (x*y=w307:dbl[])
                    "On-Line Bin Readings" <- w307
                    n220 = Multiply(x=w298, y=w297) -> (x*y=w287:dbl[])
                    "On-Line Bin Readings 2" <- w287
                    n221 = local read "Total DIAL Integration Time (Minutes)"() -> (w310:i32)
                    n222 = local read "Time Resolution Per Bin(ns)"() -> (w279:u32)
                    n223 = Array Subset(array=w307, index=w284, length=w283) -> (w316:dbl[])
                    n224 = Array Subset(array=w287, index=w284, length=w283) -> (w289:dbl[])
                    n225 = call-poly <vilib>:"Mean.vi"("X"=w316) -> ("mean"=w315:dbl)  [unwired: 1 out]
                    n226 = call-poly <vilib>:"Mean.vi"("X"=w289) -> ("mean"=w290:dbl)  [unwired: 1 out]
                    n227 = Divide(x=w310, y=w302) -> (x/y=w308:dbl)
                    n228 = local read "Index"() -> (w288:i32)
                    n229 = Subtract(x=w307, y=w315) -> (x-y=w312:dbl[])
                    n230 = Subtract(x=w287, y=w290) -> (x-y=w291:dbl[])
                    n231 = To Double Precision Float(number=w279) -> (double precision float=w280:dbl)
                    n232 = Multiply(x=w308, y=60.0) -> (x*y=w285:dbl)
                    n233 = Multiply(x=w280, y=0.15) -> (x*y=w282:dbl)
                    n234 = call "Ring Buffer Online Far.vi"("Index"=w288, "Profiles to Average"=w285, "Input Array"=w312) -> ("AvgArray"=w311:dbl[])  [unwired: 7 in, 1 out]
                    n235 = call "Ring Buffer Online Near.vi"("Index"=w288, "Profiles to Average"=w285, "Input Array"=w291) -> ("AvgArray"=w292:dbl[])  [unwired: 7 in, 1 out]
                    n236 = Divide(x="Smoothing Range", y=w282) -> (x/y=w277:dbl)
                    "Smoothed Bins" <- w277
                    n237 = call "Smooth Arrray.vi"("smooth size"=w277, "Raw Array"=w311) -> ("Smoothed Array"=→"On-Line  Smoothed":dbl[])  [unwired: 9 in]
                    n238 = call "Smooth Arrray.vi"("smooth size"=w277, "Raw Array"=w292) -> ("Smoothed Array"=→"On-Line Smoothed 2":dbl[])  [unwired: 9 in]
                    n239 = disable-structure shown="Disabled" {
                      frame Disabled {
                        n240 = script code="format long;\ncounts=sum(Online);\nif counts >=0.5e6\ntime=time;\nelse\ntime=time\nend"() -> ()  [unwired: 3 in, 2 out]
                      }
                      frame Enabled {
                      }
                    }
                  }
                  frame #4 {
                    # "CODE REMOVED!!"
                    # "Toggling the Agiltron switch to the offline DBR seed laser"
                  }
                  frame #5 {
                    # "Save the recently collected online data if 'Save Data?' is true"
                    n241 = case shown="True" "Save Data?" {
                      frame False {
                        # "'Save Data?' is false, do nothing"
                      }
                      frame True {
                        # "'Save Data?' is true, save onfline data to the Data Disk"
                        # "Write only one copy of data at this time"
                        # "Retrieve Julian Date"
                        n242 = local read "Readings"() -> (w337:T5)
                        n243 = local read "Time Resolution Per Bin(ns)"() -> (w335:u32)
                        n244 = local read "Number of Accumulates"() -> (w333:u32)
                        n245 = local read "Number of Bins"() -> (w334:u32)
                        n246 = local write "DataOpen"(TRUE ("DataOpen")) -> ()
                        n247 = local read "Lambda On Read (nm)"() -> (w359:dbl)
                        n248 = local read "On-Line Bin Readings 2"() -> (w357:dbl[])
                        n249 = local read "On-Line Bin Readings"() -> (w361:dbl[])
                        n250 = local read "Average Diode Power"() -> (w358:dbl)
                        n251 = Unbundle By Name(w337) -> ("OnLineLD"=w336:dbl)
                        n252 = To Double Precision Float(number=w335) -> (double precision float=w332:dbl)
                        n253 = To Double Precision Float(number=w334) -> (double precision float=w331:dbl)
                        n254 = To Double Precision Float(number=w333) -> (double precision float=w330:dbl)
                        n255 = call "Julian_Date_2.vi"() -> ("Julian Date"=w360:dbl)  [unwired: 11 in]
                        n256 = Build Array (concatenate)(w360, w359, w336, w358, w332, w331, w330, w361) -> (w352:dbl[])
                        n257 = Build Array (concatenate)(w360, w359, w336, w358, w332, w331, w330, w357) -> (w342:dbl[])
                        n258 = local read "NF_On_Ref"() -> (w340:refnum<file>)
                        n259 = local read "FF_On_Ref"() -> (w356:refnum<file>)
                        n260 = local read "NF_On_Ptr"() -> (w341:i64)
                        n261 = local read "FF_On_Ptr"() -> (w355:i64)
                        n262 = Set File Position(offset (in bytes) (0)=w355, refnum=w356) -> (refnum out=w353:refnum<file>, error out=w350:errorcluster)  [unwired: 2 in]
                        n263 = Set File Position(offset (in bytes) (0)=w341, refnum=w340) -> (refnum out=w346:refnum<file>, error out=w344:errorcluster)  [unwired: 2 in]
                        n264 = Write to Binary File(file (use dialog)=w346, data=w342, error in=w344, 5:FALSE ("prepend array or string size? (T)")) -> (refnum out=w345:refnum<file>, error out=w343:errorcluster)  [unwired: 2 in, 1 out]
                        n265 = Write to Binary File(file (use dialog)=w353, data=w352, error in=w350, 5:FALSE ("prepend array or string size? (T)")) -> (refnum out=w351:refnum<file>, error out=w349:errorcluster)  [unwired: 2 in, 1 out]
                        n266 = Get File Position(4:w343, 7:w345) -> (2:w339:i64)  [unwired: 2 out]
                        n267 = Get File Position(4:w349, 7:w351) -> (2:w348:i64)  [unwired: 2 out]
                        n268 = local write "NF_On_Ptr"(w339) -> ()
                        n269 = local write "FF_On_Ptr"(w348) -> ()
                      }
                    }
                  }
                }
              }
              frame #3 {
                # "Frame 3: Read offline data, calculate aerosol data, and plot offline and normalized relative backscatter\nFrame 4: Swich to online DBR\nFrame 5: Save the offline data and related information"
                # "Frame 0: Read the offline wavelength and lock if necessary, though code is not finished to do so\nFrame 1: Read the output power from the Newport power meter\nFrame 2: Wait 'Scalar Wait Time' for buffers to clear of online contiminated data"
                # "offline"
                n270 = stacked-sequence {
                  frame #0 {
                    # "Every 60 data collection cycles, read the offline DBR wavelength, and if outside of wavelength tolerance, adjust DBR current until within tolerance"
                    n271 = local read "L_Count"() -> (w363:i32)
                    n272 = Quotient & Remainder(x=w363, y=60.0) -> (x-y*floor(x/y)=w364:dbl)  [unwired: 1 out]
                    n273 = Equal To 0?(x=w364) -> (x = 0?=w362:bool)
                    n274 = case shown="True" w362 {
                      frame False {
                      }
                      frame True {
                        n275 = while {
                          i -> [w369]
                          stop <- w367 stop-if-true
                          # "Frame 5 Increment ofline DBR current if below tolerance\nFrame 6: update ILX settings to front pannel"
                          # "Frame 3: Calculating the wavelength difference\nFrame 4:Decrement offline DBR current if above tolerance"
                          # "Frame 0: Read the offline laser wavelength (settle if t=0)"
                          n276 = stacked-sequence {
                            tunnel: w369 -> [w371 _ _ _ _]
                            tunnel: [_ _ w381 _ _] -> w368
                            frame #0 {
                              n277 = Equal To 0?(x=w371) -> (x = 0?=w370:bool)
                              n278 = case shown="True" w370 {
                                frame False {
                                }
                                frame True {
                                w372 = TRUE ("Boolean")
                                # "SWITCH to NON-ABSORBING and wait to settle"
                                n279 = Build Array(w372) -> (w377:bool[])
                                n280 = local write "WM Switch"(w372) -> ()
                                n281 = call-poly <vilib>:"DAQmx Write.vi"("task/channels in"=refnum<k21> "BristolWM", "data"=w377) -> ()  [unwired: 11 in, 3 out]
                                n282 = call "TL_Driver.vi"("Device In"=refnum<visa-resource-name> "ThorLabs", "Commands"=T9."Read_Status") -> ("Readings"=w375:T5)  [unwired: 10 in, 3 out]
                                n283 = local write "Readings"(w375) -> ()
                                n284 = Wait (ms)(milliseconds to wait=u32 3200) -> ()  [unwired: 1 out]
                                }
                              }
                            }
                            frame #1 {
                              # "Read Bristol WM"
                              n285 = local read "Bristol Out"() -> (w379:i32)
                              n286 = dll-call lib="C:/H2O_DIAL/LabVIEW-2012/Bristol WM V2_31b/CLDevIface.dll" fn="CLGetLambdaReading"("devHandle"=w379) -> ("return type"=→"Lambda Off Read (nm)":dbl)  [unwired: 4 in, 2 out]
                            }
                            frame #2 {
                              # "Once locked, stop looping and illuminate 'Wavelength Lock Offline'"
                              # "While loop continues locking process until the wavelength is within tolerance"
                              # "Calculating the difference between the actual and desired \noffline wavelength"
                              n287 = local read "Lambda Off Read (nm)"() -> (w389:dbl)
                              n288 = Subtract(x=w389, y="Lambda Off Set (nm)") -> (x-y=w382:dbl)
                              "WL Difference off" <- w382
                              n289 = local read "NONAB_DIF"() -> (w386:dbl)
                              n290 = Multiply(x=-1.0, y=w386) -> (x*y=w387:dbl)
                              n291 = Greater?(x=w382, y=w387) -> (0:w383:bool)
                              n292 = Less?(x=w382, y=w386) -> (x < y?=w384:bool)
                              n293 = And(x=w383, y=w384) -> (x .and. y?=w381:bool)
                              "Wavelength Lock Offline" <- w381
                              n294 = case shown="True" w381 {
                                frame False {
                                }
                                frame True {
                                w390 = FALSE ("Boolean")
                                # "SWITCH back to ABSORBING and wait to settle"
                                n295 = Build Array(w390) -> (w392:bool[])
                                n296 = local write "WM Switch"(w390) -> ()
                                n297 = call-poly <vilib>:"DAQmx Write.vi"("task/channels in"=refnum<k21> "BristolWM", "data"=w392) -> ()  [unwired: 11 in, 3 out]
                                n298 = Wait (ms)(milliseconds to wait=u32 3200) -> ()  [unwired: 1 out]
                                }
                              }
                            }
                            frame #3 {
                              # "Would adjust the offline wavelength if code was finished"
                              n299 = local read "WL Difference off"() -> (w396:dbl)
                              n300 = Greater Or Equal?(x=w396, y="NONAB_DIF") -> (x >= y?=w394:bool)
                              n301 = case shown="True" w394 {
                                frame False {
                                # "WL difference is not out of range, do nothing"
                                }
                                frame True {
                                # "Generating a command string\nto decrement the current"
                                # "WL difference is greater than 0.0002 nm,\ndecrement the DBR current by 0.01 mA"
                                # "WL difference is out of range, this is where you would decrement\nthe laser current"
                                n302 = local read "Settings"() -> (w401:T6)
                                n303 = Unbundle By Name(w401) -> ("OffLineLD"=w402:dbl)
                                n304 = Subtract(x=w402, y=3e-06) -> (x-y=w403:dbl)
                                n305 = Bundle By Name(cluster=w401, "OffLineLD"=w403, "Module"=T11."Off Line LD") -> (w400:T6)
                                n306 = call "TL_Driver.vi"("Device In"=refnum<visa-resource-name> "ThorLabs", "Commands"=T9."SET", "Settings"=w400) -> ("Readings"=w397:T5)  [unwired: 9 in, 3 out]
                                n307 = local write "Settings"(w400) -> ()
                                n308 = local write "Readings"(w397) -> ()
                                }
                              }
                            }
                            frame #4 {
                              # "This is where you would increment the offline current if below tolerance"
                              n309 = local read "NONAB_DIF"() -> (w407:dbl)
                              n310 = local read "WL Difference off"() -> (w410:dbl)
                              n311 = Multiply(x=-1.0, y=w407) -> (x*y=w406:dbl)
                              n312 = Less Or Equal?(x=w410, y=w406) -> (x <= y?=w409:bool)
                              n313 = case shown="True" w409 {
                                frame False {
                                # "WL difference is not outisde tolerance, do nothing"
                                }
                                frame True {
                                # "Generating a command string\nto decrement the current"
                                # "WL difference is less than 0.0002 nm,\nincrement the DBR current by 0.01 mA"
                                # "Incrementing the current if below tolerance"
                                n314 = local read "Settings"() -> (w414:T6)
                                n315 = Unbundle By Name(w414) -> ("OffLineLD"=w416:dbl)
                                n316 = Add(x=w416, y=3e-06) -> (x+y=w417:dbl)
                                n317 = Bundle By Name(cluster=w414, "OffLineLD"=w417, "Module"=T11."Off Line LD") -> (w415:T6)
                                n318 = call "TL_Driver.vi"("Device In"=refnum<visa-resource-name> "ThorLabs", "Commands"=T9."SET", "Settings"=w415) -> ("Readings"=w411:T5)  [unwired: 9 in, 3 out]
                                n319 = local write "Settings"(w415) -> ()
                                n320 = local write "Readings"(w411) -> ()
                                }
                              }
                            }
                          }
                          n321 = Or(x=w368, y="Cancel Offline") -> (x .or. y?=w367:bool)
                        }
                      }
                    }
                  }
                  frame #1 {
                    # "CODE REMOVED!!!"
                    # "Reading the output power of the laser transmitter from the Ophir power meter, once read, convert to corresponding pulse energy and plot"
                  }
                  frame #2 {
                    # "CODE REMOVED!!!"
                    # "Wait 'Scalar Wait Time' for buffers to clear of online contiminated offline data"
                  }
                  frame #3 {
                    w455 = 1 ("dimension size")
                    w458 = 1
                    # "Plotting the normalized relative \nbackscatter"
                    # "Calculating the normalized relative backscatter"
                    # "Calculating/Plotting smoothed data,\ncross sections etc."
                    # "Pick off data with\nout header"
                    # "Calculate mean bin by bin mean"
                    # "Reading in 'Integration Period (Seconds)' of data"
                    # "Read the offline data from the scalar card, perform smoothing, calculate normalized relative backscatter, and plot"
                    # "File path in MATLAB script is of old dial is:\nF:\\Micropulse DIAL\\Micropulse DIAL Matlab\\\nFinal Overlap Function.mat')];"
                    # "Collects Data From Card,\nSends It To The Chart,\nAnd Saves A Copy As A\nFile If Option Selected On\nFront Panel"
                    n322 = for {
                      N: "Data Reads (number of loops)" -> [_]
                      tunnel: [w491] -> w488 mode=indexing
                      tunnel: [w490] -> w470 mode=indexing
                      # "Read in latest scalar card data from \n'Scalar Data' global variable that \nscaler.vi is writing to, then wait 1 sec\nfor next batch of data"
                      n323 = global read "AMCS_Data.vi" "AMCS_Data"() -> (w492:u16[][])
                      n324 = disable-structure shown="Disabled" {
                        frame Disabled {
                          n325 = global read "Scalar_Data.vi" "Scalar Data  2"() -> ()  [unwired: 1 out]
                          n326 = global read "Scalar_Data.vi" "Scalar Data  4"() -> ()  [unwired: 1 out]
                        }
                        frame Enabled {
                        }
                      }
                      n327 = Index Array(array=w492, index (row) #1=1 ("index (row)"), index (row) #2=3 ("index (row)")) -> (element #1=w491:u16[], element #2=w490:u16[])  [unwired: 2 in]
                    }
                    n328 = local read "Total DIAL Integration Time (Minutes)"() -> (w479:i32)
                    n329 = Divide(x=w479, y="Data Reads (number of loops)") -> (x/y=w477:dbl)
                    n330 = local read "Total Aerosol Integration Time (Minutes)"() -> (w481:dbl)
                    n331 = Multiply(x=w477, y=60.0) -> (x*y=w463:dbl)
                    n332 = local read "background length"() -> (w427:i32)
                    n333 = local read "background start"() -> (w428:u32)
                    n334 = Transpose 2D Array(2D array=w488) -> (transposed array=w487:u16[][])
                    n335 = Transpose 2D Array(2D array=w470) -> (transposed array=w469:u16[][])
                    n336 = Divide(x=w481, y="Data Reads (number of loops)") -> (x/y=w482:dbl)
                    n337 = for {
                      tunnel: w487 -> [w498] mode=indexing
                      tunnel: [w497] -> w489 mode=indexing
                      tunnel: w469 -> [w496] mode=indexing
                      tunnel: [w495] -> _ mode=indexing
                      tunnel: [w495] -> w466 mode=indexing
                      n338 = call-poly <vilib>:"Mean.vi"("X"=w498) -> ("mean"=w497:dbl)  [unwired: 1 out]
                      n339 = call-poly <vilib>:"Mean.vi"("X"=w496) -> ("mean"=w495:dbl)  [unwired: 1 out]
                    }
                    n340 = local read "bins"() -> (w456:u32)
                    n341 = Multiply(x=w482, y=60.0) -> (x*y=w446:dbl)
                    n342 = Array Subset(array=w466, index=w455, length=w456) -> (w467:dbl[])
                    "Off-Line Bin Readings 2" <- w467
                    n343 = Array Subset(array=w489, index=w455, length=w456) -> (w465:dbl[])
                    "Off-Line  Bin Readings" <- w465
                    n344 = Array Subset(array=w467, index=w428, length=w427) -> (w468:dbl[])
                    n345 = Array Subset(array=w465, index=w428, length=w427) -> (w486:dbl[])
                    n346 = local read "Smoothed Bins"() -> (w424:dbl)
                    n347 = call-poly <vilib>:"Mean.vi"("X"=w468) -> ("mean"=w434:dbl)  [unwired: 1 out]
                    n348 = call-poly <vilib>:"Mean.vi"("X"=w486) -> ("mean"=w435:dbl)  [unwired: 1 out]
                    n349 = local read "Index"() -> (w445:i32)
                    n350 = Subtract(x=w467, y=w434) -> (x-y=w447:dbl[])
                    n351 = Subtract(x=w465, y=w435) -> (x-y=w461:dbl[])
                    n352 = call "Ring Buffer Offline Far.vi"("Index"=w445, "Profiles to Average"=w463, "Input Array"=w461) -> ("AvgArray"=w484:dbl[], "RingBufferOut"=→"RingBuffer offline far":dbl[][])  [unwired: 7 in]
                    n353 = call "Ring Buffer Aerosol Far.vi"("Index"=w445, "Profiles to Average"=w446, "Input Array"=w461) -> ("AvgArray"=w480:dbl[], "RingBufferOut"=→"RingBuffer aerosol far":dbl[][])  [unwired: 7 in]
                    n354 = call "Ring Buffer Offline Near.vi"("Index"=w445, "Profiles to Average"=w463, "Input Array"=w447) -> ("AvgArray"=w464:dbl[], "RingBufferOut"=→"RingBuffer offline near":dbl[][])  [unwired: 7 in]
                    n355 = call "Ring Buffer Aerosol Near.vi"("Index"=w445, "Profiles to Average"=w446, "Input Array"=w447) -> ("AvgArray"=w443:dbl[], "RingBufferOut"=→"RingBuffer aerosol near":dbl[][])  [unwired: 7 in]
                    n356 = Reshape Array(w461, w455, w456) -> (→"raw counts":dbl[][])
                    n357 = Reshape Array(w447, w455, w456) -> (→"raw counts near":dbl[][])
                    n358 = call "Smooth Arrray.vi"("smooth size"=w424, "Raw Array"=w484) -> ("Smoothed Array"=→"Off-Line Smoothed":dbl[])  [unwired: 9 in]
                    n359 = call "Smooth Arrray.vi"("smooth size"=w424, "Raw Array"=w480) -> ("Smoothed Array"=w454:dbl[])  [unwired: 9 in]
                    "Aerosol Smoothed" <- w454
                    n360 = call "Smooth Arrray.vi"("smooth size"=w424, "Raw Array"=w464) -> ("Smoothed Array"=→"Off-Line Smoothed 2":dbl[])  [unwired: 9 in]
                    n361 = call "Smooth Arrray.vi"("smooth size"=w424, "Raw Array"=w443) -> ("Smoothed Array"=w426:dbl[])  [unwired: 9 in]
                    "Aerosol Smoothed 2" <- w426
                    n362 = local read "Number of Accumulates"() -> (w430:u32)
                    n363 = local read "Temperature (C)"() -> (w476:dbl)
                    n364 = local read "Pressure (mb)"() -> (w475:dbl)
                    n365 = script code="%accum_num=10000;     % scaler card setting number of accumulations\nt_bin = 500e-9                 % scaler card setting time per bin\n%t_d = 37.3e-9;                % APD dead time from spec sheet\n\n% conversion from accumulated counts to count rate  (c/s)\nc_convert = 1./t_bin./accum_num;\nCR_far = p_raw_far.*c_convert;\nCR_near = p_raw_near.*c_convert;\nCR_total_far = (p_raw_far+b_far).*c_convert;\nCR_total_near = (p_raw_near+b_near).*c_convert;\nb_CR_far =b_far.*c_convert;\nb_CR_near =b_near.*c_convert;\n\n% create a range array\nsize_p =  size(p_raw_far,2);\nr = (75:75:size_p*75)./1e3; \n    \n%APD correction factor\n D_far = 1./(1-(t_d*CR_total_far));\n D_near = 1./(1-(t_d*CR_total_near));\n\n %Calculating normalize relative backscatter profile\n nrb_far = CR_far.*D_far.*r.^2./E.*1e-6;\n nrb_near = CR_near.*D_near.*r.^2./E.*1e-6;"("E"=6.0 ("Real"), "temp"=w476, "press"=w475, "p_raw_far"=w454, "b_far"=w435, "b_near"=w434, "p_raw_near"=w426, "accum_num"=w430, "t_d"="dead time") -> ("nrb_far"=w449:cdb[], "D_far"=w440:dbl[], "nrb_near"=w448:cdb[], "D_near"=w439:dbl[], "b_CR_far"=w432:dbl, "b_CR_near"=w431:dbl)  [unwired: 1 in, 1 out]
                    n366 = local read "bins"() -> (w457:u32)
                    n367 = local read "Altitude Array (km)"() -> (w451:dbl[])
                    n368 = Bundle(w432, w431) -> (→"?":cluster{dbl, dbl})  [unwired: 1 in]
                    n369 = Build Array(w449, w448) -> (w453:cdb[][])
                    n370 = Build Array(w440, w439) -> (w438:dbl[][])
                    n371 = Reshape Array(w448, w458, w457) -> (w423:cdb[][])
                    n372 = Reshape Array(w449, w458, w457) -> (w421:cdb[][])
                    n373 = Build Array(w451, w451) -> (w450:dbl[][])
                    n374 = call "Convert to Dynamic Data7"("2D Array"=w438) -> ("Dynamic Data Type"=w437:dynamicdata)  [unwired: 3 in]
                    n375 = call "Convert to Dynamic Data3"("2D Array"=w453) -> ("Dynamic Data Type"=w452:dynamicdata)  [unwired: 3 in]
                    n376 = Logarithm Base 10(1:w421) -> (0:→"NRB":cdb[][])
                    n377 = call "Convert to Dynamic Data4"("2D Array"=w450) -> ("Dynamic Data Type"=w441:dynamicdata)  [unwired: 3 in]
                    n378 = Logarithm Base 10(1:w423) -> (0:→"NRB 2":cdb[][])
                    n379 = call "Build XY Graph2"("Y Input"=w441, "X Input"=w452) -> ("XY Graph"=→"NRB plot":cluster{"Y":dbl[], "Y":dbl[]}[])  [unwired: 3 in, 6 out]
                    n380 = call "Build XY Graph4"("Y Input"=w441, "X Input"=w437) -> ("XY Graph"=→"Correction":cluster{"Y":dbl[], "Y":dbl[]}[])  [unwired: 3 in, 6 out]
                  }
                  frame #4 {
                    # "CODE REMOVED!!!"
                    # "Toggle Agiltron switch to online DBR"
                  }
                  frame #5 {
                    # "If 'Save Data?' is true, save all relavant offline info"
                    n381 = local read "Save Data?"() -> (w499:bool)
                    n382 = case shown="True" w499 {
                      frame False {
                        # "'Save Data?' is false, do nothing"
                      }
                      frame True {
                        # "Write only one data file at this time"
                        # "Retrive Julian Date"
                        # "'Save Data?' is true, save offline data to the Data Disk"
                        n383 = local read "Readings"() -> (w501:T5)
                        n384 = local read "Off-Line Bin Readings 2"() -> (w520:dbl[])
                        n385 = local read "Lambda Off Read (nm)"() -> (w522:dbl)
                        n386 = local read "Off-Line  Bin Readings"() -> (w527:dbl[])
                        n387 = local read "Relative Humdity (%)"() -> (w526:dbl)
                        n388 = local read "Temperature (C)"() -> (w524:dbl)
                        n389 = Unbundle By Name(w501) -> ("OffLineLD"=w500:dbl)
                        n390 = local read "T_bench"() -> (w523:sgl)
                        n391 = local read "Pressure (mb)"() -> (w525:dbl)
                        n392 = call "Julian_Date_2.vi"() -> ("Julian Date"=w521:dbl)  [unwired: 11 in]
                        n393 = Build Array (concatenate)(w521, w522, w500, w523, w524, w525, w526, w527) -> (w506:dbl[])
                        n394 = Build Array (concatenate)(w521, w522, w500, w523, w524, w525, w526, w520) -> (w503:dbl[])
                        n395 = local read "FF_Off_Ref"() -> (w508:refnum<file>)
                        n396 = local read "NF_Off_Ref"() -> (w505:refnum<file>)
                        n397 = local read "FF_Off_Ptr"() -> (w507:i64)
                        n398 = local read "NF_Off_Ptr"() -> (w504:i64)
                        n399 = Set File Position(offset (in bytes) (0)=w507, refnum=w508) -> (refnum out=w519:refnum<file>, error out=w517:errorcluster)  [unwired: 2 in]
                        n400 = Set File Position(offset (in bytes) (0)=w504, refnum=w505) -> (refnum out=w515:refnum<file>, error out=w513:errorcluster)  [unwired: 2 in]
                        n401 = Write to Binary File(file (use dialog)=w519, data=w506, error in=w517, 5:FALSE ("prepend array or string size? (T)")) -> (refnum out=w518:refnum<file>, error out=w516:errorcluster)  [unwired: 2 in, 1 out]
                        n402 = Write to Binary File(file (use dialog)=w515, data=w503, error in=w513, 5:FALSE ("prepend array or string size? (T)")) -> (refnum out=w514:refnum<file>, error out=w512:errorcluster)  [unwired: 2 in, 1 out]
                        n403 = Get File Position(4:w516, 7:w518) -> (2:w509:i64)  [unwired: 2 out]
                        n404 = Get File Position(4:w512, 7:w514) -> (2:w502:i64)  [unwired: 2 out]
                        n405 = local write "FF_Off_Ptr"(w509) -> ()
                        n406 = local write "NF_Off_Ptr"(w502) -> ()
                      }
                    }
                  }
                }
              }
              frame #4 {
                n407 = First Call?() -> (First Call?: T/F=w530:bool)
                n408 = Or(x="calculate absorption cross sections", y=w530) -> (x .or. y?=w528:bool)
                n409 = case shown="True" w528 {
                  frame False {
                  }
                  frame True {
                    # "calculate absorption cross sections from HITRAN data base"
                    n410 = local read "Off-Line Smoothed"() -> (w531:dbl[])
                    n411 = local read "Lambda On Read (nm)"() -> (w534:dbl)
                    n412 = local read "Lambda Off Set (nm)"() -> (w537:dbl)
                    n413 = local read "Temperature (C)"() -> (w535:dbl)
                    n414 = local read "Pressure (mb)"() -> (w536:dbl)
                    n415 = script code="hitran = dlmread('C:\\H2O_DIAL\\LabVIEW-2012\\Micropulse DIAL Matlab\\815nm_841nm_HITRAN_2008.csv', ',',[1 1 1676 8]);\n%hitran = dlmread('C:\\H2O_DIAL\\LabVIEW-2012\\Micropulse DIAL Matlab\\824nm_841nm_H2O_Spectral_Calc.csv', ',',[1 1 1209 7]);\n\n\n\n%Range vector in meters\nrange = ([75:75:size(Online,2)*75]);\n\nif lambda< 828\nlambda=828.195;\nelse\nlambda=lambda;\nend;\n\n%%\n\n%Voigt profile calculation\nWNmin = 1/(828+4)*1e7;  % 832.0 nm converted to wavenumber\nWNmax = 1/(828-4)*1e7;  % 824.0 nm converted to wavenumber\n\n%Find lines from WNmin to WNmax to calculate voigt profile\nline_indices = hitran(1:size(hitran,1),1)>WNmin & hitran(1:size(hitran,1),1)<WNmax;\n\nline = double(hitran(line_indices, 1:size(hitran,2)));\n\n%Calculate temperature and pressure profile\nT0 = 273+25; % surface temperature\nT0 = 273+T0_C;\nT = T0-0.0065.*range; % set to match the sounding\n\n% pressure in atmospheres\nP0  = 0.83; % surface pressure\nP0  = P0_mb/1000*0.986; %pressure in mb converted to atm\nP = P0.*(T0./T).^-5.5;   % set this value to match sounding\n\nT00 = 296;              % HITRAN reference temperature [K]\nP00 = 1;                % HITRAN reference pressure [atm]\nnu0_0 = line(:,1);      % absorption line center wavenumber from HITRAN [cm^-1]\nS0 = line(:,2);         % initial linestrength from HITRAN [cm^-1/(mol*cm^-2)]   \ngammal0 = line(:,4);    % air-broadened halfwidth at T_ref and P_ref from HITRAN [cm^-1/atm]\ngamma_s = line(:,5);    % self-broadened halfwidth at T_ref and P_ref from HITRAN [cm^-1/atm]\nE = line(:,6);          % ground state transition energy from HITRAN [cm^-1]  \nalpha = line(:,7);      % linewidth temperature dependence factor from HITRAN\ndelta = line(:,8);      % pressure shift from HiTRAN [cm^-1 atm^-1]\n\nnu_on = 1/(lambda)*1e7;\nnu_off = 1/(lambda_off)*1e7;\n\nfor i = 1:size(Online,2); % calculate the absorption cross section at each range\n  \n    nu0 = nu0_0+delta.*(P(i)./P00); % unclear if it should be Pi/P00  \n    gammal = gammal0.*(P(i)./P00).*((T00./T(i)).^alpha);    %Calculate Lorentz lineweidth at P(i) and T(i)\n\n    const.m = 18.015E-3./6.022E23; % mass of a single water molecule\n    const.k_B = 1.3806488e-23; % (J/K)\n    const.c = 299792458; % (m/s) (exact)\n \n    gammad = (nu0).*((2.0.*const.k_B.*T(i).*log(2.0))./(const.m.*const.c^2)).^(0.5);  %Calculate HWHM Doppler linewidth at T(i)\n     \n    % term 1 in the Voigt profile\n    y = (gammal./gammad).*((log(2.0)).^(0.5));\n    \n    % term 2 in the Voigt profile\n    x_on = ((nu_on-nu0)./gammad).*(log(2.0)).^(0.5);\n    x_off = ((nu_off-nu0)./gammad).*(log(2.0)).^(0.5);\n    \n    %setting up Voigt convolution\n    t = (-(size(line,1))/2:1:size(line,1)/2-1); %set up the integration spectral step size\n    t = repmat(t',1,length(x_on))';\n    x_on = repmat(x_on,1,length(t));\n    x_off = repmat(x_off,1,length(t));\n    y = repmat(y,1,length(t));\n    f_on = (exp(-t.^2.0))./(y.^2.0+(x_on-t).^2.0);  % combined Voigt term 1 and 2\n    f_off = (exp(-t.^2.0))./(y.^2.0+(x_off-t).^2.0);\n    %Voigt integration over all of the lines at the on and offline locations\n    z_on = trapz(t(1,:),f_on,2);\n    z_off =  trapz(t(1,:),f_off,2);\n    integral_on = z_on;\n    integral_off = z_off;\n    %Calculate linestrength at temperature T\n    S = S0.*((T00./T(i)).^(1.5)).*exp(1.439.*E.*((1./T00)-(1./T(i))));\n \n    %Calculate the Voigt profile\n    K_on = (y(:,1)./pi).*integral_on;\n    K_off = (y(:,1)./pi).*integral_off;\n    \n    %Calculate the Voigt profile absorption cross section [cm^2]\n    sigmav_on = S.*(1./gammad).*(((log(2.0))./pi).^(0.5)).*K_on; %.*far_wing_on;\n    sigmav_off = S.*(1./gammad).*(((log(2.0))./pi).^(0.5)).*K_off; %.*far_wing_off;\n    \n    %Sum contributions from all of the surrounding lines\n    sigma_on_total(i) = sum(sigmav_on);\n    sigma_off_total(i) = sum(sigmav_off);\n    \nend;"("lambda"=w534, "lambda_off"=w537, "P0_mb"=w536, "T0_C"=w535, "Online"=w531) -> ("sigma_on_total"=→"sigma_on_total":dbl[], "sigma_off_total"=→"sigma_off_total":dbl[])  [unwired: 1 in, 1 out]
                  }
                }
              }
              frame #5 {
                w548 = 1
                # "normalization factor\nfrom 300 to 450m"
                # "OPTICAL DEPTH PLOT"
                # "new rainbow color bar display"
                # "Data Processing Far Channel"
                # "new rainbow color bar display"
                # "Calculating the range resolved water vapor number density and plotting"
                n416 = local read "sigma_off_total"() -> (w571:dbl[])
                n417 = local read "sigma_on_total"() -> (w568:dbl[])
                n418 = local read "On-Line  Smoothed"() -> (w546:dbl[])
                n419 = local read "Off-Line Smoothed"() -> (w545:dbl[])
                n420 = local read "Off-Line Smoothed 2"() -> (w569:dbl[])
                n421 = local read "On-Line Smoothed 2"() -> (w570:dbl[])
                n422 = script code="%Time averaging in seconds.  180 Seconds =3 minutes\ntemporal_average = 180;\n\n%Spatial averaging in bins.  2 bins = 150 meters\nspatial_average = 2;\n\n%Creating r and r+deltar vectors..this can also be acsomplished using the\n%diff command\np_oni = Online(:,1:size(Online,2)-1);\n\np_onii = Online(:,2:size(Online,2));\n\np_offi = Offline(:,1:size(Offline,2)-1);\n\np_offii = Offline(:,2:size(Offline,2));\n\nInside = (p_oni.*p_offii)./(p_onii.*p_offi);\n\ndel_cross = 1./(2.*(sigma_on_total(1:size(Online,2)-1)-sigma_off_total(1:size(Offline,2)-1)).*75*100);\n\ndel_cross(isinf(del_cross)) = 0;\n\n%Calculating Number density\nN = del_cross.*log(Inside);\n\n%Spatial smoothing of the profiles\nfilter1 = ones(1,2)./2;\n\nN_1 = N;\n\nN_1_avg = filter2(filter1,N_1);\n\nfilter1 = ones(1,10)./10;\n\nN_2 = N;\n\nN_2_avg = filter2(filter1,N_2);\n\nN_new = zeros(size(N,1),size(N,2));\n \n%Using different averaging windows for different altitudes \nN_avg=[N_1_avg(:,1:40)';N_2_avg(:,41:size(N,2))']';\n\n\nw = N_avg.*1e6.*18.015./6.022e23"("Online"=w570, "Offline"=w569, "sigma_on_total"=w568, "sigma_off_total"=w571) -> ("N_avg"=w572:cdb[], "w"=w581:cdb[])  [unwired: 1 in, 1 out]
                n423 = script code="%Time averaging in seconds.  180 Seconds = 3 minutes\ntemporal_average = 180;\n\n%Spatial averaging in bins.  2 bins = 150 meters\nspatial_average = 2;\n\n%Creating r and r+deltar vectors..this can also be acsomplished using the\n%diff command\np_oni = Online(:,1:size(Online,2)-1);\n\np_onii = Online(:,2:size(Online,2));\n\np_offi = Offline(:,1:size(Offline,2)-1);\n\np_offii = Offline(:,2:size(Offline,2));\n\nInside = (p_oni.*p_offii)./(p_onii.*p_offi);\n\ndel_cross = 1./(2.*(sigma_on_total(1:size(Online,2)-1)-sigma_off_total(1:size(Offline,2)-1)).*75*100);\n\ndel_cross(isinf(del_cross)) = 0;\n\n%Calculating Number density\nN = del_cross.*log(Inside);\n\n%Spatial smoothing of the profiles\nfilter1 = ones(1,2)./2;\n\nN_1 = N;\n\nN_1_avg = filter2(filter1,N_1);\n\nfilter1 = ones(1,10)./10;\n\nN_2 = N;\n\nN_2_avg = filter2(filter1,N_2);\n\nN_new = zeros(size(N,1),size(N,2));\n \n%Using different averaging windows for different altitudes \nN_avg=[N_1_avg(:,1:40)';N_2_avg(:,41:size(N,2))']';\n\n \nw = N_avg.*1e6.*18.015./6.022e23"("Online"=w546, "Offline"=w545, "sigma_on_total"=w568, "sigma_off_total"=w571) -> ("N_avg"=w577:cdb[], "w"=w578:cdb[])  [unwired: 1 in, 1 out]
                n424 = local read "Time Resolution Per Bin(ns)"() -> (w547:u32)
                n425 = local read "bins"() -> (w573:u32)
                n426 = local read "Altitude Array (km)"() -> (w543:dbl[])
                n427 = Build Array(w578, w581) -> (w584:cdb[][])
                n428 = To Double Precision Float(number=w547) -> (double precision float=w566:dbl)
                n429 = Reshape Array(w577, w548, w573) -> (w588:cdb[][])
                n430 = Reshape Array(w572, w548, w573) -> (w575:cdb[][])
                n431 = Multiply(x=0.15, y=w566) -> (x*y=w564:dbl)
                n432 = Build Array(w577, w572) -> (w582:cdb[][])
                n433 = Divide(x=300.0, y=w564) -> (x/y=w561:dbl)
                n434 = Divide(x=450.0, y=w564) -> (x/y=w560:dbl)
                n435 = Build Array(w543, w543) -> (w567:dbl[][])
                n436 = call "Convert to Dynamic Data5"("2D Array"=w584) -> ("Dynamic Data Type"=w583:dynamicdata)  [unwired: 3 in]
                n437 = call "Convert to Dynamic Data2"("2D Array"=w582) -> ("Dynamic Data Type"=w579:dynamicdata)  [unwired: 3 in]
                n438 = Divide(x=w588, y=1e+17) -> (x/y=→"Water Vapor Number Density":cdb[][])
                n439 = Divide(x=w575, y=1e+17) -> (x/y=→"Water Vapor Number Density 2":cdb[][])
                n440 = call "Convert to Dynamic Data6"("Array"=w543) -> ("Dynamic Data Type"=w544:dynamicdata)  [unwired: 3 in]
                n441 = To Long Integer(number=w561) -> (32bit integer=w559:i32)
                n442 = To Long Integer(number=w560) -> (32bit integer=w558:i32)
                n443 = call "Convert to Dynamic Data"("2D Array"=w567) -> ("Dynamic Data Type"=w580:dynamicdata)  [unwired: 3 in]
                n444 = call "Convert to Dynamic Data8"("2D Array"=w567) -> ("Dynamic Data Type"=w585:dynamicdata)  [unwired: 3 in]
                n445 = Decrement(x=w559) -> (x-1=w556:i32)
                n446 = Decrement(x=w558) -> (x-1=w557:i32)
                n447 = call "Build XY Graph"("Y Input"=w580, "X Input"=w579) -> ("XY Graph"=→"Water Vapor Number Density  2":cluster{"Y":dbl[], "Y":dbl[]}[])  [unwired: 3 in, 6 out]
                n448 = call "Build XY Graph3"("Y Input"=w585, "X Input"=w583) -> ("XY Graph"=→"Absolute Humidity":cluster{"Y":dbl[], "Y":dbl[]}[])  [unwired: 3 in, 6 out]
                n449 = Array Subset(array=w546, index=w556, length=w557) -> (w555:dbl[])
                n450 = Array Subset(array=w545, index=w556, length=w557) -> (w554:dbl[])
                n451 = call-poly <vilib>:"Mean.vi"("X"=w555) -> ("mean"=w553:dbl)  [unwired: 1 out]
                n452 = call-poly <vilib>:"Mean.vi"("X"=w554) -> ("mean"=w552:dbl)  [unwired: 1 out]
                n453 = Divide(x=w553, y=w552) -> (x/y=w551:dbl)
                n454 = Multiply(x=w545, y=w551) -> (x*y=w550:dbl[])
                n455 = Divide(x=w546, y=w550) -> (x/y=w549:dbl[])
                n456 = Natural Logarithm(1:w549) -> (0:w540:dbl[])
                n457 = Multiply(x=-1.0, y=w540) -> (x*y=w539:dbl[])
                n458 = call "Convert to Dynamic Data9"("Array"=w539) -> ("Dynamic Data Type"=w542:dynamicdata)  [unwired: 3 in]
                n459 = call "Build OD Plot"("Y Input"=w544, "X Input"=w542) -> ("XY Graph"=→"Optical Depth":cluster{"Y":dbl[], "Y":dbl[]}[])  [unwired: 3 in, 6 out]
              }
            }
          }
        }
        "L_Count" <- w95
      }
    }
  }
  n460 = case shown="True" w3 {
    frame False {
    }
    frame True {
      # "close data files"
      # "Close Bristol WM"
      n461 = local read "Ophir PM On/Off"() -> (w592:bool)
      n462 = local read "Bristol Out"() -> (w597:i32)
      n463 = local read "NF_Off_Ref"() -> (w593:refnum<file>)
      n464 = local read "NF_On_Ref"() -> (w594:refnum<file>)
      n465 = local read "FF_Off_Ref"() -> (w595:refnum<file>)
      n466 = local read "WS_On/Off"() -> (w591:bool)
      n467 = local read "FF_On_Ref"() -> (w596:refnum<file>)
      n468 = case shown="True" w591 {
        frame False {
        }
        frame True {
          n469 = local read "WS visa"() -> (w600:refnum<visa-resource-name>)
          n470 = call "T_RH_P.vi"("VISA in"=w600, "WS_Commands"=enum16{"OpenWS", "ReadTRHP", "CloseWS"}."CloseWS") -> ()  [unwired: 11 in, 3 out]
        }
      }
      n471 = case shown="True" w592 {
        frame False {
        }
        frame True {
          n472 = local read "OphirPM"() -> (w598:T7)
          n473 = call "OphirClose.vi"("OphirPM"=w598) -> ()  [unwired: 18 in, 1 out]
        }
      }
      n474 = dll-call lib="C:/H2O_DIAL/LabVIEW-2012/Bristol WM V2_31b/CLDevIFace.dll" fn="CLCloseDevice"("CommPort"=w597) -> ()  [unwired: 5 in, 2 out]
      n475 = Close File(refnum=w596) -> ()  [unwired: 1 in, 2 out]
      n476 = Close File(refnum=w595) -> ()  [unwired: 1 in, 2 out]
      n477 = Close File(refnum=w594) -> ()  [unwired: 1 in, 2 out]
      n478 = Close File(refnum=w593) -> ()  [unwired: 1 in, 2 out]
    }
  }
  "FileHour" <- -1 ("FileHour")
  "DataOpen" <- FALSE
